vi "main_scan_5_Zeitsequenzen.vi"() -> ()   [LabVIEW 2009]
uses:
  <vilib>/userdefined/High Color/IMAQdx.ctl
  <vilib>/vision/Image Controls.llb/IMAQ Image.ctl
  global_stage_initialised.vi
  <vilib>/vision/driver/IMAQdx.llb/IMAQdx Buffer Number Mode.ctl
  <vilib>/Utility/file.llb/Write To Spreadsheet File (DBL).vi
  <vilib>/vision/driver/NI_Vision_Acquisition_Software.lvlib
  Program Files (x86)/National Instruments/LabVIEW 2009/resource/objmgr/imaqdx.rc
panel:
  in  "Log-Plot":bool
  in  "Video Mode":u32(ring)=2 items=["Mono 8 1.88 fsp", "Mono 8 3.75 fsp", "Mono 8 7.50 fsp", "Mono 8 15.00 fsp", "Mono 8 30.00 fsp", "Mono 8 60.00 fsp", "Mono 8 120.00 fsp", "Mono 16 1.88 fsp", "Mono 16 3.75 fsp", "Mono 16 7.50 fsp", "Mono 16 15.00 fsp", "Mono 16 30.00 fsp", "Mono 16 60.00 fsp", "Format 7 Mode 0 640x480"]
  out "Vektor Summierte Helligkeit [a.u.]":dbl[](array[numeric])
  out "Vektor L/2-Position [°]":dbl[](array[numeric])
  out "Daten speichern":bool
  out "Leist/Pol # Schleifen":i64
  out "Leistungs-/Polarisationscan läuft":bool
  in  "Max. Spannungsdifferenz":dbl=150.0
  out "Geschätzte Messzeit":string="00:00"
  out "Start time [ms]":timestamp
  out "2D-Intensitätsverteilung (MCP)":dbl[][](graph)
  in  "# Photosignale":i32
  in  "Achs-ID":i32
  in  "Spannungskanal":refnum<k21>
  out "x-U-Scan läuft":bool
  out "Spannungsscan läuft":bool
  out "LAPD Spannung (V)":dbl format="%#.3g"
  out "Summierte Helligkeit (a.u.)":i64
  out "# Messschritte":i32
  out "Aktueller Messschritt":i32
  in  "LAPD-Daten speichern":bool
  in  "Summierte Helligkeit speichern":bool
  in  "Einzelbilder speichern":bool
  in  "Gemittelte Bilder speichern":bool
  in  "# Bilder/Messschritt":i32=1
  in  "SN von Rotationsbühne":i32=83831982
  in  "Wellenplatte [°]":refnum<k7>(container)
  out "Wellenplatte":bool
  in  "Waveplate ON/OFF":bool
  in  "Registerkarte":T1(tab)=enum."Sequenzaufnahme"
  out "Aktuelle xyz-Position [mm]":dbl[](array[numeric]) format="%.5g"
  in  "Rasterweite [µm]":dbl[](array[numeric])
  in  "# Rasterschritte":i32[](array[numeric])=[1, 1, 1] min=1 step=1
  in  "Rasterung ON/OFF":bool
  out "Start xyz-Position [mm]":dbl[](array[numeric]) format="%.5g"
  in  "Rasterart":T2(ring)=enum."2D-Scan(xy)"
  out "Rasterschritt [µm]":dbl[](array[numeric])
  out "2D-Intensitätsverteilung (LAPD)":dbl[][](graph)
  out "Spannungsstart [V]":dbl[](array[numeric])
  out "TIP/SUP":string[](array[string])=["Tip", "Suppressor"]
  out "Spannungsschritt [V]":dbl[](array[numeric]) format="%.1g"
  out "Aktuelle Spannung [V]":dbl[](array[numeric]) format="%.1f"
  in  "# Spannungsschritte":i32[](array[numeric])
  in  "Spannungsweite [V]":dbl[](array[numeric])
  in  "Spannungsscan ON/OFF":bool
  out "Schräglage berücksichtigen":string="Schräglage berücksichtigen"
  in  "Ausgleichslage Start festlegen":bool
  out "x-U-Scan (Ausgleichslage) xy-Start [mm]":dbl[](array[numeric]) format="%_5g"
  in  "Raum-Koordinate 2 (Lagenausgleich)":enum16{"x-Achse", "y-Achse", "z-Achse"}(ring)=enum."y-Achse"
  out "x-U-Scan y-Startposition [mm]":dbl format="%.4g"
  out "x-U-Scan aktuelle y-Position [mm]":dbl format="%.4g"
  in  "x-U-Scan (Ausgleichslage) Steigung":dbl format="%_3g"
  out "x-U-Scan Spannungsstart [V]":dbl
  out "x-U-Scan Spannungsschritt [V]":dbl
  out "x-U-Scan aktuelle Spannung [V]":dbl
  in  "# x-U-Scan Spannungsschritte":i32
  in  "x-U-Scan Spannungsweite [V]":dbl
  in  "Raum-Koordinate 1":enum16{"x-Achse", "y-Achse", "z-Achse"}(ring)
  in  "Spannungs-Koordinate":enum16{"Tip-Spannung", "Suppressor-Spannung"}(ring)=2
  in  "x-U-Scan ON/OFF":bool
  in  "x-U-Scan x-Rasterweite [µm]":dbl
  in  "# x-U-Scan x-Rasterschritte":i32
  out "x-U-Scan x-Startposition [mm]":dbl format="%.4g"
  out "x-U-Scan aktuelle x-Position [mm]":dbl format="%.4g"
  out "x-U-Scan x-Rasterschritt [µm]":dbl
  out "x-U-Scan (Ausgleichslage) xy-End [mm]":dbl[](array[numeric]) format="%_5g"
  in  "Ausgleichslage Ende festlegen":bool
  in  "Sättigungszeit [s]":dbl
  in  "Wartezeit [s]":dbl
  in  "Max. Leistung (vK) [mW]":dbl
  out "Aktuelle Leistung (iK) [mW]":dbl
  out "Aktuelle L/2-Position [°]":dbl format="%_3g"
  out "L/2-Schritt [°]":dbl
  in  "Hin und Zurück":bool=TRUE
  in  "# L/2-Schritte":i32
  in  "L/2-Weite [°]":dbl
  in  "L/2-Start [°]":dbl
  in  "Leistuns- oder Polarisationsscan":u16(ring) items=["Polarisationsscan", "Leistungsscan"]
  in  "Leistungs-/Polarisationsscan ON/OFF":bool
  out "1D-Intensitätsverteilung (MCP)":T3(graph)
  out "Vorherige L/2 Position [°]":dbl format="%_3g"
  out "Gesamtzeit [min]":dbl format="%#.2g"
  in  "# Messpunkte":i32=1
  in  "Verzögerung [s]":i64
  in  "Hintergrund-Helligkeit":i64
  in  "Helligkeit nullen":bool
  out "Helligkeitsverlauf":dbl(graph)
  in  "Sequenz Ordner":string="Referenzbilder"
  in  "Sequenzaufnahme ON":bool
  out "LAPD (a.u.)":dbl(graph)
  in  "MCP-Spannung [V]":dbl=1300.0
  in  "P-Schirm-Spannung [V]":dbl=4300.0
  in  "Proben-ID":string="140528_06"
  out "Messlogbuch":path
  out "Gemitteltes Bild":u64[][](array[numeric])
  in  "Polarisation [°]":dbl=90.0
  out "Current y step":i32
  out "Current z step":i32
  out "Current x step":i32
  out "Scanschleifenzähler":i32
  out "Kameraschleifenzähler":i32
  out "Steuerschleifenzähler":i32
  out "Bühne":bool
  in  "HV ON/OFF":bool
  out "HV-Steuerung":bool
  in  "Suppressor-Spannung [V]":dbl min=0.0 max=300.0 step=1.0 format="%.1p"
  in  "Tip-Spannung [V]":dbl min=0.0 max=300.0 step=1.0 format="%.1p"
  in  "Leistung (iK) [mW]":dbl format="%.1f"
  in  "LAPD-Kanal (Meilhaus)":u32 max=31
  out "Save folder":string
  out "Buffer Number":u64
  out "ROI table":string[](array[string])=["Breite [px]", "Höhe [px]", "X-Offset [px]", "Y-Offset [px]"]
  in  "Vollbild":bool
  out "Frame Rate (FPS)":dbl format="%#_3g"
  in  "Buffer Interval":u32=1
  out "Ereignis: FrameDone?":refnum<event-registration>
  out "Image Display":T4(plugin-control)
  in  "ROI":i32[](array[numeric])=[640, 480, 0, 0]
  in  "Shutter time (ms)":u16(ring)=3 items=["1000", "500", "200", "100", "50", "20", "10", "1"]
  out "Buffer Overrun":bool
  out "Image Memory":T4
  out "Kamera":bool
  in  "Kamera ON/OFF":bool
  in  "Detektionskamera":T5="cam0"
  out "Day folder":string
  in  "Root folder":string="D:\\Michael Lohmann\\Messungen\\"
  out "z-Achse":i32=3
  out "y-Achse":i32=2
  out "x-Achse":i32=1
  out "Event: Rasterung gestartet?":refnum<user-event>
  out "Fehler (Ausgang)":errorcluster
  in  "Programm beenden":bool
  out "Rasterung läuft":bool
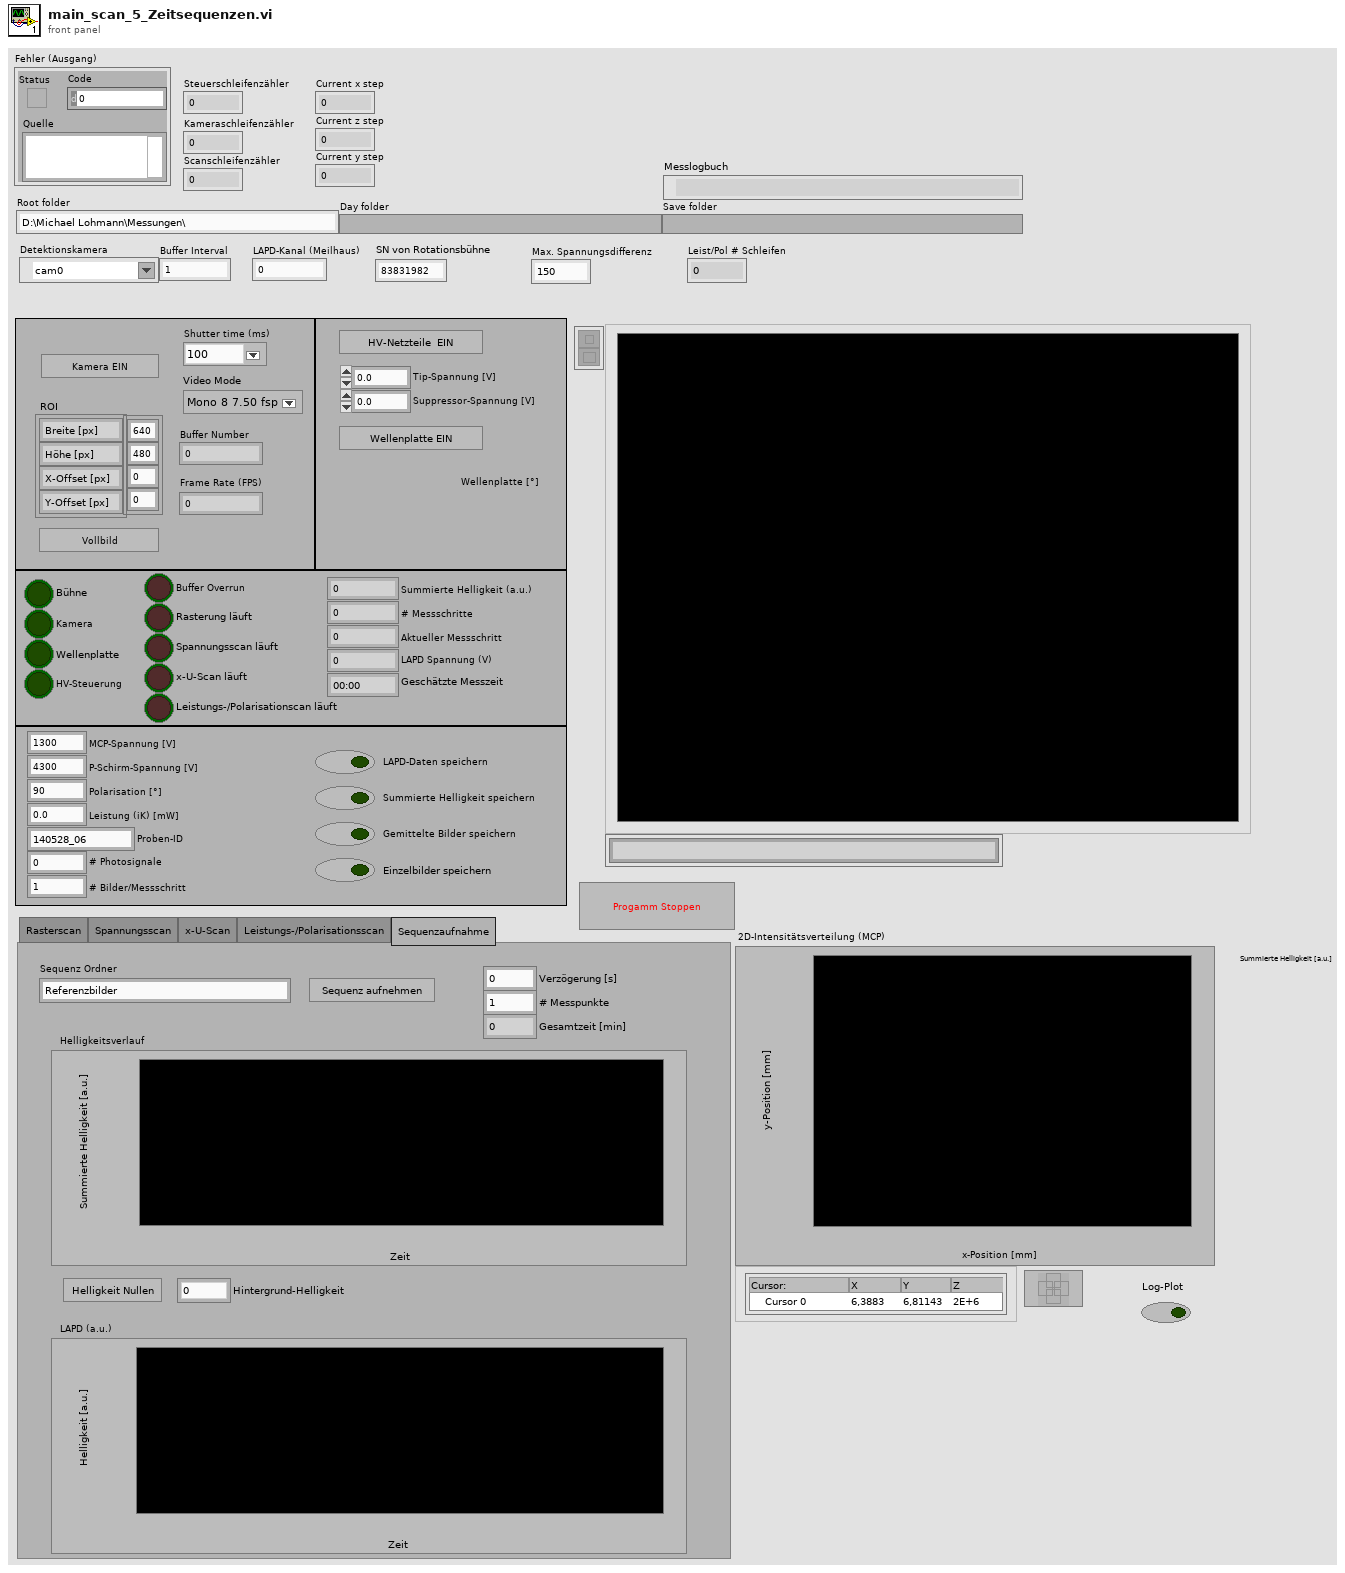
[diagram p1: front panel]
types:
  T1 = enum32{"Rasterscan", "Spannungsscan", "x-U-Scan", "Leistungs-/Polarisationsscan", "Sequenzaufnahme"}
  T2 = enum16{"Linescan(x)", "Linescan(z)", "2D-Scan(xy)", "2D-Scan(yz)", "2D-Scan(xz)"}
  T3 = cluster{"Vektor L/2-Position [°]":dbl[], "Vektor Summierte Helligkeit [a.u.]":dbl[]}
  T4 = typedef "IMAQ Image.ctl" = refnum<image>
  T5 = typedef "IMAQdx.ctl" = refnum<k21>
  T6 = enum32{"Bad", "Idle", "Run top level", "Running"}
  T7 = cluster{"Summierte Helligkeit (a.u.)":u64, "Aktuelle L/2-Position [°]":dbl}
  T8 = typedef "NI_Vision_Acquisition_Software.lvlib/IMAQdx Buffer Number Mode.ctl" = enum32{"Next", "Last", "Buffer Number"}
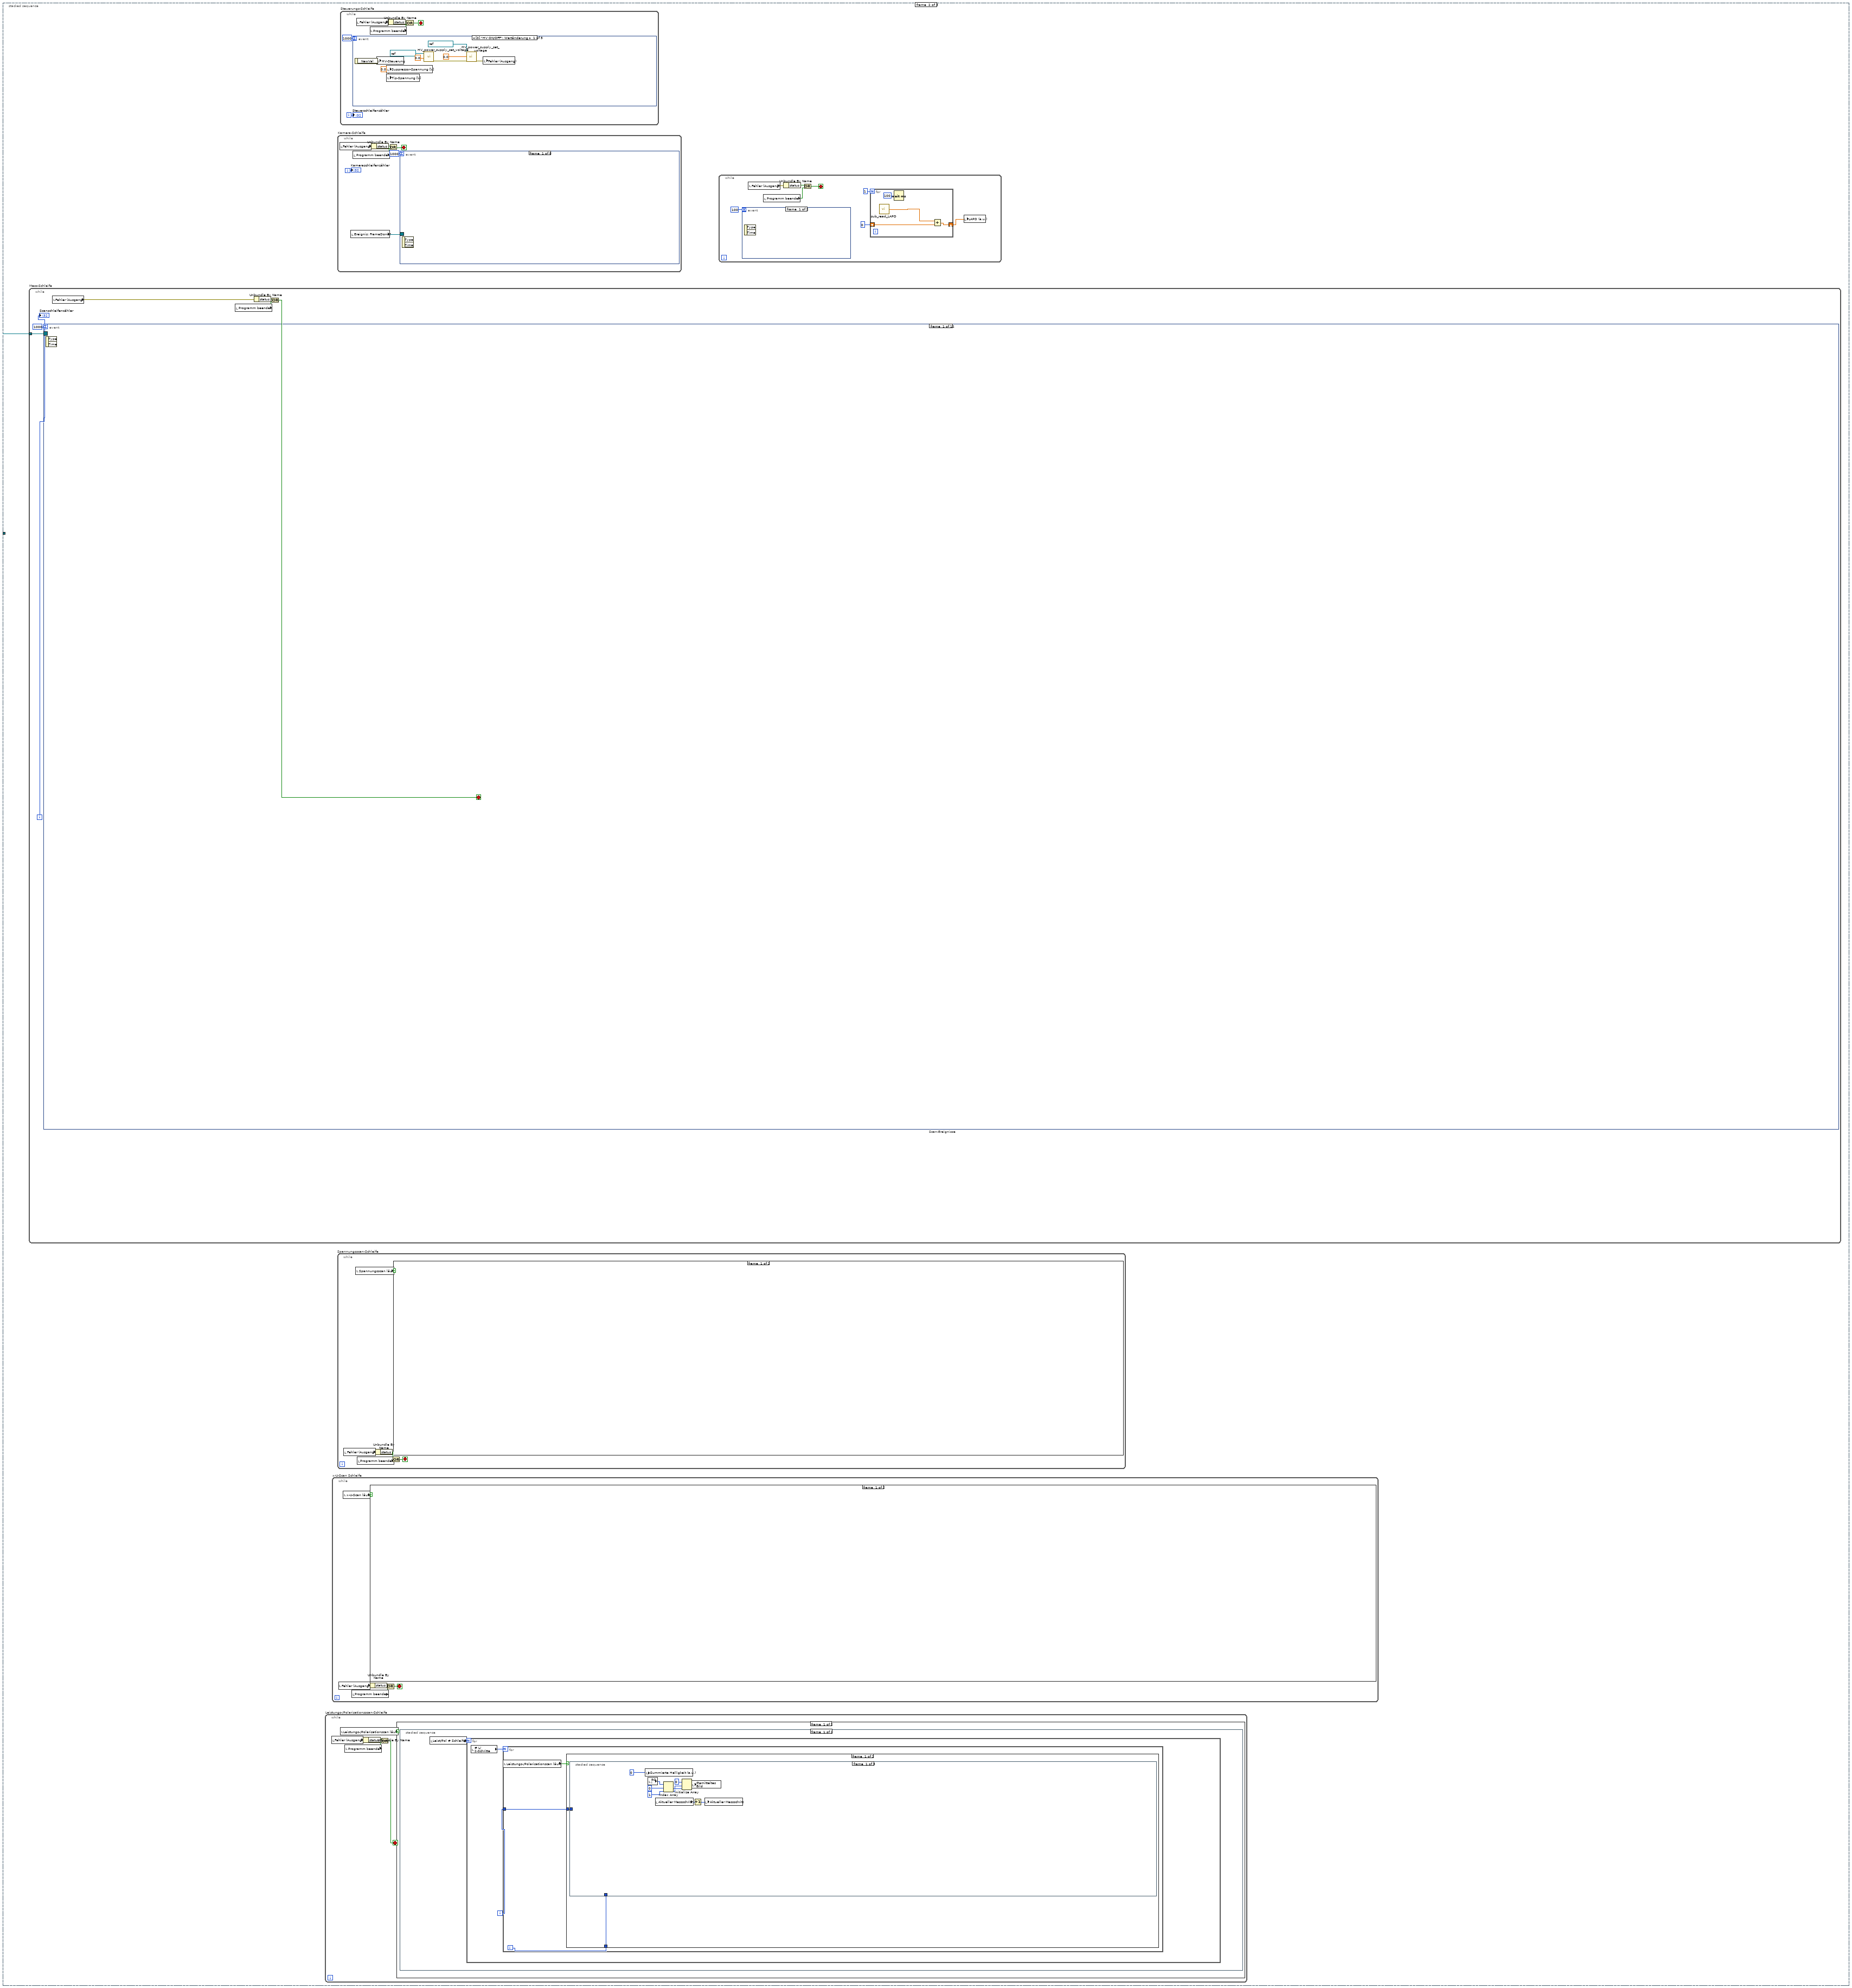
[diagram p3: hidden frame]
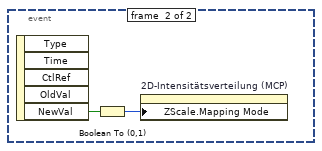
[diagram p4: hidden frame]
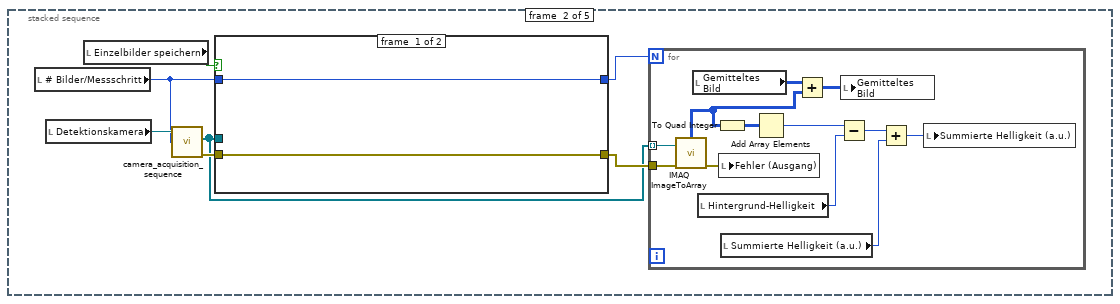
[diagram p5: hidden frame]
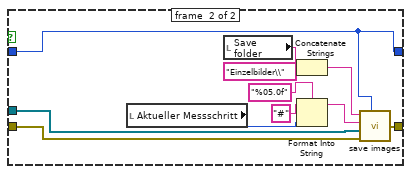
[diagram p6: hidden frame]
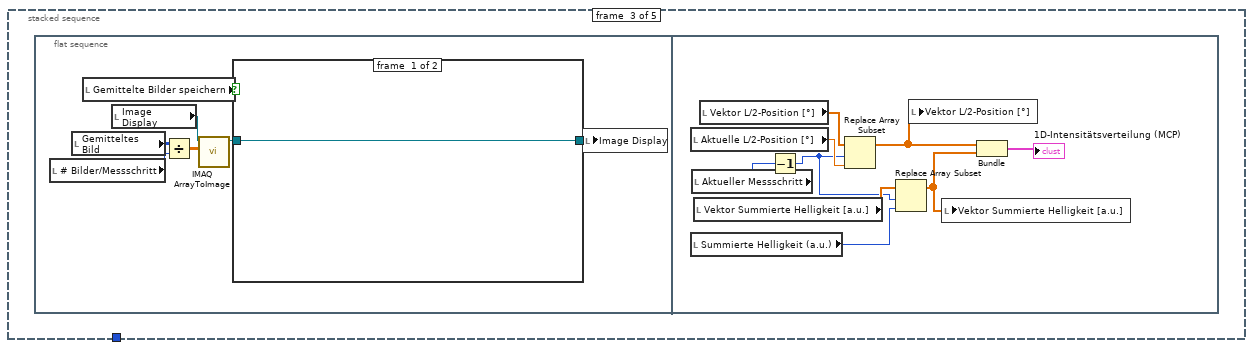
[diagram p7: hidden frame]
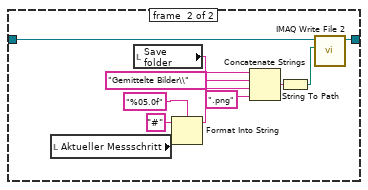
[diagram p8: hidden frame]
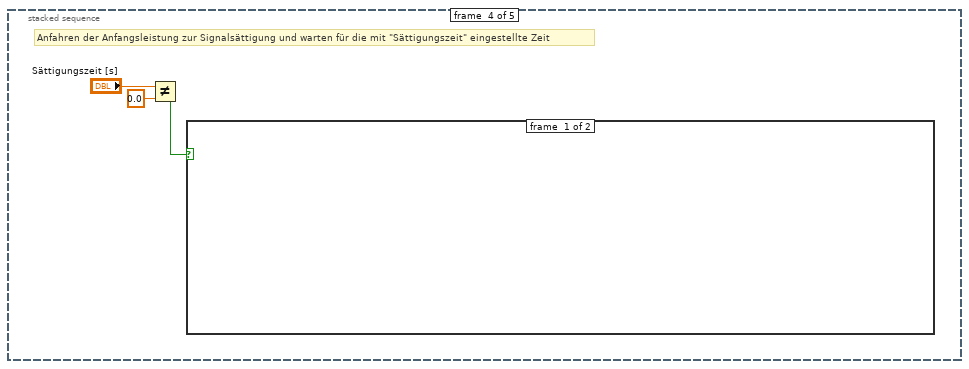
[diagram p9: hidden frame]
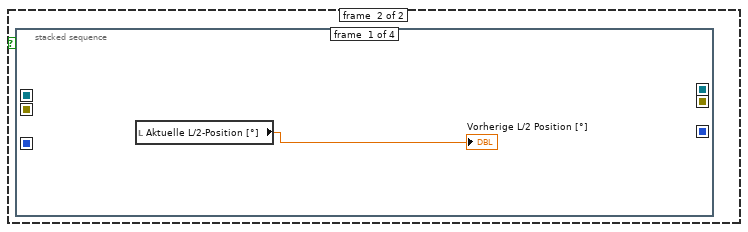
[diagram p10: hidden frame]
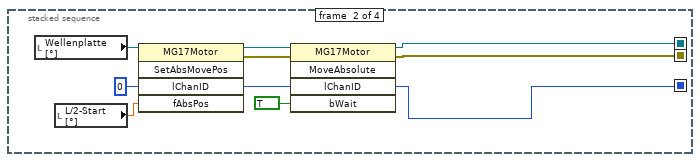
[diagram p11: hidden frame]
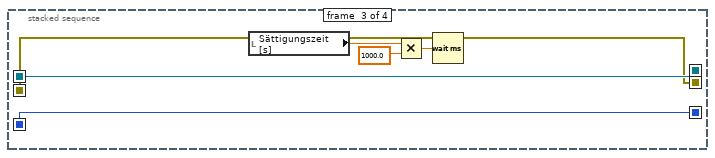
[diagram p12: hidden frame]
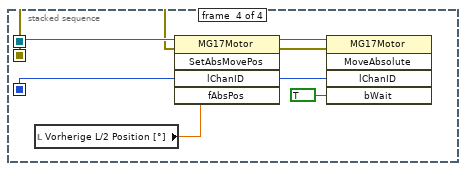
[diagram p13: hidden frame]
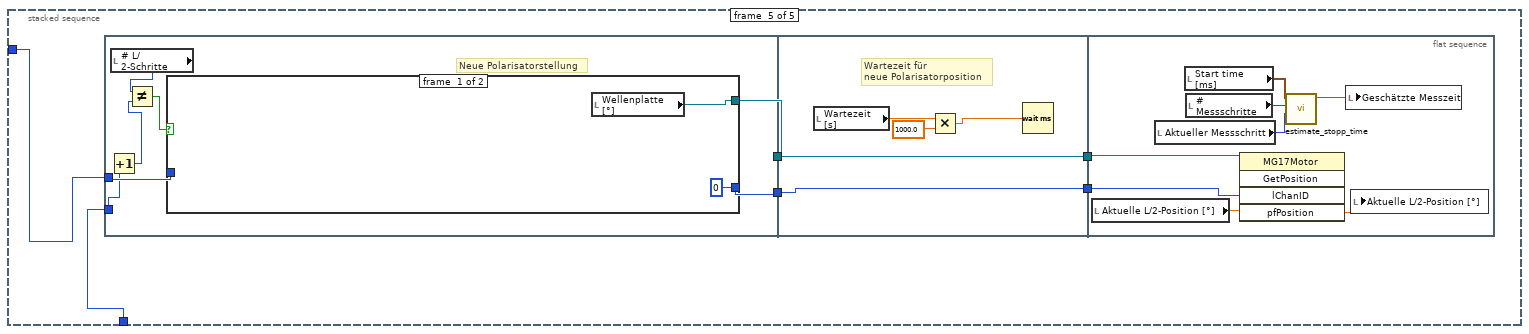
[diagram p14: hidden frame]
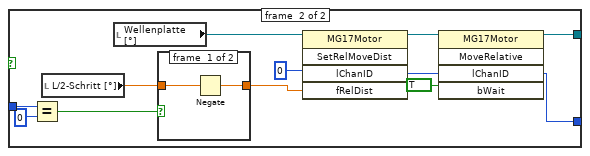
[diagram p15: hidden frame]
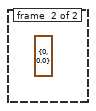
[diagram p17: hidden frame]
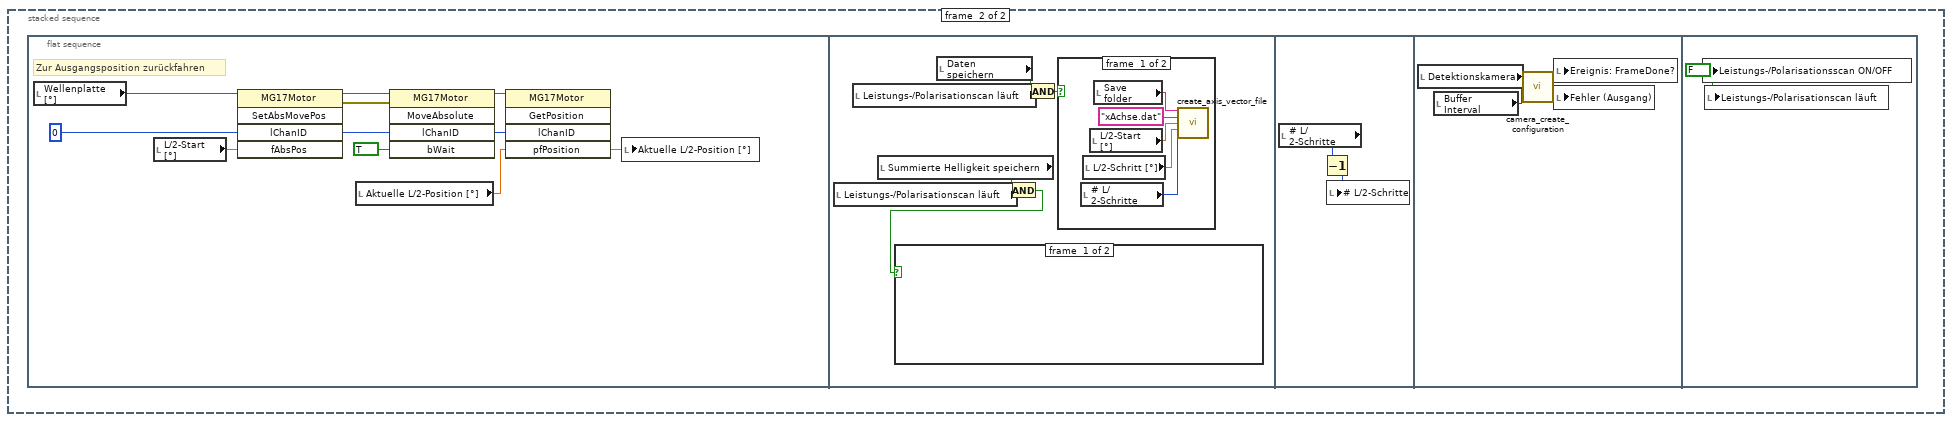
[diagram p18: hidden frame]
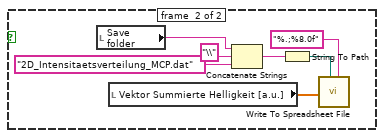
[diagram p19: hidden frame]
diagram:
  n1 = local read "Event: Rasterung gestartet?"() -> (w2:refnum<user-event>)
  n2 = register-events(w2) -> (reference out=w1:refnum<event-registration>)  [unwired: 2 in, 1 out]
  n3 = stacked-sequence {
    tunnel: w1 -> [_ w27 _]
    frame #0 {
      n4 = flat-sequence {
        frame #0 {
          # "Überprüfung ob die VI stage_control.vi ausgeführt wid, wenn nicht wird sie gestartet und gewartet bis die Bühne initialisiert ist"
          n5 = Open VI Reference(vi path=path "stage_control_mit_speichern.vi" ("VI-Pfad")) -> (vi reference=w5:refnum<vi>)  [unwired: 5 in, 1 out]
          n6 = property class="VI"(reference=w5) -> (reference out=w4:refnum<vi>, error out=w3:errorcluster, "Exec.State"=w8:T6)  [unwired: 1 in]
          n7 = Equal?(x=w8, y=T6."Run top level") -> (x = y?=w6:bool)
          n8 = case shown="False" w6 {
            tunnel: w4 -> [w15 _]
            tunnel: w3 -> [w14 _]
            frame #0 {
              n9 = invoke class="VI" method="VI ausführen"(reference=w15, error in=w14, "Wait until done"=FALSE ("Warten bis beendet"), "Auto Dispose Ref"=FALSE ("Referenz automatisch schließen")) -> (reference out=w11:refnum<vi>)  [unwired: 1 in, 4 out]
              n10 = invoke class="VI" method="FP.Öffnen"(reference=w11) -> (reference out=w10:refnum<vi>)  [unwired: 4 in, 4 out]
              n11 = while {
                tunnel: w10 -> [w22]
                stop <- w17 stop-if-true
                n12 = property class="VI"(reference=w22) -> (error out=w21:errorcluster, "Exec.State"=w20:T6)  [unwired: 1 in, 1 out]
                n13 = global read "global_stage_initialised.vi" "Bühne initialisiert"() -> (w16:bool)
                n14 = local write "Fehler (Ausgang)"(w21) -> ()
                n15 = Equal?(x=w20, y=T6."Run top level") -> (x = y?=w18:bool)
                n16 = And(x=w16, y=w18) -> (x .and. y?=w17:bool)
              }
            }
            frame #1 {
            }
          }
        }
        frame #1 {
          n17 = local read "Root folder"() -> (w26:string)
          n18 = local write "Bühne"(TRUE ("Bühne bereit")) -> ()
          n19 = call "create_day_folder.vi"("Root folder"=w26) -> ("Day Folder"=w24:string)  [unwired: 9 in, 1 out]
          n20 = local write "Day folder"(w24) -> ()
          n21 = call "create_measure_log_file.vi"("Tagesordner"=w24) -> ("Messlogbuch"=w23:path)  [unwired: 9 in]
          n22 = local write "Messlogbuch"(w23) -> ()
        }
      }
    }
    frame #1 {
      n23 = while "Mess-Schleife" {
        tunnel: w27 -> [w644]
        i -> [w643]
        stop <- w642 stop-if-true
        n24 = event "Scan-Ereignisse" shown="[3] <Event: Rasterung gestartet?>: Benutzerereignis" {
          selector: w644 -> [_ _ _ _ _ _ _ _ _ _ _]
          dyn-events: _ -> [_ _ _ _ _ _ _ _ _ _ _]
          timeout: 1000 -> [_ _ _ _ _ _ _ _ _ _ _]
          event #0 {
            n25 = event-data() -> ()  [unwired: 1 in, 2 out]
          }
          event #1 {
            n26 = event-data() -> ("NewVal"=w651:bool)  [unwired: 1 in]
            n27 = local read "Kamera"() -> (w649:bool)
            n28 = case shown="False" w649 {
              frame #0 {
                n29 = local write "Rasterung ON/OFF"(FALSE ("Rasterung ON/OFF")) -> ()
                n30 = One Button Dialog(message="Kamera aus" ("Nachricht")) -> ()  [unwired: 1 in, 1 out]
              }
              frame #1 {
              }
            }
            n31 = And(x=w649, y=w651) -> (x .and. y?=w650:bool)
            n32 = case shown="True" w650 {
              frame #0 {
                n33 = local write "Rasterung läuft"(FALSE ("Rasterung läuft")) -> ()
              }
              frame #1 {
                n34 = stacked-sequence {
                  frame #0 {
                    n35 = stacked-sequence {
                      seq-local: [w664 _] -> [_ w727]
                      frame #0 {
                        n36 = local read "Rasterart"() -> (w678:T2)
                        n37 = local read "Rasterweite [µm]"() -> (w675:dbl[])
                        n38 = local read "# Rasterschritte"() -> (w677:i32[])
                        n39 = Get Date/Time In Seconds() -> (seconds since 1Jan1904=w655:timestamp)
                        n40 = local write "Start time [ms]"(w655) -> ()
                        n41 = case shown="\"2D-Scan(xz)\"" w678 {
                          tunnel: w677 -> [w686 w702 w707 w716 w722]
                          tunnel: [w685 w701 w708 w715 w719] -> w676
                          tunnel: w675 -> [w684 w692 w704 w712 w721]
                          tunnel: [w683 w691 w703 w711 w720] -> w674
                          frame #0 {
                            n42 = Replace Array Subset(array=w686, new element #1=1 ("Neues Element/Teil-Array"), index #1=1 ("Index"), new element #2=1 ("Neues Element/Teil-Array"), index #2=2 ("Index")) -> (w685:i32[])
                            n43 = Replace Array Subset(array=w684, new element #1=0.0 ("Neues Element/Teil-Array"), index #1=1 ("Index"), new element #2=0.0 ("Neues Element/Teil-Array"), index #2=2 ("Index")) -> (w683:dbl[])
                          }
                          frame #1 {
                            n44 = Replace Array Subset(array=w702, new element #1=1 ("Neues Element/Teil-Array"), index #1=0 ("Index"), new element #2=1 ("Neues Element/Teil-Array"), index #2=1 ("Index")) -> (w701:i32[])
                            n45 = Replace Array Subset(array=w692, new element #1=0.0 ("Neues Element/Teil-Array"), index #1=0 ("Index"), new element #2=0.0 ("Neues Element/Teil-Array"), index #2=1 ("Index")) -> (w691:dbl[])
                          }
                          frame #2 {
                            n46 = Replace Array Subset(array=w707, new element=1 ("Neues Element/Teil-Array"), index=2 ("Index")) -> (w708:i32[])
                            n47 = Replace Array Subset(array=w704, new element=0.0 ("Neues Element/Teil-Array"), index=2 ("Index")) -> (w703:dbl[])
                          }
                          frame #3 {
                            n48 = Replace Array Subset(array=w716, new element=1 ("Neues Element/Teil-Array"), index=0 ("Index")) -> (w715:i32[])
                            n49 = Replace Array Subset(array=w712, new element=0.0 ("Neues Element/Teil-Array"), index=0 ("Index")) -> (w711:dbl[])
                          }
                          frame #4 {
                            n50 = Replace Array Subset(array=w722, new element=1 ("Neues Element/Teil-Array"), index=1 ("Index")) -> (w719:i32[])
                            n51 = Replace Array Subset(array=w721, new element=0.0 ("Neues Element/Teil-Array"), index=1 ("Index")) -> (w720:dbl[])
                          }
                        }
                        n52 = local write "# Rasterschritte"(w676) -> ()
                        n53 = local write "Rasterweite [µm]"(w674) -> ()
                        n54 = control-ref of="Rasterart"() -> (w673:refnum<vi>)
                        n55 = property class="Enum (strikt)"(reference=w673) -> ("RingText.Text"=w659:string)  [unwired: 1 in, 2 out]
                        n56 = control-ref of="Shutter time (ms)"() -> (w672:refnum<vi>)
                        n57 = property class="Ring (strikt)"(reference=w672) -> ("RingText.Text"=w671:string)  [unwired: 1 in, 2 out]
                        n58 = local read "# Bilder/Messschritt"() -> (w670:i32)
                        n59 = local read "Suppressor-Spannung [V]"() -> (w657:dbl)
                        n60 = local read "P-Schirm-Spannung [V]"() -> (w662:dbl)
                        n61 = local read "MCP-Spannung [V]"() -> (w661:dbl)
                        n62 = local read "Leistung (iK) [mW]"() -> (w660:dbl)
                        n63 = local read "Tip-Spannung [V]"() -> (w656:dbl)
                        n64 = Decimal String To Number(string=w671) -> (number=w668:i32)  [unwired: 2 in, 1 out]
                        n65 = local read "Polarisation [°]"() -> (w665:dbl)
                        n66 = local read "Messlogbuch"() -> (w667:path)
                        n67 = local read "Proben-ID"() -> (w666:string)
                        n68 = Multiply(x=w670, y=w668) -> (x*y=w669:i32)
                        n69 = local read "ROI"() -> (w658:i32[])
                        n70 = call "stage_get_current_xyz.vi"() -> ("Aktuelle xyz-Position OUT [mm]"=w663:dbl[])  [unwired: 3 in, 1 out]
                        n71 = call "create_measure_log_entry.vi"("Messlogbuch-Pfad"=w667, "Probe"=w666, "Polarisation [°]"=w665, "Messart"=w659, "ROI"=w658, "Messungen/Messschritt"=w670, "Maximalleistung (iK) [mW]"=w660, "Tip-Spannung [V]"=w656, "Suppressor-Spannung [V]"=w657, "Zeit/Messschritt [ms]"=w668, "MCP-Spannung [V]"=w661, "Zeit/Messung [ms]"=w669, "Phosphorschirm-Spannung [V]"=w662, "xyz [mm]"=w663) -> ("Messung Nr."=w664:i32)  [unwired: 4 in, 1 out]
                      }
                      frame #1 {
                        n72 = local read "Summierte Helligkeit speichern"() -> (w731:bool)
                        n73 = local read "Gemittelte Bilder speichern"() -> (w729:bool)
                        n74 = local read "LAPD-Daten speichern"() -> (w728:bool)
                        n75 = local read "Einzelbilder speichern"() -> (w730:bool)
                        n76 = local read "Rasterweite [µm]"() -> (w758:dbl[])
                        n77 = local read "# Rasterschritte"() -> (w757:i32[])
                        n78 = local read "# Rasterschritte"() -> (w755:i32[])
                        n79 = Divide(x=w758, y=w757) -> (x/y=w756:dbl[])
                        n80 = Compound Arithmetic op=OR(w729, w730, w731, w728) -> (w732:bool)
                        n81 = local read "Kamera"() -> (w744:bool)
                        n82 = Index Array(array=w755, index #1=0 ("Index"), index #2=1 ("Index"), index #3=2 ("Index")) -> (element #1=w752:i32, element #2=w751:i32, element #3=w750:i32)
                        n83 = local write "Rasterschritt [µm]"(w756) -> ()
                        n84 = local write "Daten speichern"(w732) -> ()
                        n85 = local read "Fehler (Ausgang)"() -> (w733:errorcluster)
                        n86 = local write "Aktueller Messschritt"(0 ("Aktueller Messschritt")) -> ()
                        n87 = Multiply(x=w752, y=w751) -> (x*y=w749:i32)
                        n88 = local read "Day folder"() -> (w738:string)
                        n89 = local read "Einzelbilder speichern"() -> (w741:bool)
                        n90 = Multiply(x=w749, y=w750) -> (x*y=w748:i32)
                        n91 = local write "# Messschritte"(w748) -> ()
                        n92 = call "create_save_folder.vi"("Day folder"=w738, "Measuring number"=w727, "Measuring folder"="Rasterung" ("Subfolder"), "error in"=w733) -> ("Save Folder"=w737:string, "Error Out"=w736:errorcluster)  [unwired: 5 in]
                        n93 = local write "Save folder"(w737) -> ()
                        n94 = case shown="True" w741 {
                          tunnel: w736 -> [w759 w761]
                          tunnel: [w759 w760] -> w735
                          frame #0 {
                          }
                          frame #1 {
                            n95 = local read "Save folder"() -> (w764:string)
                            n96 = Concatenate Strings(w764, "\\Einzelbilder" ("Subfolder")) -> (w762:string)
                            n97 = String To Path(string=w762) -> (path=w765:path)
                            n98 = call <vilib>:"Check if File or Folder Exists.vi"("error in (no error)"=w761, "path"=w765) -> ("error out"=w760:errorcluster, "file or folder exists?"=w766:bool, "dup path"=w767:path)  [unwired: 7 in]
                            n99 = case shown="False" w766 {
                              tunnel: w767 -> [w768 _]
                              frame #0 {
                                n100 = Create Folder(path (use dialog)=w768) -> ()  [unwired: 2 in, 3 out]
                              }
                              frame #1 {
                              }
                            }
                          }
                        }
                        n101 = local read "Gemittelte Bilder speichern"() -> (w742:bool)
                        n102 = case shown="True" w742 {
                          tunnel: w735 -> [w769 w771]
                          tunnel: [w769 w770] -> w734
                          frame #0 {
                          }
                          frame #1 {
                            n103 = local read "Save folder"() -> (w775:string)
                            n104 = Concatenate Strings(w775, "\\Gemittelte Bilder" ("Subfolder")) -> (w777:string)
                            n105 = String To Path(string=w777) -> (path=w774:path)
                            n106 = call <vilib>:"Check if File or Folder Exists.vi"("error in (no error)"=w771, "path"=w774) -> ("error out"=w770:errorcluster, "file or folder exists?"=w773:bool, "dup path"=w772:path)  [unwired: 7 in]
                            n107 = case shown="False" w773 {
                              tunnel: w772 -> [w778 _]
                              frame #0 {
                                n108 = Create Folder(path (use dialog)=w778) -> ()  [unwired: 2 in, 3 out]
                              }
                              frame #1 {
                              }
                            }
                          }
                        }
                        n109 = case shown="True" w744 {
                          tunnel: [w779 w781] -> w743
                          tunnel: w734 -> [w779 w780]
                          frame #0 {
                          }
                          frame #1 {
                            n110 = local read "Ereignis: FrameDone?"() -> (w782:refnum<event-registration>)
                            n111 = local read "Detektionskamera"() -> (w783:T5)
                            n112 = call "camera_release_configuration.vi"("error in"=w780, "Session In"=w783, "Ereignisregistrierung (Referenz) 2"=w782) -> ("error out"=w781:errorcluster)  [unwired: 1 out]
                          }
                        }
                        n113 = call "stage_get_current_xyz.vi"("error in"=w743) -> ("error out"=w740:errorcluster, "Aktuelle xyz-Position OUT [mm]"=w745:dbl[])  [unwired: 2 in]
                        n114 = local write "Start xyz-Position [mm]"(w745) -> ()
                        n115 = local write "Fehler (Ausgang)"(w740) -> ()
                      }
                    }
                  }
                  frame #1 {
                    n116 = flat-sequence {
                      tunnel: [w798] -> w794
                      tunnel: [w797] -> w793
                      tunnel: [w796] -> w792
                      tunnel: [w796] -> w791
                      tunnel: [w796] -> w790
                      tunnel: [w796] -> w789
                      tunnel: [w796] -> w788
                      tunnel: [w795] -> w787
                      tunnel: [w796] -> w786
                      tunnel: [w796] -> w785
                      tunnel: [w795] -> w784
                      tunnel: w794 -> [w812]
                      tunnel: w793 -> [w822]
                      tunnel: w792 -> [w821]
                      tunnel: w791 -> [w820]
                      tunnel: w790 -> [w819]
                      tunnel: w789 -> [w818]
                      tunnel: w788 -> [w817]
                      tunnel: w787 -> [w816]
                      tunnel: w786 -> [w815]
                      tunnel: w785 -> [w814]
                      tunnel: w784 -> [w813]
                      frame #0 {
                        n117 = local read "Rasterart"() -> (w799:T2)
                        n118 = case shown="\"2D-Scan(yz)\"" w799 {
                          tunnel: [0 ("Index") 2 ("Index") 0 ("Index")] -> w795
                          tunnel: [1 ("Index") 1 ("Index") 2 ("Index")] -> w796
                          tunnel: ["x-Position [mm]" ("X-Achse.Namensbeschriftung.Text") "z-Position [mm]" ("Y-Achse.Namensbeschriftung.Text") "x-Position [mm]" ("Y-Achse.Namensbeschriftung.Text")] -> w798
                          tunnel: ["y-Position [mm]" ("Y-Achse.Namensbeschriftung.Text") "y-Position [mm]" ("X-Achse.Namensbeschriftung.Text") "z-Position [mm]" ("X-Achse.Namensbeschriftung.Text")] -> w797
                          frame #0 {
                          }
                          frame #1 {
                          }
                          frame #2 {
                          }
                        }
                      }
                      frame #1 {
                        w830 = 1000.0 ("y")
                        w849 = 1000.0 ("y")
                        n119 = local read "Rasterweite [µm]"() -> (w854:dbl[])
                        n120 = local read "# Rasterschritte"() -> (w858:i32[])
                        n121 = local read "Rasterweite [µm]"() -> (w825:dbl[])
                        n122 = local read "# Rasterschritte"() -> (w847:i32[])
                        n123 = local read "Start xyz-Position [mm]"() -> (w853:dbl[])
                        n124 = Index Array(array=w854, index #1=w816, index #2=w815) -> (element #1=w850:dbl, element #2=w851:dbl)
                        n125 = Index Array(array=w858, index #1=w816, index #2=w821) -> (element #1=w856:i32, element #2=w857:i32)
                        n126 = local read "# Rasterschritte"() -> (w832:i32[])
                        n127 = Divide(x=w850, y=w849) -> (x/y=w844:dbl)
                        n128 = Divide(x=w851, y=w849) -> (x/y=w846:dbl)
                        n129 = Index Array(array=w847, index #1=w816, index #2=w820) -> (element #1=w843:i32, element #2=w845:i32)
                        n130 = Index Array(array=w825, index #1=w816, index #2=w817) -> (element #1=w829:dbl, element #2=w828:dbl)
                        n131 = Initialize Array(0.0 ("y"), w856, w857) -> (w839:dbl[][])
                        n132 = local read "Start xyz-Position [mm]"() -> (w826:dbl[])
                        n133 = control-ref of="2D-Intensitätsverteilung (MCP)"() -> (w855:refnum<vi>)
                        n134 = local write "2D-Intensitätsverteilung (LAPD)"(w839) -> ()
                        n135 = local write "2D-Intensitätsverteilung (MCP)"(w839) -> ()
                        n136 = Divide(x=w829, y=w830) -> (x/y=w835:dbl)
                        n137 = Divide(x=w828, y=w830) -> (x/y=w833:dbl)
                        n138 = Index Array(array=w853, index #1=w813, index #2=w814) -> (element #1=w852:dbl, element #2=w848:dbl)
                        n139 = Index Array(array=w832, index #1=w816, index #2=w819) -> (element #1=w836:i32, element #2=w834:i32)
                        n140 = Divide(x=w844, y=w843) -> (x/y=w842:dbl)
                        n141 = Divide(x=w846, y=w845) -> (x/y=w841:dbl)
                        n142 = property class="IntGraph (strikt)"(reference=w855, "XScale.Offset"=w852, "XScale.Multiplier"=w842, "YScale.Offset"=w848, "YScale.Multiplier"=w841, "XScale.MinorInc"=w842, "YScale.MinorInc"=w841, "XScale.NameLbl.Text"=w812, "YScale.NameLbl.Text"=w822) -> (error out=w859:errorcluster)  [unwired: 1 in, 1 out]
                        n143 = Index Array(array=w826, index #1=w816, index #2=w818) -> (element #1=w827:dbl, element #2=w831:dbl)
                        n144 = control-ref of="2D-Intensitätsverteilung (LAPD)"() -> (w823:refnum<vi>)
                        n145 = Divide(x=w835, y=w836) -> (x/y=w837:dbl)
                        n146 = Divide(x=w833, y=w834) -> (x/y=w838:dbl)
                        n147 = property class="IntGraph (strikt)"(reference=w823, error in=w859, "XScale.Offset"=w827, "XScale.Multiplier"=w837, "YScale.Offset"=w831, "YScale.Multiplier"=w838, "XScale.MinorInc"=w837, "YScale.MinorInc"=w838, "XScale.NameLbl.Text"=w812, "YScale.NameLbl.Text"=w822) -> (error out=w824:errorcluster)  [unwired: 1 out]
                        n148 = local write "Fehler (Ausgang)"(w824) -> ()
                      }
                    }
                  }
                  frame #2 {
                    n149 = flat-sequence {
                      frame #0 {
                        n150 = local read "Event: Rasterung gestartet?"() -> (w860:refnum<user-event>)
                        n151 = local read "Aktueller Messschritt"() -> (w861:i32)
                        n152 = Generate User Event(user event=w860, event data cluster=w861) -> (user event out=w862:refnum<user-event>)  [unwired: 1 in, 1 out]
                        n153 = local write "Event: Rasterung gestartet?"(w862) -> ()
                      }
                      frame #1 {
                        n154 = local write "Rasterung läuft"(TRUE ("x-Linsescan")) -> ()
                      }
                    }
                  }
                }
              }
            }
          }
          event #2 {
            n155 = event-data() -> ()  [unwired: 1 in, 1 out]
            n156 = local read "Rasterweite [µm]"() -> (w865:dbl[])
            n157 = local read "# Rasterschritte"() -> (w876:i32[])
            n158 = Replace Array Subset(array=w876, new element #1=1 ("Neues Element/Teil-Array"), index #1=0 ("Index"), new element #2=1 ("Neues Element/Teil-Array"), index #2=1 ("Index"), new element #3=1 ("Neues Element/Teil-Array"), index #3=2 ("Index")) -> (w872:i32[])
            n159 = Replace Array Subset(array=w865, new element #1=0 ("Neues Element/Teil-Array"), index #1=0 ("Index"), new element #2=0 ("Neues Element/Teil-Array"), index #2=1 ("Index"), new element #3=0 ("Neues Element/Teil-Array"), index #3=2 ("Index")) -> (w864:dbl[])
            n160 = local write "Rasterweite [µm]"(w864) -> ()
            n161 = local write "# Rasterschritte"(w872) -> ()
          }
          event #3 {
            n162 = event-data() -> ()  [unwired: 1 in, 1 out]
            n163 = stacked-sequence {
              frame #0 {
                n164 = while "x-Schleife" {
                  i -> [w882]
                  stop <- w883 stop-if-true
                  n165 = stacked-sequence {
                    frame #0 {
                      n166 = while "z-Schleife" {
                        i -> [w890]
                        stop <- w892 stop-if-true
                        n167 = stacked-sequence {
                          frame #0 {
                            n168 = while "y-Schleife" {
                              i -> [w901]
                              stop <- w907 stop-if-true
                              # "Schleife für y-Achse"
                              n169 = stacked-sequence {
                                frame #0 {
                                # "Hier findet die Messung statt"
                                n170 = stacked-sequence {
                                frame #0 {
                                n171 = local write "Summierte Helligkeit (a.u.)"(u64 0 ("Summierte Helligkeit (a.u.)")) -> ()
                                n172 = local write "LAPD Spannung (V)"(0.0 ("Transmittierte Intensität (a.u.)")) -> ()
                                n173 = local read "ROI"() -> (w914:i32[])
                                n174 = Index Array(array=w914, index #1=0 ("Index"), index #2=1 ("Index")) -> (element #1=w910:i32, element #2=w911:i32)
                                n175 = local read "Aktueller Messschritt"() -> (w917:i32)
                                n176 = Initialize Array(u64 0 ("Element"), w911, w910) -> (w916:u64[][])
                                n177 = local write "Gemitteltes Bild"(w916) -> ()
                                n178 = Increment(x=w917) -> (x+1=w918:i32)
                                n179 = local write "Aktueller Messschritt"(w918) -> ()
                                }
                                frame #1 {
                                n180 = local read "# Photosignale"() -> (w928:i32)
                                n181 = local read "# Bilder/Messschritt"() -> (w924:i32)
                                n182 = local read "Detektionskamera"() -> (w927:T5)
                                n183 = for {
                                N: w928 -> [_]
                                n184 = Wait (ms)(milliseconds to wait=u32 10 ("Zu wartende ms")) -> ()  [unwired: 1 out]
                                n185 = local read "LAPD Spannung (V)"() -> (w943:dbl)
                                n186 = call "sub_read_LAPD.vi"() -> ("data"=w942:dbl)  [unwired: 1 in]
                                n187 = Add(x=w942, y=w943) -> (x+y=w944:dbl)
                                n188 = local write "LAPD Spannung (V)"(w944) -> ()
                                }
                                n189 = local read "Einzelbilder speichern"() -> (w922:bool)
                                n190 = call "camera_acquisition_sequence.vi"("Session In"=w927, "Desired image number"=w924) -> ("Image Array"=w921:T4[], "error out"=w926:errorcluster)  [unwired: 2 in, 1 out]
                                n191 = case shown="True" w922 {
                                tunnel: w926 -> [w930 w938]
                                tunnel: [w930 w937] -> w925
                                tunnel: w924 -> [w929 w936]
                                tunnel: [w929 w936] -> w923
                                tunnel: w921 -> [_ w935]
                                frame #0 {
                                }
                                frame #1 {
                                n192 = local read "Aktueller Messschritt"() -> (w941:i32)
                                n193 = local read "Save folder"() -> (w933:string)
                                n194 = Concatenate Strings(w933, "Einzelbilder\\" ("String")) -> (w931:string)
                                n195 = Format Into String(format string="%05.0f" ("Format-String"), initial string="#" ("Eingangs-String"), w941) -> (resulting string=w934:string)  [unwired: 1 in, 1 out]
                                n196 = call "save images.vi"("Save Folder"=w931, "File name prefix"=w934, "Array"=w935, "error out 2"=w938, "Bilder/Messschritt"=w936) -> ("error out"=w937:errorcluster)
                                }
                                }
                                n197 = for {
                                N: w923 -> [_]
                                tunnel: w925 -> [w954]
                                tunnel: w921 -> [w952] mode=indexing
                                n198 = call "IMAQ ImageToArray"("error in (no error)"=w954, "Image"=w952) -> ("error out"=w953:errorcluster, "Image Pixels (U8)"=w951:u8[][])  [unwired: 2 in, 3 out]
                                n199 = local write "Fehler (Ausgang)"(w953) -> ()
                                n200 = To Quad Integer(1:w951) -> (0:w955:i64[][])
                                n201 = local read "Gemitteltes Bild"() -> (w949:u64[][])
                                n202 = Add Array Elements(numeric array=w955) -> (sum=w948:i64)
                                n203 = local read "Summierte Helligkeit (a.u.)"() -> (w956:i64)
                                n204 = Add(x=w949, y=w951) -> (x+y=w950:u64[][])
                                n205 = local write "Gemitteltes Bild"(w950) -> ()
                                n206 = local read "Hintergrund-Helligkeit"() -> (w946:i64)
                                n207 = Subtract(x=w948, y=w946) -> (x-y=w947:i64)
                                n208 = Add(x=w947, y=w956) -> (x+y=w957:i64)
                                n209 = local write "Summierte Helligkeit (a.u.)"(w957) -> ()
                                }
                                }
                                frame #2 {
                                n210 = local read "Rasterart"() -> (w967:T2)
                                n211 = case shown="\"2D-Scan(xz)\"" w967 {
                                tunnel: [w989 w990 w992 w993 w995] -> w966
                                tunnel: [w988 w991 w992 w993 w994] -> w965
                                frame #0 {
                                n212 = local read "Current y step"() -> (w988:i32)
                                n213 = local read "Current x step"() -> (w989:i32)
                                }
                                frame #1 {
                                n214 = local read "Current z step"() -> (w990:i32)
                                n215 = local read "Current y step"() -> (w991:i32)
                                }
                                frame #2 {
                                n216 = local read "Current z step"() -> (w992:i32)
                                }
                                frame #3 {
                                n217 = local read "Current x step"() -> (w993:i32)
                                }
                                frame #4 {
                                n218 = local read "Current z step"() -> (w994:i32)
                                n219 = local read "Current x step"() -> (w995:i32)
                                }
                                }
                                n220 = local read "# Bilder/Messschritt"() -> (w962:i32)
                                n221 = local read "Gemitteltes Bild"() -> (w964:u64[][])
                                n222 = local read "LAPD Spannung (V)"() -> (w973:dbl)
                                n223 = local read "# Photosignale"() -> (w972:i32)
                                n224 = local read "Image Display"() -> (w960:T4)
                                n225 = Divide(x=w964, y=w962) -> (x/y=w963:dbl[][])
                                n226 = local read "2D-Intensitätsverteilung (LAPD)"() -> (w968:dbl[][])
                                n227 = local read "2D-Intensitätsverteilung (MCP)"() -> (w969:dbl[][])
                                n228 = local read "Gemittelte Bilder speichern"() -> (w958:bool)
                                n229 = local read "Summierte Helligkeit (a.u.)"() -> (w974:i64)
                                n230 = Divide(x=w973, y=w972) -> (x/y=w970:dbl)
                                n231 = call "IMAQ ArrayToImage"("Image Pixels (U8)"=w963, "Image"=w960) -> ("Image Out"=w961:T4)  [unwired: 8 in, 1 out]
                                n232 = local write "LAPD Spannung (V)"(w970) -> ()
                                n233 = Replace Array Subset(array=w969, new element=w974, index (row)=w966, index (col)=w965) -> (w975:dbl[][])
                                n234 = Replace Array Subset(array=w968, new element=w970, index (row)=w966, index (col)=w965) -> (w971:dbl[][])
                                n235 = case shown="True" w958 {
                                tunnel: w961 -> [w976 w987]
                                tunnel: [w976 w978] -> w959
                                frame #0 {
                                }
                                frame #1 {
                                n236 = local read "Aktueller Messschritt"() -> (w982:i32)
                                n237 = local read "Save folder"() -> (w984:string)
                                n238 = Format Into String(format string="%05.0f" ("Format-String"), initial string="#" ("Eingangs-String"), w982) -> (resulting string=w981:string)  [unwired: 1 in, 1 out]
                                n239 = Concatenate Strings(w984, "Gemittelte Bilder\\" ("String"), w981, ".png" ("String")) -> (w980:string)
                                n240 = String To Path(string=w980) -> (path=w979:path)
                                n241 = call-poly "IMAQ Write File 2"("File Path"=w979, "Image"=w987) -> ("Image Out (duplicate)"=w978:T4)  [unwired: 8 in, 1 out]
                                }
                                }
                                n242 = local write "2D-Intensitätsverteilung (MCP)"(w975) -> ()
                                n243 = local write "2D-Intensitätsverteilung (LAPD)"(w971) -> ()
                                n244 = local write "Image Display"(w959) -> ()
                                }
                                }
                                }
                                frame #1 {
                                n245 = local read "y-Achse"() -> (w1001:i32)
                                n246 = local read "Aktueller Messschritt"() -> (w998:i32)
                                n247 = local read "Rasterschritt [µm]"() -> (w1005:dbl[])
                                n248 = local read "Start time [ms]"() -> (w999:timestamp)
                                n249 = local read "# Messschritte"() -> (w997:i32)
                                n250 = Decrement(x=w1001) -> (x-1=w1004:i32)
                                n251 = Index Array(array=w1005, index=w1004) -> (element=w1000:dbl)
                                n252 = call "estimate_stopp_time.vi"("Aktueller Messschritt"=w998, "# Messschritte"=w997, "Startzeit"=w999) -> ("Stopp Zeit"=w996:string)  [unwired: 8 in]
                                n253 = local write "Geschätzte Messzeit"(w996) -> ()
                                n254 = Not Equal?(x=w1000, y=0.0) -> (x != y?=w1002:bool)
                                n255 = case shown="True" w1002 {
                                tunnel: w1001 -> [_ w1007]
                                tunnel: w1000 -> [_ w1006]
                                frame #0 {
                                }
                                frame #1 {
                                # "Fahre nächste y-Position an"
                                n256 = call "stage_move_axis_relative.vi"("Achse"=w1007, "Schrittweite [µm]"=w1006) -> ("error out"=w1009:errorcluster, "xyz-Position OUT [mm]"=w1008:dbl[])  [unwired: 1 in, 1 out]
                                n257 = local write "Aktuelle xyz-Position [mm]"(w1008) -> ()
                                n258 = local write "Fehler (Ausgang)"(w1009) -> ()
                                }
                                }
                                }
                              }
                              n259 = local read "y-Achse"() -> (w900:i32)
                              n260 = local read "# Rasterschritte"() -> (w906:i32[])
                              n261 = Decrement(x=w900) -> (x-1=w902:i32)
                              n262 = local read "Rasterung ON/OFF"() -> (w908:bool)
                              n263 = Increment(x=w901) -> (x+1=w903:i32)
                              n264 = Index Array(array=w906, index=w902) -> (element=w905:i32)
                              n265 = Equal?(x=w905, y=w903) -> (x = y?=w904:bool)
                              n266 = Not(x=w908) -> (.not. x?=w909:bool)
                              n267 = Or(x=w904, y=w909) -> (x .or. y?=w907:bool)
                              "Current y step" <- w901
                            }
                          }
                          frame #1 {
                            n268 = flat-sequence {
                              frame #0 {
                                n269 = local read "Rasterschritt [µm]"() -> (w1016:dbl[])
                                n270 = local read "y-Achse"() -> (w1011:i32)
                                n271 = Decrement(x=w1011) -> (x-1=w1015:i32)
                                n272 = local read "Start xyz-Position [mm]"() -> (w1010:dbl[])
                                n273 = Index Array(array=w1016, index=w1015) -> (element=w1014:dbl)
                                n274 = Not Equal?(x=w1014, y=0.0) -> (x != y?=w1012:bool)
                                n275 = case shown="True" w1012 {
                                tunnel: w1011 -> [_ w1018]
                                tunnel: w1010 -> [_ w1017]
                                frame #0 {
                                }
                                frame #1 {
                                # "Fahre Startposition für y an"
                                n276 = call "stage_move_axis_absolute.vi"("Ziel xyz IN [mm]"=w1017, "Achse"=w1018) -> ("error out"=w1020:errorcluster, "Ziel xyz OUT [mm]"=w1019:dbl[])  [unwired: 1 in, 1 out]
                                n277 = local write "Aktuelle xyz-Position [mm]"(w1019) -> ()
                                n278 = local write "Fehler (Ausgang)"(w1020) -> ()
                                }
                                }
                              }
                              frame #1 {
                                n279 = local read "Rasterschritt [µm]"() -> (w1026:dbl[])
                                n280 = local read "z-Achse"() -> (w1021:i32)
                                n281 = Decrement(x=w1021) -> (x-1=w1022:i32)
                                n282 = Index Array(array=w1026, index=w1022) -> (element=w1023:dbl)
                                n283 = Not Equal?(x=w1023, y=0.0) -> (x != y?=w1024:bool)
                                n284 = case shown="True" w1024 {
                                tunnel: w1023 -> [_ w1028]
                                tunnel: w1021 -> [_ w1027]
                                frame #0 {
                                }
                                frame #1 {
                                # "Fahre nächste Position für z an"
                                n285 = call "stage_move_axis_relative.vi"("Achse"=w1027, "Schrittweite [µm]"=w1028) -> ("error out"=w1029:errorcluster, "xyz-Position OUT [mm]"=w1030:dbl[])  [unwired: 1 in, 1 out]
                                n286 = local write "Aktuelle xyz-Position [mm]"(w1030) -> ()
                                n287 = local write "Fehler (Ausgang)"(w1029) -> ()
                                }
                                }
                              }
                            }
                          }
                        }
                        n288 = local read "z-Achse"() -> (w891:i32)
                        n289 = local read "# Rasterschritte"() -> (w895:i32[])
                        n290 = Decrement(x=w891) -> (x-1=w899:i32)
                        n291 = local read "Rasterung ON/OFF"() -> (w894:bool)
                        n292 = Increment(x=w890) -> (x+1=w898:i32)
                        n293 = Index Array(array=w895, index=w899) -> (element=w896:i32)
                        n294 = Equal?(x=w896, y=w898) -> (x = y?=w897:bool)
                        n295 = Not(x=w894) -> (.not. x?=w893:bool)
                        n296 = Or(x=w897, y=w893) -> (x .or. y?=w892:bool)
                        "Current z step" <- w890
                      }
                    }
                    frame #1 {
                      n297 = flat-sequence {
                        frame #0 {
                          n298 = local read "z-Achse"() -> (w1031:i32)
                          n299 = local read "Rasterschritt [µm]"() -> (w1034:dbl[])
                          n300 = Decrement(x=w1031) -> (x-1=w1035:i32)
                          n301 = local read "Start xyz-Position [mm]"() -> (w1032:dbl[])
                          n302 = Index Array(array=w1034, index=w1035) -> (element=w1036:dbl)
                          n303 = Not Equal?(x=w1036, y=0.0) -> (x != y?=w1033:bool)
                          n304 = case shown="True" w1033 {
                            tunnel: w1032 -> [_ w1039]
                            tunnel: w1031 -> [_ w1038]
                            frame #0 {
                            }
                            frame #1 {
                              # "Fahre Startposition für z an"
                              n305 = call "stage_move_axis_absolute.vi"("Ziel xyz IN [mm]"=w1039, "Achse"=w1038) -> ("error out"=w1040:errorcluster, "Ziel xyz OUT [mm]"=w1041:dbl[])  [unwired: 1 in, 1 out]
                              n306 = local write "Aktuelle xyz-Position [mm]"(w1041) -> ()
                              n307 = local write "Fehler (Ausgang)"(w1040) -> ()
                            }
                          }
                        }
                        frame #1 {
                          n308 = local read "Rasterschritt [µm]"() -> (w1047:dbl[])
                          n309 = local read "x-Achse"() -> (w1042:i32)
                          n310 = Decrement(x=w1042) -> (x-1=w1046:i32)
                          n311 = Index Array(array=w1047, index=w1046) -> (element=w1045:dbl)
                          n312 = Not Equal?(x=w1045, y=0.0) -> (x != y?=w1043:bool)
                          n313 = case shown="True" w1043 {
                            tunnel: w1045 -> [_ w1050]
                            tunnel: w1042 -> [_ w1048]
                            frame #0 {
                            }
                            frame #1 {
                              # "Fahre nächste Position für x an"
                              n314 = call "stage_move_axis_relative.vi"("Achse"=w1048, "Schrittweite [µm]"=w1050) -> ("error out"=w1051:errorcluster, "xyz-Position OUT [mm]"=w1049:dbl[])  [unwired: 1 in, 1 out]
                              n315 = local write "Aktuelle xyz-Position [mm]"(w1049) -> ()
                              n316 = local write "Fehler (Ausgang)"(w1051) -> ()
                            }
                          }
                        }
                      }
                    }
                  }
                  n317 = local read "# Rasterschritte"() -> (w880:i32[])
                  n318 = local read "x-Achse"() -> (w881:i32)
                  n319 = Decrement(x=w881) -> (x-1=w884:i32)
                  n320 = local read "Rasterung ON/OFF"() -> (w888:bool)
                  n321 = Increment(x=w882) -> (x+1=w885:i32)
                  n322 = Index Array(array=w880, index=w884) -> (element=w887:i32)
                  n323 = Equal?(x=w887, y=w885) -> (x = y?=w886:bool)
                  n324 = Not(x=w888) -> (.not. x?=w889:bool)
                  n325 = Or(x=w886, y=w889) -> (x .or. y?=w883:bool)
                  "Current x step" <- w882
                }
              }
              frame #1 {
                n326 = flat-sequence {
                  frame #0 {
                    # "Zur Ausgangsposition zurückfahren"
                    n327 = local read "Start xyz-Position [mm]"() -> (w1142:dbl[])
                    n328 = local read "Detektionskamera"() -> (w1132:T5)
                    n329 = local read "Buffer Interval"() -> (w1131:u32)
                    n330 = call "camera_create_configuration.vi"("BufferInterval"=w1131, "Session Out 2"=w1132) -> ("Fehler (Ausgang)"=w1130:errorcluster, "Ereignisregistrierung (Referenz)"=w1133:refnum<event-registration>)  [unwired: 1 in, 1 out]
                    n331 = local write "Ereignis: FrameDone?"(w1133) -> ()
                    n332 = local read "x-Achse"() -> (w1139:i32)
                    n333 = call "stage_move_axis_absolute.vi"("error in"=w1130, "Ziel xyz IN [mm]"=w1142, "Achse"=w1139) -> ("error out"=w1135:errorcluster)  [unwired: 2 out]
                    n334 = local read "y-Achse"() -> (w1140:i32)
                    n335 = call "stage_move_axis_absolute.vi"("error in"=w1135, "Ziel xyz IN [mm]"=w1142, "Achse"=w1140) -> ("error out"=w1136:errorcluster)  [unwired: 2 out]
                    n336 = local read "z-Achse"() -> (w1141:i32)
                    n337 = call "stage_move_axis_absolute.vi"("error in"=w1136, "Ziel xyz IN [mm]"=w1142, "Achse"=w1141) -> ("error out"=w1137:errorcluster, "Fertig?"=w1138:bool, "Ziel xyz OUT [mm]"=w1143:dbl[])
                    n338 = local write "Aktuelle xyz-Position [mm]"(w1143) -> ()
                    n339 = local write "Fehler (Ausgang)"(w1137) -> ()
                    n340 = Not(x=w1138) -> (.not. x?=w1134:bool)
                    n341 = local write "Rasterung ON/OFF"(w1134) -> ()
                    n342 = local write "Rasterung läuft"(w1134) -> ()
                  }
                }
                n343 = local read "Daten speichern"() -> (w1052:bool)
                n344 = local read "LAPD-Daten speichern"() -> (w1061:bool)
                n345 = local read "2D-Intensitätsverteilung (MCP)"() -> (w1060:dbl[][])
                n346 = local read "Summierte Helligkeit speichern"() -> (w1062:bool)
                n347 = case shown="True" w1052 {
                  frame #0 {
                  }
                  frame #1 {
                    n348 = local read "Rasterschritt [µm]"() -> (w1064:dbl[])
                    n349 = Divide(x=w1064, y=1000) -> (x/y=w1065:dbl[])
                    n350 = local read "Start xyz-Position [mm]"() -> (w1067:dbl[])
                    n351 = local read "# Rasterschritte"() -> (w1068:i32[])
                    n352 = local read "Save folder"() -> (w1066:string)
                    n353 = local read "Rasterart"() -> (w1069:T2)
                    n354 = case shown="\"2D-Scan(xz)\"" w1069 {
                      tunnel: w1068 -> [w1072 w1079 w1091 w1112 w1122]
                      tunnel: w1067 -> [w1070 w1081 w1089 w1113 w1124]
                      tunnel: w1066 -> [w1073 w1082 w1088 w1111 w1125]
                      tunnel: w1065 -> [w1071 w1080 w1090 w1102 w1123]
                      frame #0 {
                        w1078 = 0 ("Index")
                        n355 = Index Array(array=w1070, index=w1078) -> (element=w1076:dbl)
                        n356 = Index Array(array=w1071, index=w1078) -> (element=w1074:dbl)
                        n357 = Index Array(array=w1072, index=w1078) -> (element=w1075:i32)
                        n358 = call "create_axis_vector_file.vi"("Save folder"=w1073, "Dateiname"="xAchse.dat", "Start"=w1076, "Schrittlänge"=w1074, "# Schritte"=w1075) -> ()  [unwired: 11 in]
                      }
                      frame #1 {
                        w1087 = 2 ("Index")
                        n359 = Index Array(array=w1081, index=w1087) -> (element=w1085:dbl)
                        n360 = Index Array(array=w1080, index=w1087) -> (element=w1083:dbl)
                        n361 = Index Array(array=w1079, index=w1087) -> (element=w1084:i32)
                        n362 = call "create_axis_vector_file.vi"("Save folder"=w1082, "Dateiname"="xAchse.dat", "Start"=w1085, "Schrittlänge"=w1083, "# Schritte"=w1084) -> ()  [unwired: 11 in]
                      }
                      frame #2 {
                        w1100 = 1 ("Index")
                        w1101 = 0 ("Index")
                        n363 = Index Array(array=w1089, index #1=w1101, index #2=w1100) -> (element #1=w1097:dbl, element #2=w1094:dbl)
                        n364 = Index Array(array=w1090, index #1=w1101, index #2=w1100) -> (element #1=w1095:dbl, element #2=w1093:dbl)
                        n365 = Index Array(array=w1091, index #1=w1101, index #2=w1100) -> (element #1=w1096:i32, element #2=w1092:i32)
                        n366 = call "create_axis_vector_file.vi"("Save folder"=w1088, "Dateiname"="xAchse.dat", "Start"=w1097, "Schrittlänge"=w1095, "# Schritte"=w1096) -> ()  [unwired: 11 in]
                        n367 = call "create_axis_vector_file.vi"("Save folder"=w1088, "Dateiname"="yAchse.dat", "Start"=w1094, "Schrittlänge"=w1093, "# Schritte"=w1092) -> ()  [unwired: 11 in]
                      }
                      frame #3 {
                        w1114 = 2 ("Index")
                        w1115 = 1 ("Index")
                        n368 = Index Array(array=w1113, index #1=w1115, index #2=w1114) -> (element #1=w1108:dbl, element #2=w1105:dbl)
                        n369 = Index Array(array=w1102, index #1=w1115, index #2=w1114) -> (element #1=w1106:dbl, element #2=w1104:dbl)
                        n370 = Index Array(array=w1112, index #1=w1115, index #2=w1114) -> (element #1=w1107:i32, element #2=w1103:i32)
                        n371 = call "create_axis_vector_file.vi"("Save folder"=w1111, "Dateiname"="yAchse.dat", "Start"=w1108, "Schrittlänge"=w1106, "# Schritte"=w1107) -> ()  [unwired: 11 in]
                        n372 = call "create_axis_vector_file.vi"("Save folder"=w1111, "Dateiname"="xAchse.dat", "Start"=w1105, "Schrittlänge"=w1104, "# Schritte"=w1103) -> ()  [unwired: 11 in]
                      }
                      frame #4 {
                        w1128 = 2 ("Index")
                        w1129 = 0 ("Index")
                        n373 = Index Array(array=w1124, index #1=w1129, index #2=w1128) -> (element #1=w1121:dbl, element #2=w1116:dbl)
                        n374 = Index Array(array=w1123, index #1=w1129, index #2=w1128) -> (element #1=w1120:dbl, element #2=w1117:dbl)
                        n375 = Index Array(array=w1122, index #1=w1129, index #2=w1128) -> (element #1=w1119:i32, element #2=w1118:i32)
                        n376 = call "create_axis_vector_file.vi"("Save folder"=w1125, "Dateiname"="xAchse.dat", "Start"=w1121, "Schrittlänge"=w1120, "# Schritte"=w1119) -> ()  [unwired: 11 in]
                        n377 = call "create_axis_vector_file.vi"("Save folder"=w1125, "Dateiname"="yAchse.dat", "Start"=w1116, "Schrittlänge"=w1117, "# Schritte"=w1118) -> ()  [unwired: 11 in]
                      }
                    }
                  }
                }
                n378 = local read "2D-Intensitätsverteilung (LAPD)"() -> (w1056:dbl[][])
                n379 = control-ref of="2D-Intensitätsverteilung (MCP)"() -> (w1059:refnum<vi>)
                n380 = case shown="True" w1061 {
                  frame #0 {
                  }
                  frame #1 {
                    n381 = local read "Save folder"() -> (w1148:string)
                    n382 = Concatenate Strings(w1148, "\\" ("String"), "2D_Intensitaetsverteilung_LAPD.dat" ("String")) -> (w1150:string)
                    n383 = local read "2D-Intensitätsverteilung (LAPD)"() -> (w1146:dbl[][])
                    n384 = String To Path(string=w1150) -> (path=w1149:path)
                    n385 = call-poly <vilib>:"Write To Spreadsheet File.vi"("format (%.3f)"="%.;%.5f", "2D data"=w1146, "file path (dialog if empty)"=w1149) -> ()  [unwired: 5 in, 1 out]
                  }
                }
                n386 = case shown="True" w1062 {
                  frame #0 {
                  }
                  frame #1 {
                    n387 = local read "Save folder"() -> (w1154:string)
                    n388 = Concatenate Strings(w1154, "\\" ("String"), "2D_Intensitaetsverteilung_MCP.dat" ("String")) -> (w1152:string)
                    n389 = local read "2D-Intensitätsverteilung (MCP)"() -> (w1156:dbl[][])
                    n390 = String To Path(string=w1152) -> (path=w1153:path)
                    n391 = call-poly <vilib>:"Write To Spreadsheet File.vi"("format (%.3f)"="%.;%8.0f", "2D data"=w1156, "file path (dialog if empty)"=w1153) -> ()  [unwired: 5 in, 1 out]
                  }
                }
                n392 = Array Max & Min(array=w1060) -> (max value=w1058:dbl, min value=w1057:dbl)  [unwired: 2 out]
                n393 = control-ref of="2D-Intensitätsverteilung (LAPD)"() -> (w1053:refnum<vi>)
                n394 = property class="IntGraph (strikt)"(reference=w1059, "ZScale.Maximum"=w1058, "ZScale.Minimum"=w1057) -> ()  [unwired: 1 in, 2 out]
                n395 = Array Max & Min(array=w1056) -> (max value=w1055:dbl, min value=w1054:dbl)  [unwired: 2 out]
                n396 = property class="IntGraph (strikt)"(reference=w1053, "ZScale.Maximum"=w1055, "ZScale.Minimum"=w1054) -> ()  [unwired: 1 in, 2 out]
              }
            }
          }
          event #4 {
            n397 = event-data() -> ("NewVal"=w1159:bool)  [unwired: 1 in, 3 out]
            n398 = local read "Wellenplatte"() -> (w1160:bool)
            n399 = local read "Kamera"() -> (w1161:bool)
            n400 = Compound Arithmetic op=AND(w1161, w1159, w1160) -> (w1158:bool)
            n401 = case shown="True" w1158 {
              frame #0 {
                n402 = local write "Leistungs-/Polarisationscan läuft"(FALSE ("Messung läuft")) -> ()
              }
              frame #1 {
                n403 = stacked-sequence {
                  frame #0 {
                    n404 = flat-sequence {
                      tunnel: [w1187] -> w1166
                      tunnel: [w1179] -> w1164
                      tunnel: w1166 -> [w1216]
                      tunnel: [w1216] -> w1165
                      tunnel: w1164 -> [w1215]
                      tunnel: [w1215] -> w1163
                      tunnel: w1165 -> [w1223]
                      tunnel: w1163 -> [w1222]
                      frame #0 {
                        n405 = local read "Hin und Zurück"() -> (w1173:bool)
                        n406 = local read "# L/2-Schritte"() -> (w1172:i32)
                        n407 = Get Date/Time In Seconds() -> (seconds since 1Jan1904=w1182:timestamp)
                        n408 = local read "L/2-Weite [°]"() -> (w1177:dbl)
                        n409 = local write "Aktueller Messschritt"(0 ("Aktueller Messschritt")) -> ()
                        n410 = local write "Start time [ms]"(w1182) -> ()
                        n411 = local read "Leistuns- oder Polarisationsscan"() -> (w1180:u16)
                        n412 = Divide(x=w1177, y=w1172) -> (x/y=w1176:dbl)
                        n413 = case shown="False" w1173 {
                          tunnel: w1172 -> [w1199 w1204]
                          tunnel: [w1197 w1202] -> w1167
                          frame #0 {
                            n414 = local write "Leist/Pol # Schleifen"(i64 1 ("Leist/Pol # Schleifen")) -> ()
                            n415 = Increment(x=w1199) -> (x+1=w1197:i32)
                          }
                          frame #1 {
                            n416 = local write "Leist/Pol # Schleifen"(i64 2 ("Leist/Pol # Schleifen")) -> ()
                            n417 = Increment(x=w1204) -> (x+1=w1200:i32)
                            n418 = Multiply(x=w1200, y=2) -> (x*y=w1202:i32)
                          }
                        }
                        n419 = local write "L/2-Schritt [°]"(w1176) -> ()
                        n420 = local read "L/2-Start [°]"() -> (w1174:dbl)
                        n421 = case shown="1" w1180 {
                          tunnel: ["Polarisationsscan" ("Subfolder") "Leistungsscan" ("Subfolder")] -> w1179
                          tunnel: [w1205 w1211] -> w1178
                          tunnel: [w1206 w1208] -> w1175
                          tunnel: w1174 -> [w1205 w1210]
                          frame #0 {
                            n422 = local read "Leistung (iK) [mW]"() -> (w1206:dbl)
                          }
                          frame #1 {
                            n423 = local read "Max. Leistung (vK) [mW]"() -> (w1209:dbl)
                            n424 = local read "Polarisation [°]"() -> (w1211:dbl)
                            n425 = call "calculate_power_in_chamber.vi"("Aktuelle L/2 Position [°]"=w1210, "Eingestellte Polarisation [°]"=w1211, "Max. Leistung (vK) [mW]"=w1209) -> ("Aktuelle Leistung (iK) [mW]"=w1208:dbl)  [unwired: 8 in]
                            n426 = local write "Leistung (iK) [mW]"(w1208) -> ()
                          }
                        }
                        n427 = local write "# Messschritte"(w1167) -> ()
                        n428 = Initialize Array(0.0 ("Element"), w1167) -> (w1171:dbl[])
                        n429 = Initialize Array(0.0 ("Element"), w1167) -> (w1170:dbl[])
                        n430 = local write "Vektor Summierte Helligkeit [a.u.]"(w1171) -> ()
                        n431 = local write "Vektor L/2-Position [°]"(w1170) -> ()
                        n432 = control-ref of="Shutter time (ms)"() -> (w1196:refnum<vi>)
                        n433 = property class="Ring (strikt)"(reference=w1196) -> ("RingText.Text"=w1195:string)  [unwired: 1 in, 2 out]
                        n434 = local read "# Bilder/Messschritt"() -> (w1188:i32)
                        n435 = local read "Suppressor-Spannung [V]"() -> (w1184:dbl)
                        n436 = local read "P-Schirm-Spannung [V]"() -> (w1186:dbl)
                        n437 = local read "MCP-Spannung [V]"() -> (w1185:dbl)
                        n438 = local read "Tip-Spannung [V]"() -> (w1183:dbl)
                        n439 = local read "Messlogbuch"() -> (w1193:path)
                        n440 = call "stage_get_current_xyz.vi"() -> ("Aktuelle xyz-Position OUT [mm]"=w1181:dbl[])  [unwired: 3 in, 1 out]
                        n441 = Decimal String To Number(string=w1195) -> (number=w1189:i32)  [unwired: 2 in, 1 out]
                        n442 = local read "Proben-ID"() -> (w1192:string)
                        n443 = local write "Start xyz-Position [mm]"(w1181) -> ()
                        n444 = Multiply(x=w1188, y=w1189) -> (x*y=w1190:i32)
                        n445 = local read "ROI"() -> (w1191:i32[])
                        n446 = call "create_measure_log_entry.vi"("Messlogbuch-Pfad"=w1193, "Probe"=w1192, "Polarisation [°]"=w1178, "Messart"=w1179, "ROI"=w1191, "Messungen/Messschritt"=w1188, "Maximalleistung (iK) [mW]"=w1175, "Tip-Spannung [V]"=w1183, "Suppressor-Spannung [V]"=w1184, "Zeit/Messschritt [ms]"=w1189, "MCP-Spannung [V]"=w1185, "Zeit/Messung [ms]"=w1190, "Phosphorschirm-Spannung [V]"=w1186, "xyz [mm]"=w1181) -> ("Messung Nr."=w1187:i32)  [unwired: 4 in, 1 out]
                      }
                      frame #1 {
                        n447 = local read "# L/2-Schritte"() -> (w1214:i32)
                        n448 = Increment(x=w1214) -> (x+1=w1213:i32)
                        n449 = local write "# L/2-Schritte"(w1213) -> ()
                      }
                      frame #2 {
                        n450 = local read "Fehler (Ausgang)"() -> (w1225:errorcluster)
                        n451 = local read "Summierte Helligkeit speichern"() -> (w1218:bool)
                        n452 = local read "Einzelbilder speichern"() -> (w1231:bool)
                        n453 = local read "Gemittelte Bilder speichern"() -> (w1220:bool)
                        n454 = local read "Day folder"() -> (w1230:string)
                        n455 = local read "LAPD-Daten speichern"() -> (w1221:bool)
                        n456 = local read "Einzelbilder speichern"() -> (w1219:bool)
                        n457 = call "create_save_folder.vi"("Day folder"=w1230, "Measuring number"=w1223, "Measuring folder"=w1222, "error in"=w1225) -> ("Save Folder"=w1229:string, "Error Out"=w1228:errorcluster)  [unwired: 5 in]
                        n458 = local write "Save folder"(w1229) -> ()
                        n459 = case shown="True" w1231 {
                          tunnel: w1228 -> [w1234 w1236]
                          tunnel: [w1234 w1235] -> w1227
                          frame #0 {
                          }
                          frame #1 {
                            n460 = local read "Save folder"() -> (w1239:string)
                            n461 = Concatenate Strings(w1239, "\\Einzelbilder" ("Subfolder")) -> (w1237:string)
                            n462 = String To Path(string=w1237) -> (path=w1240:path)
                            n463 = call <vilib>:"Check if File or Folder Exists.vi"("error in (no error)"=w1236, "path"=w1240) -> ("error out"=w1235:errorcluster, "file or folder exists?"=w1241:bool, "dup path"=w1242:path)  [unwired: 7 in]
                            n464 = case shown="False" w1241 {
                              tunnel: w1242 -> [w1243 _]
                              frame #0 {
                                n465 = Create Folder(path (use dialog)=w1243) -> ()  [unwired: 2 in, 3 out]
                              }
                              frame #1 {
                              }
                            }
                          }
                        }
                        n466 = Compound Arithmetic op=OR(w1220, w1219, w1218, w1221) -> (w1217:bool)
                        n467 = local write "Daten speichern"(w1217) -> ()
                        n468 = local read "Gemittelte Bilder speichern"() -> (w1232:bool)
                        n469 = case shown="True" w1232 {
                          tunnel: w1227 -> [w1244 w1246]
                          tunnel: [w1244 w1245] -> w1226
                          frame #0 {
                          }
                          frame #1 {
                            n470 = local read "Save folder"() -> (w1250:string)
                            n471 = Concatenate Strings(w1250, "\\Gemittelte Bilder" ("Subfolder")) -> (w1252:string)
                            n472 = String To Path(string=w1252) -> (path=w1249:path)
                            n473 = call <vilib>:"Check if File or Folder Exists.vi"("error in (no error)"=w1246, "path"=w1249) -> ("error out"=w1245:errorcluster, "file or folder exists?"=w1248:bool, "dup path"=w1247:path)  [unwired: 7 in]
                            n474 = case shown="False" w1248 {
                              tunnel: w1247 -> [w1253 _]
                              frame #0 {
                                n475 = Create Folder(path (use dialog)=w1253) -> ()  [unwired: 2 in, 3 out]
                              }
                              frame #1 {
                              }
                            }
                          }
                        }
                        n476 = local read "Kamera"() -> (w1233:bool)
                        n477 = case shown="True" w1233 {
                          tunnel: [w1254 w1256] -> w1224
                          tunnel: w1226 -> [w1254 w1255]
                          frame #0 {
                          }
                          frame #1 {
                            n478 = local read "Ereignis: FrameDone?"() -> (w1257:refnum<event-registration>)
                            n479 = local read "Detektionskamera"() -> (w1258:T5)
                            n480 = call "camera_release_configuration.vi"("error in"=w1255, "Session In"=w1258, "Ereignisregistrierung (Referenz) 2"=w1257) -> ("error out"=w1256:errorcluster)  [unwired: 1 out]
                          }
                        }
                        n481 = local write "Fehler (Ausgang)"(w1224) -> ()
                      }
                    }
                  }
                  frame #1 {
                    n482 = flat-sequence {
                      frame #0 {
                        n483 = local read "Wellenplatte [°]"() -> (w1269:refnum<k7>)
                        n484 = local read "L/2-Start [°]"() -> (w1263:dbl)
                        n485 = invoke class="MG17Motor" method="SetAbsMovePos"(reference=w1269, "lChanID"=0, "fAbsPos"=w1263) -> (reference out=w1267:refnum<k7>, error out=w1264:errorcluster, "lChanID"=w1265:i32)  [unwired: 2 in, 2 out]
                        n486 = local read "Aktuelle L/2-Position [°]"() -> (w1261:dbl)
                        n487 = invoke class="MG17Motor" method="MoveAbsolute"(reference=w1267, error in=w1264, "lChanID"=w1265, "bWait"=TRUE) -> (reference out=w1260:refnum<k7>, "lChanID"=w1259:i32)  [unwired: 1 in, 3 out]
                        n488 = invoke class="MG17Motor" method="GetPosition"(reference=w1260, "lChanID"=w1259, "pfPosition"=w1261) -> ("pfPosition"=w1262:sgl)  [unwired: 2 in, 4 out]
                        n489 = local write "Aktuelle L/2-Position [°]"(w1262) -> ()
                      }
                      frame #1 {
                        n490 = local write "Leistungs-/Polarisationscan läuft"(TRUE ("Messung läuft")) -> ()
                      }
                    }
                  }
                }
              }
            }
          }
          event #5 {
            n491 = event-data() -> ("NewVal"=w1273:bool)  [unwired: 1 in]
            n492 = local read "HV-Steuerung"() -> (w1271:bool)
            n493 = local read "Kamera"() -> (w1274:bool)
            n494 = Compound Arithmetic op=AND(w1274, w1273, w1271) -> (w1272:bool)
            n495 = case shown="True" w1272 {
              frame #0 {
                n496 = local write "Spannungsscan läuft"(FALSE ("Messung läuft")) -> ()
              }
              frame #1 {
                n497 = stacked-sequence {
                  frame #0 {
                    n498 = flat-sequence {
                      tunnel: [w1289] -> w1276
                      tunnel: w1276 -> [w1310]
                      frame #0 {
                        n499 = Get Date/Time In Seconds() -> (seconds since 1Jan1904=w1277:timestamp)
                        n500 = local write "Aktueller Messschritt"(0 ("Aktueller Messschritt")) -> ()
                        n501 = local write "Start time [ms]"(w1277) -> ()
                        n502 = local read "# Spannungsschritte"() -> (w1298:i32[])
                        n503 = local read "Spannungsweite [V]"() -> (w1297:dbl[])
                        n504 = control-ref of="Shutter time (ms)"() -> (w1302:refnum<vi>)
                        n505 = property class="Ring (strikt)"(reference=w1302) -> ("RingText.Text"=w1301:string)  [unwired: 1 in, 2 out]
                        n506 = local read "Suppressor-Spannung [V]"() -> (w1279:dbl)
                        n507 = local read "# Bilder/Messschritt"() -> (w1295:i32)
                        n508 = local read "Spannungsstart [V]"() -> (w1283:dbl[])
                        n509 = local read "Tip-Spannung [V]"() -> (w1280:dbl)
                        n510 = Divide(x=w1297, y=w1298) -> (x/y=w1299:dbl[])
                        n511 = Decimal String To Number(string=w1301) -> (number=w1284:i32)  [unwired: 2 in, 1 out]
                        n512 = local read "P-Schirm-Spannung [V]"() -> (w1287:dbl)
                        n513 = local read "MCP-Spannung [V]"() -> (w1286:dbl)
                        n514 = local read "Leistung (iK) [mW]"() -> (w1285:dbl)
                        n515 = local read "Polarisation [°]"() -> (w1292:dbl)
                        n516 = local read "Messlogbuch"() -> (w1294:path)
                        n517 = local read "Proben-ID"() -> (w1293:string)
                        n518 = local write "Spannungsschritt [V]"(w1299) -> ()
                        n519 = Multiply(x=w1295, y=w1284) -> (x*y=w1296:i32)
                        n520 = Replace Array Subset(array=w1283, new element #1=w1280, index #1=0 ("Index"), new element #2=w1279, index #2=1 ("Index")) -> (w1278:dbl[])
                        n521 = local read "ROI"() -> (w1290:i32[])
                        n522 = local write "Aktuelle Spannung [V]"(w1278) -> ()
                        n523 = local write "Spannungsstart [V]"(w1278) -> ()
                        n524 = call "stage_get_current_xyz.vi"() -> ("Aktuelle xyz-Position OUT [mm]"=w1288:dbl[])  [unwired: 3 in, 1 out]
                        n525 = call "create_measure_log_entry.vi"("Messlogbuch-Pfad"=w1294, "Probe"=w1293, "Polarisation [°]"=w1292, "Messart"="Spannungsscan", "ROI"=w1290, "Messungen/Messschritt"=w1295, "Maximalleistung (iK) [mW]"=w1285, "Tip-Spannung [V]"=w1280, "Suppressor-Spannung [V]"=w1279, "Zeit/Messschritt [ms]"=w1284, "MCP-Spannung [V]"=w1286, "Zeit/Messung [ms]"=w1296, "Phosphorschirm-Spannung [V]"=w1287, "xyz [mm]"=w1288) -> ("Messung Nr."=w1289:i32)  [unwired: 4 in, 1 out]
                      }
                      frame #1 {
                        n526 = local read "Fehler (Ausgang)"() -> (w1311:errorcluster)
                        n527 = local read "Day folder"() -> (w1316:string)
                        n528 = local read "Einzelbilder speichern"() -> (w1318:bool)
                        n529 = local read "# Spannungsschritte"() -> (w1325:i32[])
                        n530 = local read "Summierte Helligkeit speichern"() -> (w1306:bool)
                        n531 = local read "Gemittelte Bilder speichern"() -> (w1304:bool)
                        n532 = call "create_save_folder.vi"("Day folder"=w1316, "Measuring number"=w1310, "Measuring folder"="Spannungsscan" ("Subfolder"), "error in"=w1311) -> ("Save Folder"=w1315:string, "Error Out"=w1314:errorcluster)  [unwired: 5 in]
                        n533 = local read "LAPD-Daten speichern"() -> (w1303:bool)
                        n534 = local read "Einzelbilder speichern"() -> (w1305:bool)
                        n535 = local write "Save folder"(w1315) -> ()
                        n536 = case shown="True" w1318 {
                          tunnel: w1314 -> [w1326 w1328]
                          tunnel: [w1326 w1327] -> w1313
                          frame #0 {
                          }
                          frame #1 {
                            n537 = local read "Save folder"() -> (w1331:string)
                            n538 = Concatenate Strings(w1331, "\\Einzelbilder" ("Subfolder")) -> (w1329:string)
                            n539 = String To Path(string=w1329) -> (path=w1332:path)
                            n540 = call <vilib>:"Check if File or Folder Exists.vi"("error in (no error)"=w1328, "path"=w1332) -> ("error out"=w1327:errorcluster, "file or folder exists?"=w1333:bool, "dup path"=w1334:path)  [unwired: 7 in]
                            n541 = case shown="False" w1333 {
                              tunnel: w1334 -> [w1335 _]
                              frame #0 {
                                n542 = Create Folder(path (use dialog)=w1335) -> ()  [unwired: 2 in, 3 out]
                              }
                              frame #1 {
                              }
                            }
                          }
                        }
                        n543 = Index Array(array=w1325, index #1=0 ("Index"), index #2=1 ("Index")) -> (element #1=w1322:i32, element #2=w1321:i32)
                        n544 = Multiply(x=w1322, y=w1321) -> (x*y=w1308:i32)
                        n545 = Compound Arithmetic op=OR(w1304, w1305, w1306, w1303) -> (w1307:bool)
                        n546 = local write "Daten speichern"(w1307) -> ()
                        n547 = local write "# Messschritte"(w1308) -> ()
                        n548 = local read "Gemittelte Bilder speichern"() -> (w1319:bool)
                        n549 = case shown="True" w1319 {
                          tunnel: w1313 -> [w1336 w1338]
                          tunnel: [w1336 w1337] -> w1312
                          frame #0 {
                          }
                          frame #1 {
                            n550 = local read "Save folder"() -> (w1342:string)
                            n551 = Concatenate Strings(w1342, "\\Gemittelte Bilder" ("Subfolder")) -> (w1344:string)
                            n552 = String To Path(string=w1344) -> (path=w1341:path)
                            n553 = call <vilib>:"Check if File or Folder Exists.vi"("error in (no error)"=w1338, "path"=w1341) -> ("error out"=w1337:errorcluster, "file or folder exists?"=w1340:bool, "dup path"=w1339:path)  [unwired: 7 in]
                            n554 = case shown="False" w1340 {
                              tunnel: w1339 -> [w1345 _]
                              frame #0 {
                                n555 = Create Folder(path (use dialog)=w1345) -> ()  [unwired: 2 in, 3 out]
                              }
                              frame #1 {
                              }
                            }
                          }
                        }
                        n556 = local read "Kamera"() -> (w1320:bool)
                        n557 = case shown="True" w1320 {
                          tunnel: [w1346 w1348] -> w1309
                          tunnel: w1312 -> [w1346 w1347]
                          frame #0 {
                          }
                          frame #1 {
                            n558 = local read "Ereignis: FrameDone?"() -> (w1349:refnum<event-registration>)
                            n559 = local read "Detektionskamera"() -> (w1350:T5)
                            n560 = call "camera_release_configuration.vi"("error in"=w1347, "Session In"=w1350, "Ereignisregistrierung (Referenz) 2"=w1349) -> ("error out"=w1348:errorcluster)  [unwired: 1 out]
                          }
                        }
                        n561 = local write "Fehler (Ausgang)"(w1309) -> ()
                      }
                    }
                  }
                  frame #1 {
                    n562 = flat-sequence {
                      frame #0 {
                        w1356 = 1 ("Index")
                        w1357 = 0 ("Index")
                        n563 = local read "# Spannungsschritte"() -> (w1367:i32[])
                        n564 = local read "Spannungsstart [V]"() -> (w1352:dbl[])
                        n565 = local read "Spannungsschritt [V]"() -> (w1355:dbl[])
                        n566 = Index Array(array=w1367, index #1=w1357, index #2=w1356) -> (element #1=w1365:i32, element #2=w1366:i32)
                        n567 = Index Array(array=w1352, index #1=w1357, index #2=w1356) -> (element #1=w1354:dbl, element #2=w1353:dbl)
                        n568 = control-ref of="2D-Intensitätsverteilung (MCP)"() -> (w1351:refnum<vi>)
                        n569 = Index Array(array=w1355, index #1=w1357, index #2=w1356) -> (element #1=w1359:dbl, element #2=w1358:dbl)
                        n570 = Initialize Array(0.0 ("y"), w1365, w1366) -> (w1363:dbl[][])
                        n571 = local write "2D-Intensitätsverteilung (MCP)"(w1363) -> ()
                        n572 = property class="IntGraph (strikt)"(reference=w1351, "XScale.Offset"=w1354, "XScale.Multiplier"=w1359, "YScale.Offset"=w1353, "YScale.Multiplier"=w1358, "XScale.MinorInc"=w1359, "YScale.MinorInc"=w1358, "XScale.NameLbl.Text"="Tip-Spannung [V]" ("Y-Achse.Namensbeschriftung.Text"), "YScale.NameLbl.Text"="Suppressor-Spannung [V]" ("X-Achse.Namensbeschriftung.Text")) -> (error out=w1362:errorcluster)  [unwired: 1 in, 1 out]
                        n573 = local write "Fehler (Ausgang)"(w1362) -> ()
                      }
                      frame #1 {
                        n574 = local write "Spannungsscan läuft"(TRUE ("Messung läuft")) -> ()
                      }
                    }
                  }
                }
              }
            }
          }
          event #6 {
            n575 = event-data() -> ("NewVal"=w1371:bool)  [unwired: 1 in]
            n576 = local read "HV-Steuerung"() -> (w1369:bool)
            n577 = local read "Kamera"() -> (w1372:bool)
            n578 = Compound Arithmetic op=AND(w1372, w1371, w1369) -> (w1370:bool)
            n579 = case shown="True" w1370 {
              frame #0 {
                n580 = local write "x-U-Scan läuft"(FALSE ("Messung läuft")) -> ()
              }
              frame #1 {
                n581 = stacked-sequence {
                  frame #0 {
                    # "Falls der gewählte Startwert für den Scan und der Startwert zur Berechnung der Ausgleichslage nicht identisch sind muss ein korrigierter Wert für die Raum-Koordinate 2 angefahren werden"
                    n582 = local read "x-U-Scan (Ausgleichslage) Steigung"() -> (w1375:dbl)
                    n583 = Not Equal?(x=w1375, y=0.0) -> (x != y?=w1376:bool)
                    n584 = case shown="True" w1376 {
                      frame #0 {
                      }
                      frame #1 {
                        n585 = flat-sequence {
                          tunnel: [w1379] -> w1377
                          tunnel: w1377 -> [w1392]
                          frame #0 {
                            n586 = local read "x-U-Scan (Ausgleichslage) xy-Start [mm]"() -> (w1390:dbl[])
                            n587 = local read "Raum-Koordinate 2 (Lagenausgleich)"() -> (w1379:enum16{"x-Achse", "y-Achse", "z-Achse"})
                            n588 = local read "Raum-Koordinate 1"() -> (w1388:enum16{"x-Achse", "y-Achse", "z-Achse"})
                            n589 = call "stage_get_current_xyz.vi"() -> ("Aktuelle xyz-Position OUT [mm]"=w1381:dbl[])  [unwired: 3 in, 1 out]
                            n590 = local read "x-U-Scan (Ausgleichslage) Steigung"() -> (w1385:dbl)
                            n591 = Index Array(array=w1381, index=w1388) -> (element=w1387:dbl)
                            n592 = Index Array(array=w1390, index #1=w1388, index #2=w1379) -> (element #1=w1389:dbl, element #2=w1382:dbl)
                            n593 = local write "x-U-Scan x-Startposition [mm]"(w1387) -> ()
                            n594 = Subtract(x=w1387, y=w1389) -> (x-y=w1386:dbl)
                            n595 = Multiply(x=w1386, y=w1385) -> (x*y=w1383:dbl)
                            n596 = Increment(x=w1379) -> (x+1=w1384:enum16{"x-Achse", "y-Achse", "z-Achse"})
                            n597 = Add(x=w1383, y=w1382) -> (x+y=w1378:dbl)
                            n598 = Replace Array Subset(array=w1381, new element=w1378, index=w1379) -> (w1380:dbl[])
                            n599 = call "stage_move_axis_absolute.vi"("Ziel xyz IN [mm]"=w1380, "Achse"=w1384) -> ()  [unwired: 1 in, 3 out]
                          }
                          frame #1 {
                            n600 = call "stage_get_current_xyz.vi"() -> ("Aktuelle xyz-Position OUT [mm]"=w1393:dbl[])  [unwired: 3 in, 1 out]
                            n601 = local write "Start xyz-Position [mm]"(w1393) -> ()
                            n602 = Index Array(array=w1393, index=w1392) -> (element=w1391:dbl)
                            n603 = local write "x-U-Scan y-Startposition [mm]"(w1391) -> ()
                          }
                        }
                      }
                    }
                  }
                  frame #1 {
                    n604 = flat-sequence {
                      tunnel: [w1409] -> w1394
                      tunnel: w1394 -> [w1440]
                      frame #0 {
                        n605 = Get Date/Time In Seconds() -> (seconds since 1Jan1904=w1400:timestamp)
                        n606 = local write "Aktueller Messschritt"(0 ("Aktueller Messschritt")) -> ()
                        n607 = local write "Start time [ms]"(w1400) -> ()
                        n608 = local read "Spannungs-Koordinate"() -> (w1419:enum16{"Tip-Spannung", "Suppressor-Spannung"})
                        n609 = local read "# x-U-Scan Spannungsschritte"() -> (w1424:i32)
                        n610 = local read "x-U-Scan x-Rasterweite [µm]"() -> (w1422:dbl)
                        n611 = local read "x-U-Scan Spannungsweite [V]"() -> (w1423:dbl)
                        n612 = local read "# x-U-Scan x-Rasterschritte"() -> (w1421:i32)
                        n613 = control-ref of="Shutter time (ms)"() -> (w1428:refnum<vi>)
                        n614 = case shown="\"Suppressor-Spannung\", Voreinstellung" w1419 {
                          tunnel: [refnum<k21> "Dev0/Ao1" ("Spannungskanal") refnum<k21> "Dev0/Ao0" ("Spannungskanal")] -> w1418
                          tunnel: [w1429 w1431] -> w1401
                          frame #0 {
                            n615 = local read "Tip-Spannung [V]"() -> (w1429:dbl)
                          }
                          frame #1 {
                            n616 = local read "Suppressor-Spannung [V]"() -> (w1431:dbl)
                          }
                        }
                        n617 = property class="Ring (strikt)"(reference=w1428) -> ("RingText.Text"=w1427:string)  [unwired: 1 in, 2 out]
                        n618 = Divide(x=w1423, y=w1424) -> (x/y=w1425:dbl)
                        n619 = Divide(x=w1422, y=w1421) -> (x/y=w1420:dbl)
                        n620 = local read "# Bilder/Messschritt"() -> (w1410:i32)
                        n621 = local write "x-U-Scan Spannungsschritt [V]"(w1425) -> ()
                        n622 = local write "x-U-Scan x-Rasterschritt [µm]"(w1420) -> ()
                        n623 = Decimal String To Number(string=w1427) -> (number=w1411:i32)  [unwired: 2 in, 1 out]
                        n624 = local read "Suppressor-Spannung [V]"() -> (w1405:dbl)
                        n625 = local read "P-Schirm-Spannung [V]"() -> (w1408:dbl)
                        n626 = local read "MCP-Spannung [V]"() -> (w1407:dbl)
                        n627 = local read "Leistung (iK) [mW]"() -> (w1406:dbl)
                        n628 = local read "Tip-Spannung [V]"() -> (w1404:dbl)
                        n629 = local read "Polarisation [°]"() -> (w1415:dbl)
                        n630 = local read "Messlogbuch"() -> (w1417:path)
                        n631 = local read "Proben-ID"() -> (w1416:string)
                        n632 = Multiply(x=w1410, y=w1411) -> (x*y=w1412:i32)
                        n633 = local read "Raum-Koordinate 2 (Lagenausgleich)"() -> (w1397:enum16{"x-Achse", "y-Achse", "z-Achse"})
                        n634 = local read "ROI"() -> (w1413:i32[])
                        n635 = local read "Raum-Koordinate 1"() -> (w1398:enum16{"x-Achse", "y-Achse", "z-Achse"})
                        n636 = call "stage_get_current_xyz.vi"() -> ("Aktuelle xyz-Position OUT [mm]"=w1399:dbl[])  [unwired: 3 in, 1 out]
                        n637 = call "create_measure_log_entry.vi"("Messlogbuch-Pfad"=w1417, "Probe"=w1416, "Polarisation [°]"=w1415, "Messart"="x-U-Scan", "ROI"=w1413, "Messungen/Messschritt"=w1410, "Maximalleistung (iK) [mW]"=w1406, "Tip-Spannung [V]"=w1404, "Suppressor-Spannung [V]"=w1405, "Zeit/Messschritt [ms]"=w1411, "MCP-Spannung [V]"=w1407, "Zeit/Messung [ms]"=w1412, "Phosphorschirm-Spannung [V]"=w1408, "xyz [mm]"=w1399) -> ("Messung Nr."=w1409:i32)  [unwired: 4 in, 1 out]
                        n638 = local write "Start xyz-Position [mm]"(w1399) -> ()
                        n639 = Index Array(array=w1399, index #1=w1398, index #2=w1397) -> (element #1=w1395:dbl, element #2=w1396:dbl)
                        n640 = Add(x=w1398, y=1) -> (x+y=w1402:i32)
                        n641 = local write "x-U-Scan aktuelle y-Position [mm]"(w1396) -> ()
                        n642 = local write "x-U-Scan aktuelle x-Position [mm]"(w1395) -> ()
                        n643 = local write "x-U-Scan y-Startposition [mm]"(w1396) -> ()
                        n644 = local write "x-U-Scan x-Startposition [mm]"(w1395) -> ()
                        n645 = local write "x-U-Scan aktuelle Spannung [V]"(w1401) -> ()
                        n646 = local write "x-U-Scan Spannungsstart [V]"(w1401) -> ()
                        n647 = local write "Spannungskanal"(w1418) -> ()
                        n648 = local write "Achs-ID"(w1402) -> ()
                      }
                      frame #1 {
                        n649 = local read "Fehler (Ausgang)"() -> (w1443:errorcluster)
                        n650 = local read "Day folder"() -> (w1448:string)
                        n651 = local read "Summierte Helligkeit speichern"() -> (w1436:bool)
                        n652 = local read "# x-U-Scan Spannungsschritte"() -> (w1439:i32)
                        n653 = local read "# x-U-Scan x-Rasterschritte"() -> (w1438:i32)
                        n654 = local read "Gemittelte Bilder speichern"() -> (w1434:bool)
                        n655 = local read "LAPD-Daten speichern"() -> (w1433:bool)
                        n656 = local read "Einzelbilder speichern"() -> (w1435:bool)
                        n657 = local read "Einzelbilder speichern"() -> (w1450:bool)
                        n658 = call "create_save_folder.vi"("Day folder"=w1448, "Measuring number"=w1440, "Measuring folder"="x-U-Scan" ("Subfolder"), "error in"=w1443) -> ("Save Folder"=w1447:string, "Error Out"=w1446:errorcluster)  [unwired: 5 in]
                        n659 = Multiply(x=w1439, y=w1438) -> (x*y=w1441:i32)
                        n660 = local write "Save folder"(w1447) -> ()
                        n661 = case shown="True" w1450 {
                          tunnel: w1446 -> [w1453 w1455]
                          tunnel: [w1453 w1454] -> w1445
                          frame #0 {
                          }
                          frame #1 {
                            n662 = local read "Save folder"() -> (w1458:string)
                            n663 = Concatenate Strings(w1458, "\\Einzelbilder" ("Subfolder")) -> (w1456:string)
                            n664 = String To Path(string=w1456) -> (path=w1459:path)
                            n665 = call <vilib>:"Check if File or Folder Exists.vi"("error in (no error)"=w1455, "path"=w1459) -> ("error out"=w1454:errorcluster, "file or folder exists?"=w1460:bool, "dup path"=w1461:path)  [unwired: 7 in]
                            n666 = case shown="False" w1460 {
                              tunnel: w1461 -> [w1462 _]
                              frame #0 {
                                n667 = Create Folder(path (use dialog)=w1462) -> ()  [unwired: 2 in, 3 out]
                              }
                              frame #1 {
                              }
                            }
                          }
                        }
                        n668 = Compound Arithmetic op=OR(w1434, w1435, w1436, w1433) -> (w1437:bool)
                        n669 = local write "Daten speichern"(w1437) -> ()
                        n670 = local write "# Messschritte"(w1441) -> ()
                        n671 = local read "Gemittelte Bilder speichern"() -> (w1451:bool)
                        n672 = case shown="True" w1451 {
                          tunnel: w1445 -> [w1463 w1465]
                          tunnel: [w1463 w1464] -> w1444
                          frame #0 {
                          }
                          frame #1 {
                            n673 = local read "Save folder"() -> (w1469:string)
                            n674 = Concatenate Strings(w1469, "\\Gemittelte Bilder" ("Subfolder")) -> (w1471:string)
                            n675 = String To Path(string=w1471) -> (path=w1468:path)
                            n676 = call <vilib>:"Check if File or Folder Exists.vi"("error in (no error)"=w1465, "path"=w1468) -> ("error out"=w1464:errorcluster, "file or folder exists?"=w1467:bool, "dup path"=w1466:path)  [unwired: 7 in]
                            n677 = case shown="False" w1467 {
                              tunnel: w1466 -> [w1472 _]
                              frame #0 {
                                n678 = Create Folder(path (use dialog)=w1472) -> ()  [unwired: 2 in, 3 out]
                              }
                              frame #1 {
                              }
                            }
                          }
                        }
                        n679 = local read "Kamera"() -> (w1452:bool)
                        n680 = case shown="True" w1452 {
                          tunnel: [w1473 w1475] -> w1442
                          tunnel: w1444 -> [w1473 w1474]
                          frame #0 {
                          }
                          frame #1 {
                            n681 = local read "Ereignis: FrameDone?"() -> (w1476:refnum<event-registration>)
                            n682 = local read "Detektionskamera"() -> (w1477:T5)
                            n683 = call "camera_release_configuration.vi"("error in"=w1474, "Session In"=w1477, "Ereignisregistrierung (Referenz) 2"=w1476) -> ("error out"=w1475:errorcluster)  [unwired: 1 out]
                          }
                        }
                        n684 = local write "Fehler (Ausgang)"(w1442) -> ()
                      }
                    }
                  }
                  frame #2 {
                    n685 = flat-sequence {
                      frame #0 {
                        n686 = local read "# x-U-Scan Spannungsschritte"() -> (w1486:i32)
                        n687 = local read "x-U-Scan x-Rasterschritt [µm]"() -> (w1479:dbl)
                        n688 = local read "# x-U-Scan x-Rasterschritte"() -> (w1485:i32)
                        n689 = Initialize Array(0.0 ("y"), w1485, w1486) -> (w1490:dbl[][])
                        n690 = Divide(x=w1479, y=1000.0) -> (x/y=w1480:dbl)
                        n691 = local write "2D-Intensitätsverteilung (MCP)"(w1490) -> ()
                        n692 = local read "x-U-Scan Spannungsschritt [V]"() -> (w1482:dbl)
                        n693 = local read "x-U-Scan x-Startposition [mm]"() -> (w1483:dbl)
                        n694 = local read "x-U-Scan Spannungsstart [V]"() -> (w1484:dbl)
                        n695 = control-ref of="2D-Intensitätsverteilung (MCP)"() -> (w1481:refnum<vi>)
                        n696 = property class="IntGraph (strikt)"(reference=w1481, "XScale.Offset"=w1483, "XScale.Multiplier"=w1480, "YScale.Offset"=w1484, "YScale.Multiplier"=w1482, "XScale.MinorInc"=w1480, "YScale.MinorInc"=w1482, "XScale.NameLbl.Text"="Position [mm]" ("Y-Achse.Namensbeschriftung.Text"), "YScale.NameLbl.Text"="Spannung [V]" ("X-Achse.Namensbeschriftung.Text")) -> (error out=w1489:errorcluster)  [unwired: 1 in, 1 out]
                        n697 = local write "Fehler (Ausgang)"(w1489) -> ()
                      }
                      frame #1 {
                        n698 = local write "x-U-Scan läuft"(TRUE ("Messung läuft")) -> ()
                      }
                    }
                  }
                }
              }
            }
          }
          event #7 {
            n699 = event-data() -> ("NewVal"=w1493:bool)  [unwired: 1 in]
            n700 = case shown="True" w1493 {
              frame #0 {
              }
              frame #1 {
                n701 = flat-sequence {
                  tunnel: [w1498] -> w1494
                  tunnel: w1494 -> [w1515]
                  frame #0 {
                    n702 = local write "Ausgleichslage Start festlegen"(FALSE ("Ausgleichslage Ende festlegen")) -> ()
                    n703 = local read "Raum-Koordinate 2 (Lagenausgleich)"() -> (w1496:enum16{"x-Achse", "y-Achse", "z-Achse"})
                    n704 = local read "Raum-Koordinate 1"() -> (w1497:enum16{"x-Achse", "y-Achse", "z-Achse"})
                    n705 = local read "x-U-Scan (Ausgleichslage) xy-Start [mm]"() -> (w1499:dbl[])
                    n706 = call "stage_get_current_xyz.vi"() -> ("Aktuelle xyz-Position OUT [mm]"=w1504:dbl[])  [unwired: 3 in, 1 out]
                    n707 = Index Array(array=w1504, index #1=w1497, index #2=w1496) -> (element #1=w1501:dbl, element #2=w1500:dbl)
                    n708 = Replace Array Subset(array=w1499, new element #1=w1501, index #1=0 ("Index"), new element #2=w1500, index #2=1 ("Index")) -> (w1498:dbl[])
                    n709 = local write "x-U-Scan (Ausgleichslage) xy-Start [mm]"(w1498) -> ()
                  }
                  frame #1 {
                    n710 = local read "x-U-Scan (Ausgleichslage) xy-End [mm]"() -> (w1516:dbl[])
                    n711 = Index Array(array=w1515, index #1=0 ("Index"), index #2=1 ("Index")) -> (element #1=w1507:dbl, element #2=w1510:dbl)
                    n712 = Index Array(array=w1516, index #1=0 ("Index"), index #2=1 ("Index")) -> (element #1=w1506:dbl, element #2=w1509:dbl)
                    n713 = Not Equal?(x=w1507, y=w1506) -> (x != y?=w1505:bool)
                    n714 = case shown="True" w1505 {
                      tunnel: w1510 -> [_ w1522]
                      tunnel: w1509 -> [_ w1521]
                      tunnel: w1506 -> [_ w1520]
                      tunnel: w1507 -> [_ w1519]
                      tunnel: [0.0 w1518] -> w1508
                      frame #0 {
                      }
                      frame #1 {
                        n715 = Subtract(x=w1522, y=w1521) -> (x-y=w1524:dbl)
                        n716 = Subtract(x=w1519, y=w1520) -> (x-y=w1523:dbl)
                        n717 = Divide(x=w1524, y=w1523) -> (x/y=w1518:dbl)
                      }
                    }
                    n718 = local write "x-U-Scan (Ausgleichslage) Steigung"(w1508) -> ()
                  }
                }
              }
            }
          }
          event #8 {
            n719 = event-data() -> ("NewVal"=w1525:bool)  [unwired: 1 in]
            n720 = case shown="True" w1525 {
              frame #0 {
              }
              frame #1 {
                n721 = flat-sequence {
                  tunnel: [w1530] -> w1526
                  tunnel: w1526 -> [w1547]
                  frame #0 {
                    n722 = local write "Ausgleichslage Ende festlegen"(FALSE ("Ausgleichslage Ende festlegen")) -> ()
                    n723 = local read "Raum-Koordinate 2 (Lagenausgleich)"() -> (w1528:enum16{"x-Achse", "y-Achse", "z-Achse"})
                    n724 = local read "Raum-Koordinate 1"() -> (w1529:enum16{"x-Achse", "y-Achse", "z-Achse"})
                    n725 = local read "x-U-Scan (Ausgleichslage) xy-End [mm]"() -> (w1531:dbl[])
                    n726 = call "stage_get_current_xyz.vi"() -> ("Aktuelle xyz-Position OUT [mm]"=w1536:dbl[])  [unwired: 3 in, 1 out]
                    n727 = Index Array(array=w1536, index #1=w1529, index #2=w1528) -> (element #1=w1533:dbl, element #2=w1532:dbl)
                    n728 = Replace Array Subset(array=w1531, new element #1=w1533, index #1=0 ("Index"), new element #2=w1532, index #2=1 ("Index")) -> (w1530:dbl[])
                    n729 = local write "x-U-Scan (Ausgleichslage) xy-End [mm]"(w1530) -> ()
                  }
                  frame #1 {
                    n730 = local read "x-U-Scan (Ausgleichslage) xy-Start [mm]"() -> (w1548:dbl[])
                    n731 = Index Array(array=w1547, index #1=0 ("Index"), index #2=1 ("Index")) -> (element #1=w1539:dbl, element #2=w1542:dbl)
                    n732 = Index Array(array=w1548, index #1=0 ("Index"), index #2=1 ("Index")) -> (element #1=w1538:dbl, element #2=w1541:dbl)
                    n733 = Not Equal?(x=w1539, y=w1538) -> (x != y?=w1537:bool)
                    n734 = case shown="True" w1537 {
                      tunnel: w1542 -> [_ w1554]
                      tunnel: w1541 -> [_ w1553]
                      tunnel: w1538 -> [_ w1552]
                      tunnel: w1539 -> [_ w1551]
                      tunnel: [0.0 w1550] -> w1540
                      frame #0 {
                      }
                      frame #1 {
                        n735 = Subtract(x=w1554, y=w1553) -> (x-y=w1556:dbl)
                        n736 = Subtract(x=w1551, y=w1552) -> (x-y=w1555:dbl)
                        n737 = Divide(x=w1556, y=w1555) -> (x/y=w1550:dbl)
                      }
                    }
                    n738 = local write "x-U-Scan (Ausgleichslage) Steigung"(w1540) -> ()
                  }
                }
              }
            }
          }
          event #9 {
            n739 = event-data() -> ("NewVal"=w1557:bool)  [unwired: 1 in]
            n740 = case shown="True" w1557 {
              frame #0 {
              }
              frame #1 {
                n741 = stacked-sequence {
                  seq-local: [w1578 _ _ _] -> [_ w1584 _ _]
                  seq-local: [w1577 _ _ _] -> [_ w1587 _ _]
                  seq-local: [w1559 _ _ _] -> [_ w1586 _ _]
                  seq-local: [_ w1587 _ _] -> [_ _ w1598 _]
                  seq-local: [_ w1586 _ _] -> [_ _ w1597 _]
                  seq-local: [_ w1583 _ _] -> [_ _ w1600 _]
                  seq-local: [_ w1582 _ _] -> [_ _ w1599 _]
                  seq-local: [_ _ w1596 _] -> [_ _ _ w1626]
                  seq-local: [_ _ w1595 _] -> [_ _ _ w1625]
                  frame #0 {
                    n742 = local read "# Messpunkte"() -> (w1558:i32)
                    n743 = control-ref of="Shutter time (ms)"() -> (w1581:refnum<vi>)
                    n744 = property class="Ring (strikt)"(reference=w1581) -> ("RingText.Text"=w1561:string)  [unwired: 1 in, 2 out]
                    n745 = local write "# Messschritte"(w1558) -> ()
                    n746 = local read "# Bilder/Messschritt"() -> (w1575:i32)
                    n747 = local read "Suppressor-Spannung [V]"() -> (w1562:dbl)
                    n748 = local read "P-Schirm-Spannung [V]"() -> (w1567:dbl)
                    n749 = Decimal String To Number(string=w1561) -> (number=w1574:i32)  [unwired: 2 in, 1 out]
                    n750 = local read "MCP-Spannung [V]"() -> (w1566:dbl)
                    n751 = Concatenate Strings(w1561, "ms_" ("String")) -> (w1559:string)
                    n752 = local read "Leistung (iK) [mW]"() -> (w1565:dbl)
                    n753 = local read "Tip-Spannung [V]"() -> (w1563:dbl)
                    n754 = local read "Polarisation [°]"() -> (w1570:dbl)
                    n755 = local read "Messlogbuch"() -> (w1572:path)
                    n756 = Multiply(x=w1575, y=w1574) -> (x*y=w1573:i32)
                    n757 = local read "Proben-ID"() -> (w1571:string)
                    n758 = local read "ROI"() -> (w1568:i32[])
                    n759 = local read "Sequenz Ordner"() -> (w1579:string)
                    n760 = local read "Day folder"() -> (w1580:string)
                    n761 = call "stage_get_current_xyz.vi"() -> ("Aktuelle xyz-Position OUT [mm]"=w1576:dbl[])  [unwired: 3 in, 1 out]
                    n762 = call "create_measure_log_entry.vi"("Messlogbuch-Pfad"=w1572, "Probe"=w1571, "Polarisation [°]"=w1570, "Messart"="Referenzbilder", "ROI"=w1568, "Messungen/Messschritt"=w1575, "Maximalleistung (iK) [mW]"=w1565, "Tip-Spannung [V]"=w1563, "Suppressor-Spannung [V]"=w1562, "Zeit/Messschritt [ms]"=w1574, "MCP-Spannung [V]"=w1566, "Zeit/Messung [ms]"=w1573, "Phosphorschirm-Spannung [V]"=w1567, "xyz [mm]"=w1576) -> ("Messung Nr."=w1564:i32)  [unwired: 4 in, 1 out]
                    n763 = call "create_save_folder.vi"("Day folder"=w1580, "Measuring number"=w1564, "Measuring folder"=w1579) -> ("Save Folder"=w1577:string, "Error Out"=w1578:errorcluster)  [unwired: 6 in]
                    n764 = local write "Save folder"(w1577) -> ()
                  }
                  frame #1 {
                    n765 = local read "Kamera"() -> (w1585:bool)
                    n766 = case shown="True" w1585 {
                      tunnel: [w1589 w1592] -> w1582
                      tunnel: w1584 -> [w1588 w1591]
                      tunnel: [w1588 w1590] -> w1583
                      frame #0 {
                        n767 = local read "Detektionskamera"() -> (w1589:T5)
                      }
                      frame #1 {
                        n768 = local read "Ereignis: FrameDone?"() -> (w1593:refnum<event-registration>)
                        n769 = local read "Detektionskamera"() -> (w1594:T5)
                        n770 = call "camera_release_configuration.vi"("error in"=w1591, "Session In"=w1594, "Ereignisregistrierung (Referenz) 2"=w1593) -> ("error out"=w1590:errorcluster, "Session Out"=w1592:T5)
                      }
                    }
                  }
                  frame #2 {
                    n771 = for {
                      N: "# Messpunkte" -> [_]
                      tunnel: [w1608] -> w1595
                      tunnel: [w1607] -> w1596
                      tunnel: w1598 -> [w1606]
                      tunnel: w1597 -> [w1604]
                      tunnel: w1600 -> [w1603]
                      tunnel: w1599 -> [w1602]
                      i -> [w1605]
                      n772 = stacked-sequence {
                        tunnel: [w1618 _] -> w1608
                        tunnel: [w1617 _] -> w1607
                        tunnel: w1606 -> [w1616 _]
                        tunnel: w1605 -> [w1609 _]
                        tunnel: w1604 -> [w1614 _]
                        tunnel: w1603 -> [w1612 _]
                        tunnel: w1602 -> [w1611 _]
                        frame #0 {
                          n773 = local read "# Bilder/Messschritt"() -> (w1620:i32)
                          n774 = Format Into String(format string="#%03.0f" ("Format-String"), initial string=w1614, w1609) -> (resulting string=w1613:string)  [unwired: 1 in, 1 out]
                          n775 = Increment(x=w1609) -> (x+1=w1610:i32)
                          n776 = local write "Aktueller Messschritt"(w1610) -> ()
                          n777 = call "camera_acquisition_sequence.vi"("Session In"=w1611, "Desired image number"=w1620, "error in"=w1612) -> ("Session Out"=w1617:T5, "Image Array"=w1621:T4[], "error out"=w1619:errorcluster)  [unwired: 1 in]
                          n778 = call "save images.vi"("Save Folder"=w1616, "File name prefix"=w1613, "Array"=w1621, "error out 2"=w1619, "Bilder/Messschritt"=w1620) -> ("error out"=w1618:errorcluster)
                        }
                        frame #1 {
                          n779 = Multiply(x=i64 1000, y="Verzögerung [s]") -> (x*y=w1623:i64)
                          n780 = Wait (ms)(milliseconds to wait=w1623) -> ()  [unwired: 1 out]
                        }
                      }
                    }
                  }
                  frame #3 {
                    n781 = local read "Buffer Interval"() -> (w1631:u32)
                    n782 = call "camera_create_configuration.vi"("error in"=w1625, "BufferInterval"=w1631, "Session Out 2"=w1626) -> ("Fehler (Ausgang)"=w1629:errorcluster, "Session Out"=w1628:T5, "Ereignisregistrierung (Referenz)"=w1627:refnum<event-registration>)
                    n783 = local write "Ereignis: FrameDone?"(w1627) -> ()
                    n784 = local write "Detektionskamera"(w1628) -> ()
                    n785 = local write "Fehler (Ausgang)"(w1629) -> ()
                    n786 = Unbundle By Name(w1629) -> ("status"=w1630:bool)
                    n787 = local write "Sequenzaufnahme ON"(w1630) -> ()
                  }
                }
              }
            }
          }
          event #10 {
            n788 = event-data() -> ()  [unwired: 1 in, 1 out]
            n789 = control-ref of="Shutter time (ms)"() -> (w1642:refnum<vi>)
            n790 = property class="Ring (strikt)"(reference=w1642) -> ("RingText.Text"=w1641:string)  [unwired: 1 in, 2 out]
            n791 = local read "# Bilder/Messschritt"() -> (w1639:i32)
            n792 = local read "Verzögerung [s]"() -> (w1644:i64)
            n793 = local read "# Messpunkte"() -> (w1640:i32)
            n794 = Decimal String To Number(string=w1641) -> (number=w1638:i32)  [unwired: 2 in, 1 out]
            n795 = Multiply(x=w1640, y=w1644) -> (x*y=w1643:i64)
            n796 = Compound Arithmetic op=MULTIPLY(w1640, w1639, w1638) -> (w1637:i32)
            n797 = Divide(x=w1637, y=1000) -> (x/y=w1636:dbl)
            n798 = Add(x=w1643, y=w1636) -> (x+y=w1634:dbl)
            n799 = Divide(x=w1634, y=60.0) -> (x/y=→"Gesamtzeit [min]":dbl)
          }
        }
        n800 = local read "Fehler (Ausgang)"() -> (w647:errorcluster)
        n801 = local read "Programm beenden"() -> (w645:bool)
        n802 = Unbundle By Name(w647) -> ("status"=w646:bool)
        n803 = Or(x=w646, y=w645) -> (x .or. y?=w642:bool)
        "Scanschleifenzähler" <- w643
      }
      n804 = while "Leistungs-/Polarisationsscan-Schleife" {
        stop <- w43 stop-if-true
        n805 = local read "Fehler (Ausgang)"() -> (w46:errorcluster)
        n806 = local read "Leistungs-/Polarisationscan läuft"() -> (w42:bool)
        n807 = local read "Programm beenden"() -> (w44:bool)
        n808 = Unbundle By Name(w46) -> ("status"=w45:bool)
        n809 = Or(x=w45, y=w44) -> (x .or. y?=w43:bool)
        n810 = case shown="True" w42 {
          frame #0 {
            n811 = stacked-sequence {
              frame #0 {
                n812 = local read "Leist/Pol # Schleifen"() -> (w47:i64)
                n813 = for {
                  N: w47 -> [_]
                  i -> [w48]
                  n814 = local read "# L/2-Schritte"() -> (w49:i32)
                  n815 = for "Schleife für L/2-Position" {
                    N: w49 -> [_]
                    tunnel: w48 -> [w51]
                    i -> [w50]
                    n816 = local read "Leistungs-/Polarisationscan läuft"() -> (w52:bool)
                    n817 = case shown="True" w52 {
                      tunnel: w51 -> [w54 _]
                      tunnel: w50 -> [w53 _]
                      frame #0 {
                        n818 = stacked-sequence {
                          tunnel: w54 -> [_ _ _ _ w158]
                          tunnel: w53 -> [_ _ _ _ w153]
                          frame #0 {
                            n819 = local write "Summierte Helligkeit (a.u.)"(u64 0 ("Summierte Helligkeit (a.u.)")) -> ()
                            n820 = local read "ROI"() -> (w60:i32[])
                            n821 = local read "Aktueller Messschritt"() -> (w57:i32)
                            n822 = Index Array(array=w60, index #1=0 ("Index"), index #2=1 ("Index")) -> (element #1=w64:i32, element #2=w63:i32)
                            n823 = Initialize Array(u64 0 ("Element"), w63, w64) -> (w58:u64[][])
                            n824 = local write "Gemitteltes Bild"(w58) -> ()
                            n825 = Increment(x=w57) -> (x+1=w56:i32)
                            n826 = local write "Aktueller Messschritt"(w56) -> ()
                          }
                          frame #1 {
                            n827 = local read "# Bilder/Messschritt"() -> (w68:i32)
                            n828 = local read "Detektionskamera"() -> (w71:T5)
                            n829 = local read "Einzelbilder speichern"() -> (w66:bool)
                            n830 = call "camera_acquisition_sequence.vi"("Session In"=w71, "Desired image number"=w68) -> ("Image Array"=w65:T4[], "error out"=w70:errorcluster)  [unwired: 2 in, 1 out]
                            n831 = case shown="True" w66 {
                              tunnel: w70 -> [w73 w81]
                              tunnel: [w73 w80] -> w69
                              tunnel: w68 -> [w72 w79]
                              tunnel: [w72 w79] -> w67
                              tunnel: w65 -> [_ w78]
                              frame #0 {
                              }
                              frame #1 {
                                n832 = local read "Aktueller Messschritt"() -> (w84:i32)
                                n833 = local read "Save folder"() -> (w76:string)
                                n834 = Concatenate Strings(w76, "Einzelbilder\\" ("String")) -> (w74:string)
                                n835 = Format Into String(format string="%05.0f" ("Format-String"), initial string="#" ("Eingangs-String"), w84) -> (resulting string=w77:string)  [unwired: 1 in, 1 out]
                                n836 = call "save images.vi"("Save Folder"=w74, "File name prefix"=w77, "Array"=w78, "error out 2"=w81, "Bilder/Messschritt"=w79) -> ("error out"=w80:errorcluster)
                              }
                            }
                            n837 = for {
                              N: w67 -> [_]
                              tunnel: w69 -> [w94]
                              tunnel: w65 -> [w92] mode=indexing
                              n838 = call "IMAQ ImageToArray"("error in (no error)"=w94, "Image"=w92) -> ("error out"=w93:errorcluster, "Image Pixels (U8)"=w91:u8[][])  [unwired: 2 in, 3 out]
                              n839 = local read "Gemitteltes Bild"() -> (w89:u64[][])
                              n840 = local read "Hintergrund-Helligkeit"() -> (w85:i64)
                              n841 = To Quad Integer(1:w91) -> (0:w95:i64[][])
                              n842 = local write "Fehler (Ausgang)"(w93) -> ()
                              n843 = local read "Summierte Helligkeit (a.u.)"() -> (w88:i64)
                              n844 = Add Array Elements(numeric array=w95) -> (sum=w87:i64)
                              n845 = Add(x=w89, y=w91) -> (x+y=w90:u64[][])
                              n846 = Subtract(x=w87, y=w85) -> (x-y=w86:i64)
                              n847 = local write "Gemitteltes Bild"(w90) -> ()
                              n848 = Add(x=w86, y=w88) -> (x+y=w96:i64)
                              n849 = local write "Summierte Helligkeit (a.u.)"(w96) -> ()
                            }
                          }
                          frame #2 {
                            n850 = flat-sequence {
                              frame #0 {
                                n851 = local read "# Bilder/Messschritt"() -> (w99:i32)
                                n852 = local read "Gemitteltes Bild"() -> (w97:u64[][])
                                n853 = local read "Gemittelte Bilder speichern"() -> (w103:bool)
                                n854 = local read "Image Display"() -> (w101:T4)
                                n855 = Divide(x=w97, y=w99) -> (x/y=w98:dbl[][])
                                n856 = call "IMAQ ArrayToImage"("Image Pixels (U8)"=w98, "Image"=w101) -> ("Image Out"=w100:T4)  [unwired: 8 in, 1 out]
                                n857 = case shown="True" w103 {
                                tunnel: w100 -> [w104 w115]
                                tunnel: [w104 w106] -> w102
                                frame #0 {
                                }
                                frame #1 {
                                n858 = local read "Aktueller Messschritt"() -> (w110:i32)
                                n859 = local read "Save folder"() -> (w112:string)
                                n860 = Format Into String(format string="%05.0f" ("Format-String"), initial string="#" ("Eingangs-String"), w110) -> (resulting string=w109:string)  [unwired: 1 in, 1 out]
                                n861 = Concatenate Strings(w112, "Gemittelte Bilder\\" ("String"), w109, ".png" ("String")) -> (w108:string)
                                n862 = String To Path(string=w108) -> (path=w107:path)
                                n863 = call-poly "IMAQ Write File 2"("File Path"=w107, "Image"=w115) -> ("Image Out (duplicate)"=w106:T4)  [unwired: 8 in, 1 out]
                                }
                                }
                                n864 = local write "Image Display"(w102) -> ()
                              }
                              frame #1 {
                                n865 = local read "Aktuelle L/2-Position [°]"() -> (w121:dbl)
                                n866 = local read "Summierte Helligkeit (a.u.)"() -> (w120:i64)
                                n867 = local read "Aktueller Messschritt"() -> (w119:i32)
                                n868 = local read "Vektor Summierte Helligkeit [a.u.]"() -> (w123:dbl[])
                                n869 = local read "Vektor L/2-Position [°]"() -> (w122:dbl[])
                                n870 = Decrement(x=w119) -> (x-1=w118:i32)
                                n871 = Replace Array Subset(array=w122, new element=w121, index=w118) -> (w117:dbl[])
                                n872 = Replace Array Subset(array=w123, new element=w120, index=w118) -> (w116:dbl[])
                                n873 = local write "Vektor L/2-Position [°]"(w117) -> ()
                                n874 = local write "Vektor Summierte Helligkeit [a.u.]"(w116) -> ()
                                n875 = Bundle("Vektor L/2-Position [°]"=w117, "Vektor Summierte Helligkeit [a.u.]"=w116) -> (→"1D-Intensitätsverteilung (MCP)":T3)  [unwired: 1 in]
                              }
                            }
                          }
                          frame #3 {
                            # "Anfahren der Anfangsleistung zur Signalsättigung und warten für die mit \"Sättigungszeit\" eingestellte Zeit"
                            n876 = Not Equal?(x="Sättigungszeit [s]", y=0.0) -> (x != y?=w127:bool)
                            n877 = case shown="True" w127 {
                              frame #0 {
                              }
                              frame #1 {
                                n878 = stacked-sequence {
                                seq-local: [_ w131 _ _] -> [_ _ w141 _]
                                seq-local: [_ w130 _ _] -> [_ _ w140 _]
                                seq-local: [_ w129 _ _] -> [_ _ w139 _]
                                seq-local: [_ _ w141 _] -> [_ _ _ w148]
                                seq-local: [_ _ w140 _] -> [_ _ _ w147]
                                seq-local: [_ _ w139 _] -> [_ _ _ w146]
                                frame #0 {
                                n879 = local read "Aktuelle L/2-Position [°]"() -> (→"Vorherige L/2 Position [°]":dbl)
                                }
                                frame #1 {
                                n880 = local read "Wellenplatte [°]"() -> (w132:refnum<k7>)
                                n881 = local read "L/2-Start [°]"() -> (w138:dbl)
                                n882 = invoke class="MG17Motor" method="SetAbsMovePos"(reference=w132, "lChanID"=0, "fAbsPos"=w138) -> (reference out=w134:refnum<k7>, error out=w137:errorcluster, "lChanID"=w136:i32)  [unwired: 2 in, 2 out]
                                n883 = invoke class="MG17Motor" method="MoveAbsolute"(reference=w134, error in=w137, "lChanID"=w136, "bWait"=TRUE) -> (reference out=w130:refnum<k7>, error out=w129:errorcluster, "lChanID"=w131:i32)  [unwired: 1 in, 2 out]
                                }
                                frame #2 {
                                n884 = local read "Sättigungszeit [s]"() -> (w144:dbl)
                                n885 = Multiply(x=w144, y=1000.0) -> (x*y=w142:dbl)
                                n886 = Wait (ms)(milliseconds to wait=w142) -> ()  [unwired: 1 out]
                                }
                                frame #3 {
                                n887 = local read "Vorherige L/2 Position [°]"() -> (w145:dbl)
                                n888 = invoke class="MG17Motor" method="SetAbsMovePos"(reference=w147, error in=w146, "lChanID"=w148, "fAbsPos"=w145) -> (reference out=w150:refnum<k7>, error out=w152:errorcluster, "lChanID"=w151:i32)  [unwired: 1 in, 2 out]
                                n889 = invoke class="MG17Motor" method="MoveAbsolute"(reference=w150, error in=w152, "lChanID"=w151, "bWait"=TRUE) -> ()  [unwired: 1 in, 5 out]
                                }
                                }
                              }
                            }
                          }
                          frame #4 {
                            n890 = flat-sequence {
                              tunnel: w158 -> [w165]
                              tunnel: [w164] -> w157
                              tunnel: [w163] -> w156
                              tunnel: w153 -> [w162]
                              tunnel: w157 -> [w186]
                              tunnel: w156 -> [w187]
                              tunnel: [w187] -> w155
                              tunnel: [w186] -> w154
                              tunnel: w155 -> [w191]
                              tunnel: w154 -> [w190]
                              frame #0 {
                                # "Neue Polarisatorstellung"
                                n891 = Increment(x=w162) -> (x+1=w161:i32)
                                n892 = local read "# L/2-Schritte"() -> (w160:i32)
                                n893 = Not Equal?(x=w160, y=w161) -> (x != y?=w159:bool)
                                n894 = case shown="True" w159 {
                                tunnel: w165 -> [_ w172]
                                tunnel: [0 ("lChanID") w169] -> w164
                                tunnel: [w167 w168] -> w163
                                frame #0 {
                                n895 = local read "Wellenplatte [°]"() -> (w167:refnum<k7>)
                                }
                                frame #1 {
                                n896 = Equal?(x=w172, y=0) -> (x = y?=w170:bool)
                                n897 = local read "L/2-Schritt [°]"() -> (w174:dbl)
                                n898 = local read "Wellenplatte [°]"() -> (w175:refnum<k7>)
                                n899 = case shown="False" w170 {
                                tunnel: w174 -> [w181 w182]
                                tunnel: [w180 w182] -> w173
                                frame #0 {
                                n900 = Negate(x=w181) -> (-x=w180:dbl)
                                }
                                frame #1 {
                                }
                                }
                                n901 = invoke class="MG17Motor" method="SetRelMoveDist"(reference=w175, "lChanID"=0, "fRelDist"=w173) -> (reference out=w177:refnum<k7>, "lChanID"=w178:i32)  [unwired: 2 in, 3 out]
                                n902 = invoke class="MG17Motor" method="MoveRelative"(reference=w177, "lChanID"=w178, "bWait"=TRUE) -> (reference out=w168:refnum<k7>, "lChanID"=w169:i32)  [unwired: 2 in, 3 out]
                                }
                                }
                              }
                              frame #1 {
                                # "Wartezeit für\nneue Polarisatorposition"
                                n903 = local read "Wartezeit [s]"() -> (w184:dbl)
                                n904 = Multiply(x=w184, y=1000.0) -> (x*y=w183:dbl)
                                n905 = Wait (ms)(milliseconds to wait=w183) -> ()  [unwired: 1 out]
                              }
                              frame #2 {
                                n906 = local read "Aktuelle L/2-Position [°]"() -> (w188:dbl)
                                n907 = local read "Aktueller Messschritt"() -> (w193:i32)
                                n908 = local read "Start time [ms]"() -> (w195:timestamp)
                                n909 = local read "# Messschritte"() -> (w194:i32)
                                n910 = invoke class="MG17Motor" method="GetPosition"(reference=w191, "lChanID"=w190, "pfPosition"=w188) -> ("pfPosition"=w189:sgl)  [unwired: 2 in, 4 out]
                                n911 = call "estimate_stopp_time.vi"("Aktueller Messschritt"=w193, "# Messschritte"=w194, "Startzeit"=w195) -> ("Stopp Zeit"=w192:string)  [unwired: 8 in]
                                n912 = local write "Geschätzte Messzeit"(w192) -> ()
                                n913 = local write "Aktuelle L/2-Position [°]"(w189) -> ()
                              }
                            }
                          }
                        }
                      }
                      frame #1 {
                        (unwired) T7 {"Summierte Helligkeit (a.u.)"=0, "Aktuelle L/2-Position [°]"=0.0}
                      }
                    }
                  }
                }
              }
              frame #1 {
                n914 = flat-sequence {
                  frame #0 {
                    # "Zur Ausgangsposition zurückfahren"
                    n915 = local read "Wellenplatte [°]"() -> (w206:refnum<k7>)
                    n916 = local read "L/2-Start [°]"() -> (w200:dbl)
                    n917 = invoke class="MG17Motor" method="SetAbsMovePos"(reference=w206, "lChanID"=0, "fAbsPos"=w200) -> (reference out=w204:refnum<k7>, error out=w201:errorcluster, "lChanID"=w202:i32)  [unwired: 2 in, 2 out]
                    n918 = local read "Aktuelle L/2-Position [°]"() -> (w198:dbl)
                    n919 = invoke class="MG17Motor" method="MoveAbsolute"(reference=w204, error in=w201, "lChanID"=w202, "bWait"=TRUE) -> (reference out=w197:refnum<k7>, "lChanID"=w196:i32)  [unwired: 1 in, 3 out]
                    n920 = invoke class="MG17Motor" method="GetPosition"(reference=w197, "lChanID"=w196, "pfPosition"=w198) -> ("pfPosition"=w199:sgl)  [unwired: 2 in, 4 out]
                    n921 = local write "Aktuelle L/2-Position [°]"(w199) -> ()
                  }
                  frame #1 {
                    n922 = local read "Leistungs-/Polarisationscan läuft"() -> (w209:bool)
                    n923 = local read "Leistungs-/Polarisationscan läuft"() -> (w211:bool)
                    n924 = local read "Summierte Helligkeit speichern"() -> (w208:bool)
                    n925 = local read "Daten speichern"() -> (w212:bool)
                    n926 = And(x=w208, y=w209) -> (x .and. y?=w207:bool)
                    n927 = case shown="True" w207 {
                      frame #0 {
                      }
                      frame #1 {
                        n928 = local read "Save folder"() -> (w213:string)
                        n929 = local read "Vektor Summierte Helligkeit [a.u.]"() -> (w214:dbl[])
                        n930 = Concatenate Strings(w213, "\\" ("String"), "2D_Intensitaetsverteilung_MCP.dat" ("String")) -> (w218:string)
                        n931 = String To Path(string=w218) -> (path=w217:path)
                        n932 = call-poly <vilib>:"Write To Spreadsheet File.vi"("format (%.3f)"="%.;%8.0f", "1D data"=w214, "file path (dialog if empty)"=w217) -> ()  [unwired: 5 in, 1 out]
                      }
                    }
                    n933 = And(x=w212, y=w211) -> (x .and. y?=w210:bool)
                    n934 = case shown="True" w210 {
                      frame #0 {
                        n935 = local read "# L/2-Schritte"() -> (w222:i32)
                        n936 = local read "L/2-Schritt [°]"() -> (w221:dbl)
                        n937 = local read "L/2-Start [°]"() -> (w220:dbl)
                        n938 = local read "Save folder"() -> (w223:string)
                        n939 = call "create_axis_vector_file.vi"("Save folder"=w223, "Dateiname"="xAchse.dat", "Start"=w220, "Schrittlänge"=w221, "# Schritte"=w222) -> ()  [unwired: 11 in]
                      }
                      frame #1 {
                      }
                    }
                  }
                  frame #2 {
                    n940 = local read "# L/2-Schritte"() -> (w226:i32)
                    n941 = Decrement(x=w226) -> (x-1=w225:i32)
                    n942 = local write "# L/2-Schritte"(w225) -> ()
                  }
                  frame #3 {
                    n943 = local read "Detektionskamera"() -> (w228:T5)
                    n944 = local read "Buffer Interval"() -> (w229:u32)
                    n945 = call "camera_create_configuration.vi"("BufferInterval"=w229, "Session Out 2"=w228) -> ("Fehler (Ausgang)"=w230:errorcluster, "Ereignisregistrierung (Referenz)"=w227:refnum<event-registration>)  [unwired: 1 in, 1 out]
                    n946 = local write "Ereignis: FrameDone?"(w227) -> ()
                    n947 = local write "Fehler (Ausgang)"(w230) -> ()
                  }
                  frame #4 {
                    w231 = FALSE ("Spannungsscan läuft")
                    n948 = local write "Leistungs-/Polarisationsscan ON/OFF"(w231) -> ()
                    n949 = local write "Leistungs-/Polarisationscan läuft"(w231) -> ()
                  }
                }
              }
            }
          }
          frame #1 {
          }
        }
      }
      n950 = while "x-U-Scan Schleife" {
        stop <- w233 stop-if-true
        n951 = local read "Fehler (Ausgang)"() -> (w234:errorcluster)
        n952 = local read "x-U-Scan läuft"() -> (w232:bool)
        n953 = local read "Programm beenden"() -> (w236:bool)
        n954 = case shown="True" w232 {
          frame #0 {
          }
          frame #1 {
            n955 = stacked-sequence {
              frame #0 {
                n956 = local read "# x-U-Scan x-Rasterschritte"() -> (w237:i32)
                n957 = for "Schleife für Raumkoordinate" {
                  N: w237 -> [_]
                  i -> [w238]
                  n958 = local read "x-U-Scan läuft"() -> (w239:bool)
                  n959 = case shown="True" w239 {
                    tunnel: w238 -> [_ w240]
                    frame #0 {
                    }
                    frame #1 {
                      n960 = stacked-sequence {
                        tunnel: w240 -> [w242 _]
                        frame #0 {
                          n961 = local read "# x-U-Scan Spannungsschritte"() -> (w241:i32)
                          n962 = for "Schleife für Spannungskoordinate" {
                            N: w241 -> [_]
                            tunnel: w242 -> [w244]
                            i -> [w243]
                            n963 = local read "x-U-Scan läuft"() -> (w245:bool)
                            n964 = case shown="True" w245 {
                              tunnel: w244 -> [_ w247]
                              tunnel: w243 -> [_ w246]
                              frame #0 {
                              }
                              frame #1 {
                                n965 = stacked-sequence {
                                tunnel: w247 -> [_ _ w291 _]
                                tunnel: w246 -> [_ _ w290 _]
                                frame #0 {
                                n966 = local write "Summierte Helligkeit (a.u.)"(u64 0 ("Summierte Helligkeit (a.u.)")) -> ()
                                n967 = local read "ROI"() -> (w253:i32[])
                                n968 = local read "Aktueller Messschritt"() -> (w250:i32)
                                n969 = Index Array(array=w253, index #1=0 ("Index"), index #2=1 ("Index")) -> (element #1=w257:i32, element #2=w256:i32)
                                n970 = Initialize Array(u64 0 ("Element"), w256, w257) -> (w251:u64[][])
                                n971 = local write "Gemitteltes Bild"(w251) -> ()
                                n972 = Increment(x=w250) -> (x+1=w249:i32)
                                n973 = local write "Aktueller Messschritt"(w249) -> ()
                                }
                                frame #1 {
                                n974 = local read "# Bilder/Messschritt"() -> (w261:i32)
                                n975 = local read "Detektionskamera"() -> (w264:T5)
                                n976 = local read "Einzelbilder speichern"() -> (w259:bool)
                                n977 = call "camera_acquisition_sequence.vi"("Session In"=w264, "Desired image number"=w261) -> ("Image Array"=w258:T4[], "error out"=w263:errorcluster)  [unwired: 2 in, 1 out]
                                n978 = case shown="True" w259 {
                                tunnel: w263 -> [w266 w274]
                                tunnel: [w266 w273] -> w262
                                tunnel: w261 -> [w265 w272]
                                tunnel: [w265 w272] -> w260
                                tunnel: w258 -> [_ w271]
                                frame #0 {
                                }
                                frame #1 {
                                n979 = local read "Aktueller Messschritt"() -> (w277:i32)
                                n980 = local read "Save folder"() -> (w269:string)
                                n981 = Concatenate Strings(w269, "Einzelbilder\\" ("String")) -> (w267:string)
                                n982 = Format Into String(format string="%05.0f" ("Format-String"), initial string="#" ("Eingangs-String"), w277) -> (resulting string=w270:string)  [unwired: 1 in, 1 out]
                                n983 = call "save images.vi"("Save Folder"=w267, "File name prefix"=w270, "Array"=w271, "error out 2"=w274, "Bilder/Messschritt"=w272) -> ("error out"=w273:errorcluster)
                                }
                                }
                                n984 = for {
                                N: w260 -> [_]
                                tunnel: w262 -> [w286]
                                tunnel: w258 -> [w284] mode=indexing
                                n985 = call "IMAQ ImageToArray"("error in (no error)"=w286, "Image"=w284) -> ("error out"=w285:errorcluster, "Image Pixels (U8)"=w283:u8[][])  [unwired: 2 in, 3 out]
                                n986 = local read "Gemitteltes Bild"() -> (w281:u64[][])
                                n987 = local read "Summierte Helligkeit (a.u.)"() -> (w288:i64)
                                n988 = local write "Fehler (Ausgang)"(w285) -> ()
                                n989 = To Quad Integer(1:w283) -> (0:w287:i64[][])
                                n990 = Add Array Elements(numeric array=w287) -> (sum=w280:i64)
                                n991 = Add(x=w281, y=w283) -> (x+y=w282:u64[][])
                                n992 = local write "Gemitteltes Bild"(w282) -> ()
                                n993 = local read "Hintergrund-Helligkeit"() -> (w278:i64)
                                n994 = Subtract(x=w280, y=w278) -> (x-y=w279:i64)
                                n995 = Add(x=w279, y=w288) -> (x+y=w289:i64)
                                n996 = local write "Summierte Helligkeit (a.u.)"(w289) -> ()
                                }
                                }
                                frame #2 {
                                n997 = local read "# Bilder/Messschritt"() -> (w297:i32)
                                n998 = local read "2D-Intensitätsverteilung (MCP)"() -> (w294:dbl[][])
                                n999 = local read "Gemitteltes Bild"() -> (w295:u64[][])
                                n1000 = local read "Summierte Helligkeit (a.u.)"() -> (w292:i64)
                                n1001 = local read "Gemittelte Bilder speichern"() -> (w301:bool)
                                n1002 = local read "Image Display"() -> (w299:T4)
                                n1003 = Divide(x=w295, y=w297) -> (x/y=w296:dbl[][])
                                n1004 = call "IMAQ ArrayToImage"("Image Pixels (U8)"=w296, "Image"=w299) -> ("Image Out"=w298:T4)  [unwired: 8 in, 1 out]
                                n1005 = Replace Array Subset(array=w294, new element=w292, index (row)=w291, index (col)=w290) -> (w293:dbl[][])
                                n1006 = local write "2D-Intensitätsverteilung (MCP)"(w293) -> ()
                                n1007 = case shown="True" w301 {
                                tunnel: w298 -> [w302 w313]
                                tunnel: [w302 w304] -> w300
                                frame #0 {
                                }
                                frame #1 {
                                n1008 = local read "Aktueller Messschritt"() -> (w308:i32)
                                n1009 = local read "Save folder"() -> (w310:string)
                                n1010 = Format Into String(format string="%05.0f" ("Format-String"), initial string="#" ("Eingangs-String"), w308) -> (resulting string=w307:string)  [unwired: 1 in, 1 out]
                                n1011 = Concatenate Strings(w310, "Gemittelte Bilder\\" ("String"), w307, ".png" ("String")) -> (w306:string)
                                n1012 = String To Path(string=w306) -> (path=w305:path)
                                n1013 = call-poly "IMAQ Write File 2"("File Path"=w305, "Image"=w313) -> ("Image Out (duplicate)"=w304:T4)  [unwired: 8 in, 1 out]
                                }
                                }
                                n1014 = local write "Image Display"(w300) -> ()
                                }
                                frame #3 {
                                n1015 = flat-sequence {
                                frame #0 {
                                n1016 = local read "x-U-Scan aktuelle Spannung [V]"() -> (w316:dbl)
                                n1017 = local read "x-U-Scan Spannungsschritt [V]"() -> (w317:dbl)
                                n1018 = local read "Spannungskanal"() -> (w315:refnum<k21>)
                                n1019 = Add(x=w316, y=w317) -> (x+y=w314:dbl)
                                n1020 = local write "x-U-Scan aktuelle Spannung [V]"(w314) -> ()
                                n1021 = call "HV_power_supply_set_voltage.vi"("Desired output voltage in V (HV power supply)"=w314, "Channel of HV power supply"=w315) -> ("error out"=w318:errorcluster)  [unwired: 8 in]
                                n1022 = local write "Fehler (Ausgang)"(w318) -> ()
                                }
                                frame #1 {
                                # "Wartezeit für\nneue Spannung"
                                n1023 = Wait (ms)(milliseconds to wait=u32 200 ("Zu wartende ms")) -> ()  [unwired: 1 out]
                                }
                                frame #2 {
                                n1024 = local read "Aktueller Messschritt"() -> (w321:i32)
                                n1025 = local read "Start time [ms]"() -> (w323:timestamp)
                                n1026 = local read "# Messschritte"() -> (w322:i32)
                                n1027 = call "estimate_stopp_time.vi"("Aktueller Messschritt"=w321, "# Messschritte"=w322, "Startzeit"=w323) -> ("Stopp Zeit"=w320:string)  [unwired: 8 in]
                                n1028 = local write "Geschätzte Messzeit"(w320) -> ()
                                }
                                }
                                }
                                }
                              }
                            }
                          }
                        }
                        frame #1 {
                          n1029 = flat-sequence {
                            frame #0 {
                              n1030 = local read "x-U-Scan Spannungsstart [V]"() -> (w324:dbl)
                              n1031 = local read "Spannungskanal"() -> (w325:refnum<k21>)
                              n1032 = local write "x-U-Scan aktuelle Spannung [V]"(w324) -> ()
                              n1033 = call "HV_power_supply_set_voltage.vi"("Desired output voltage in V (HV power supply)"=w324, "Channel of HV power supply"=w325) -> ("error out"=w326:errorcluster)  [unwired: 8 in]
                              n1034 = local write "Fehler (Ausgang)"(w326) -> ()
                            }
                            frame #1 {
                              # "Fahre nächste x-Position an"
                              n1035 = local read "x-U-Scan x-Rasterschritt [µm]"() -> (w331:dbl)
                              n1036 = local read "Achs-ID"() -> (w330:i32)
                              n1037 = Decrement(x=w330) -> (x-1=w329:i32)
                              n1038 = call "stage_move_axis_relative.vi"("Achse"=w330, "Schrittweite [µm]"=w331) -> ("xyz-Position OUT [mm]"=w328:dbl[])  [unwired: 1 in, 2 out]
                              n1039 = Index Array(array=w328, index=w329) -> (element=w327:dbl)
                              n1040 = local write "x-U-Scan aktuelle x-Position [mm]"(w327) -> ()
                            }
                            frame #2 {
                              n1041 = local read "x-U-Scan (Ausgleichslage) Steigung"() -> (w333:dbl)
                              n1042 = Not Equal?(x=w333, y=0.0) -> (x != y?=w334:bool)
                              n1043 = case shown="True" w334 {
                                frame #0 {
                                }
                                frame #1 {
                                # "Fahre nächste y-Position an"
                                n1044 = local read "Raum-Koordinate 2 (Lagenausgleich)"() -> (w335:enum16{"x-Achse", "y-Achse", "z-Achse"})
                                n1045 = local read "x-U-Scan (Ausgleichslage) Steigung"() -> (w337:dbl)
                                n1046 = local read "x-U-Scan x-Rasterschritt [µm]"() -> (w339:dbl)
                                n1047 = Multiply(x=w339, y=w337) -> (x*y=w338:dbl)
                                n1048 = Increment(x=w335) -> (x+1=w336:enum16{"x-Achse", "y-Achse", "z-Achse"})
                                n1049 = call "stage_move_axis_relative.vi"("Achse"=w336, "Schrittweite [µm]"=w338) -> ("xyz-Position OUT [mm]"=w340:dbl[])  [unwired: 1 in, 2 out]
                                n1050 = Index Array(array=w340, index=w335) -> (element=w341:dbl)
                                n1051 = local write "x-U-Scan aktuelle y-Position [mm]"(w341) -> ()
                                }
                              }
                            }
                            frame #3 {
                              # "Wartezeit für\nStartspannung"
                              n1052 = Wait (ms)(milliseconds to wait=u32 6000 ("Zu wartende ms")) -> ()  [unwired: 1 out]
                            }
                          }
                        }
                      }
                    }
                  }
                }
              }
              frame #1 {
                n1053 = local read "x-U-Scan läuft"() -> (w343:bool)
                n1054 = case shown="True" w343 {
                  frame #0 {
                    n1055 = flat-sequence {
                      frame #0 {
                        # "Zur Ausgangsposition zurückfahren"
                        n1056 = local read "x-U-Scan x-Startposition [mm]"() -> (w344:dbl)
                        n1057 = local read "Aktuelle xyz-Position [mm]"() -> (w347:dbl[])
                        n1058 = local read "Achs-ID"() -> (w345:i32)
                        n1059 = local read "x-U-Scan Spannungsstart [V]"() -> (w351:dbl)
                        n1060 = Decrement(x=w345) -> (x-1=w346:i32)
                        n1061 = Replace Array Subset(array=w347, new element=w344, index=w346) -> (w348:dbl[])
                        n1062 = local read "Detektionskamera"() -> (w355:T5)
                        n1063 = local read "Buffer Interval"() -> (w354:u32)
                        n1064 = call "stage_move_axis_absolute.vi"("Ziel xyz IN [mm]"=w348, "Achse"=w345) -> ("error out"=w349:errorcluster)  [unwired: 1 in, 2 out]
                        n1065 = local write "x-U-Scan aktuelle Spannung [V]"(w351) -> ()
                        n1066 = local read "Spannungskanal"() -> (w352:refnum<k21>)
                        n1067 = call "camera_create_configuration.vi"("error in"=w349, "BufferInterval"=w354, "Session Out 2"=w355) -> ("Fehler (Ausgang)"=w353:errorcluster, "Ereignisregistrierung (Referenz)"=w356:refnum<event-registration>)  [unwired: 1 out]
                        n1068 = local write "Ereignis: FrameDone?"(w356) -> ()
                        n1069 = call "HV_power_supply_set_voltage.vi"("error in"=w353, "Desired output voltage in V (HV power supply)"=w351, "Channel of HV power supply"=w352) -> ("error out"=w350:errorcluster)  [unwired: 7 in]
                        n1070 = local write "Fehler (Ausgang)"(w350) -> ()
                      }
                    }
                  }
                  frame #1 {
                    n1071 = flat-sequence {
                      frame #0 {
                        n1072 = local read "2D-Intensitätsverteilung (MCP)"() -> (w357:dbl[][])
                        n1073 = control-ref of="2D-Intensitätsverteilung (MCP)"() -> (w360:refnum<vi>)
                        n1074 = Array Max & Min(array=w357) -> (max value=w358:dbl, min value=w359:dbl)  [unwired: 2 out]
                        n1075 = property class="IntGraph (strikt)"(reference=w360, "ZScale.Maximum"=w358, "ZScale.Minimum"=w359) -> ()  [unwired: 1 in, 2 out]
                      }
                      frame #1 {
                        # "Zur Ausgangsposition zurückfahren"
                        n1076 = local read "Start xyz-Position [mm]"() -> (w365:dbl[])
                        n1077 = local read "x-U-Scan Spannungsstart [V]"() -> (w370:dbl)
                        n1078 = local read "x-U-Scan Spannungsstart [V]"() -> (w368:dbl)
                        n1079 = local read "Detektionskamera"() -> (w373:T5)
                        n1080 = local read "Achs-ID"() -> (w362:i32)
                        n1081 = local read "Buffer Interval"() -> (w372:u32)
                        n1082 = local read "Spannungskanal"() -> (w369:refnum<k21>)
                        n1083 = Decrement(x=w362) -> (x-1=w363:i32)
                        n1084 = call "stage_move_axis_absolute.vi"("Ziel xyz IN [mm]"=w365, "Achse"=w362) -> ("error out"=w366:errorcluster, "Ziel xyz OUT [mm]"=w364:dbl[])  [unwired: 1 in, 1 out]
                        n1085 = local write "x-U-Scan aktuelle Spannung [V]"(w370) -> ()
                        n1086 = call "camera_create_configuration.vi"("error in"=w366, "BufferInterval"=w372, "Session Out 2"=w373) -> ("Fehler (Ausgang)"=w367:errorcluster, "Ereignisregistrierung (Referenz)"=w374:refnum<event-registration>)  [unwired: 1 out]
                        n1087 = Index Array(array=w364, index=w363) -> (element=w361:dbl)
                        n1088 = local write "x-U-Scan aktuelle x-Position [mm]"(w361) -> ()
                        n1089 = local write "x-U-Scan aktuelle Spannung [V]"(w368) -> ()
                        n1090 = local write "Ereignis: FrameDone?"(w374) -> ()
                        n1091 = call "HV_power_supply_set_voltage.vi"("error in"=w367, "Desired output voltage in V (HV power supply)"=w368, "Channel of HV power supply"=w369) -> ("error out"=w371:errorcluster)  [unwired: 7 in]
                        n1092 = local write "Fehler (Ausgang)"(w371) -> ()
                      }
                      frame #2 {
                        n1093 = local read "x-U-Scan (Ausgleichslage) Steigung"() -> (w376:dbl)
                        n1094 = Not Equal?(x=w376, y=0.0) -> (x != y?=w375:bool)
                        n1095 = case shown="True" w375 {
                          frame #0 {
                          }
                          frame #1 {
                            n1096 = local read "Raum-Koordinate 2 (Lagenausgleich)"() -> (w378:enum16{"x-Achse", "y-Achse", "z-Achse"})
                            n1097 = local read "Start xyz-Position [mm]"() -> (w380:dbl[])
                            n1098 = Increment(x=w378) -> (x+1=w379:enum16{"x-Achse", "y-Achse", "z-Achse"})
                            n1099 = call "stage_move_axis_absolute.vi"("Ziel xyz IN [mm]"=w380, "Achse"=w379) -> ("Ziel xyz OUT [mm]"=w381:dbl[])  [unwired: 1 in, 2 out]
                            n1100 = Index Array(array=w381, index=w378) -> (element=w382:dbl)
                            n1101 = local write "x-U-Scan aktuelle y-Position [mm]"(w382) -> ()
                          }
                        }
                      }
                      frame #3 {
                        n1102 = local read "Daten speichern"() -> (w383:bool)
                        n1103 = case shown="True" w383 {
                          frame #0 {
                          }
                          frame #1 {
                            n1104 = local read "x-U-Scan x-Rasterschritt [µm]"() -> (w391:dbl)
                            n1105 = local read "x-U-Scan (Ausgleichslage) Steigung"() -> (w385:dbl)
                            n1106 = local read "x-U-Scan Spannungsschritt [V]"() -> (w394:dbl)
                            n1107 = local read "# x-U-Scan Spannungsschritte"() -> (w393:i32)
                            n1108 = local read "x-U-Scan x-Startposition [mm]"() -> (w392:dbl)
                            n1109 = local read "x-U-Scan Spannungsstart [V]"() -> (w395:dbl)
                            n1110 = local read "# x-U-Scan x-Rasterschritte"() -> (w387:i32)
                            n1111 = Divide(x=w391, y=1000.0) -> (x/y=w388:dbl)
                            n1112 = local read "Save folder"() -> (w389:string)
                            n1113 = Not Equal?(x=w385, y=0.0) -> (x != y?=w386:bool)
                            n1114 = local read "2D-Intensitätsverteilung (MCP)"() -> (w402:dbl[][])
                            n1115 = call "create_axis_vector_file.vi"("Save folder"=w389, "Dateiname"="yAchse.dat", "Start"=w395, "Schrittlänge"=w394, "# Schritte"=w393) -> ()  [unwired: 11 in]
                            n1116 = case shown="True" w386 {
                              tunnel: w389 -> [_ w410]
                              tunnel: w388 -> [_ w407]
                              tunnel: w387 -> [_ w404]
                              frame #0 {
                              }
                              frame #1 {
                                n1117 = local read "x-U-Scan (Ausgleichslage) Steigung"() -> (w408:dbl)
                                n1118 = local read "x-U-Scan y-Startposition [mm]"() -> (w405:dbl)
                                n1119 = Multiply(x=w407, y=w408) -> (x*y=w406:dbl)
                                n1120 = call "create_axis_vector_file.vi"("Save folder"=w410, "Dateiname"="zAchse.dat", "Start"=w405, "Schrittlänge"=w406, "# Schritte"=w404) -> ()  [unwired: 11 in]
                              }
                            }
                            n1121 = call "create_axis_vector_file.vi"("Save folder"=w389, "Dateiname"="xAchse.dat", "Start"=w392, "Schrittlänge"=w388, "# Schritte"=w387) -> ()  [unwired: 11 in]
                            n1122 = Concatenate Strings(w389, "\\" ("String"), "2D_Intensitaetsverteilung_MCP.dat" ("String")) -> (w399:string)
                            n1123 = String To Path(string=w399) -> (path=w400:path)
                            n1124 = call-poly <vilib>:"Write To Spreadsheet File.vi"("format (%.3f)"="%.;%8.0f", "2D data"=w402, "file path (dialog if empty)"=w400) -> ()  [unwired: 5 in, 1 out]
                          }
                        }
                      }
                      frame #4 {
                        w411 = FALSE ("Spannungsscan läuft")
                        n1125 = local write "x-U-Scan ON/OFF"(w411) -> ()
                        n1126 = local write "x-U-Scan läuft"(w411) -> ()
                      }
                    }
                  }
                }
              }
            }
          }
        }
        n1127 = Unbundle By Name(w234) -> ("status"=w235:bool)
        n1128 = Or(x=w235, y=w236) -> (x .or. y?=w233:bool)
      }
      n1129 = while "Spannungsscan-Schleife" {
        stop <- w413 stop-if-true
        n1130 = local read "Fehler (Ausgang)"() -> (w414:errorcluster)
        n1131 = local read "Spannungsscan läuft"() -> (w412:bool)
        n1132 = local read "Programm beenden"() -> (w416:bool)
        n1133 = Unbundle By Name(w414) -> ("status"=w415:bool)
        n1134 = Or(x=w415, y=w416) -> (x .or. y?=w413:bool)
        n1135 = case shown="True" w412 {
          frame #0 {
          }
          frame #1 {
            n1136 = stacked-sequence {
              frame #0 {
                n1137 = local read "# Spannungsschritte"() -> (w421:i32[])
                n1138 = Index Array(array=w421, index #1=0 ("Index"), index #2=1 ("Index")) -> (element #1=w418:i32, element #2=w417:i32)
                n1139 = for "Schleife für Tip-Spannung" {
                  N: w418 -> [_]
                  tunnel: w417 -> [w422]
                  i -> [w423]
                  n1140 = local read "Spannungsscan läuft"() -> (w424:bool)
                  n1141 = case shown="True" w424 {
                    tunnel: w423 -> [_ w426]
                    tunnel: w422 -> [_ w425]
                    frame #0 {
                    }
                    frame #1 {
                      n1142 = stacked-sequence {
                        tunnel: w426 -> [w428 _]
                        tunnel: w425 -> [w427 _]
                        frame #0 {
                          n1143 = for "Schleife für Suppressor-Spannung" {
                            N: w427 -> [_]
                            tunnel: w428 -> [w430]
                            i -> [w429]
                            n1144 = local read "Spannungsscan läuft"() -> (w431:bool)
                            n1145 = case shown="True" w431 {
                              tunnel: w430 -> [_ w433]
                              tunnel: w429 -> [_ w432]
                              frame #0 {
                              }
                              frame #1 {
                                n1146 = stacked-sequence {
                                tunnel: w433 -> [_ _ w477 _]
                                tunnel: w432 -> [_ _ w476 _]
                                frame #0 {
                                n1147 = local write "Summierte Helligkeit (a.u.)"(u64 0 ("Summierte Helligkeit (a.u.)")) -> ()
                                n1148 = local read "ROI"() -> (w439:i32[])
                                n1149 = local read "Aktueller Messschritt"() -> (w436:i32)
                                n1150 = Index Array(array=w439, index #1=0 ("Index"), index #2=1 ("Index")) -> (element #1=w443:i32, element #2=w442:i32)
                                n1151 = Initialize Array(u64 0 ("Element"), w442, w443) -> (w437:u64[][])
                                n1152 = local write "Gemitteltes Bild"(w437) -> ()
                                n1153 = Increment(x=w436) -> (x+1=w435:i32)
                                n1154 = local write "Aktueller Messschritt"(w435) -> ()
                                }
                                frame #1 {
                                n1155 = local read "# Bilder/Messschritt"() -> (w447:i32)
                                n1156 = local read "Detektionskamera"() -> (w450:T5)
                                n1157 = local read "Einzelbilder speichern"() -> (w445:bool)
                                n1158 = call "camera_acquisition_sequence.vi"("Session In"=w450, "Desired image number"=w447) -> ("Image Array"=w444:T4[], "error out"=w449:errorcluster)  [unwired: 2 in, 1 out]
                                n1159 = case shown="True" w445 {
                                tunnel: w449 -> [w452 w460]
                                tunnel: [w452 w459] -> w448
                                tunnel: w447 -> [w451 w458]
                                tunnel: [w451 w458] -> w446
                                tunnel: w444 -> [_ w457]
                                frame #0 {
                                }
                                frame #1 {
                                n1160 = local read "Aktueller Messschritt"() -> (w463:i32)
                                n1161 = local read "Save folder"() -> (w455:string)
                                n1162 = Concatenate Strings(w455, "Einzelbilder\\" ("String")) -> (w453:string)
                                n1163 = Format Into String(format string="%05.0f" ("Format-String"), initial string="#" ("Eingangs-String"), w463) -> (resulting string=w456:string)  [unwired: 1 in, 1 out]
                                n1164 = call "save images.vi"("Save Folder"=w453, "File name prefix"=w456, "Array"=w457, "error out 2"=w460, "Bilder/Messschritt"=w458) -> ("error out"=w459:errorcluster)
                                }
                                }
                                n1165 = for {
                                N: w446 -> [_]
                                tunnel: w448 -> [w472]
                                tunnel: w444 -> [w470] mode=indexing
                                n1166 = call "IMAQ ImageToArray"("error in (no error)"=w472, "Image"=w470) -> ("error out"=w471:errorcluster, "Image Pixels (U8)"=w469:u8[][])  [unwired: 2 in, 3 out]
                                n1167 = local read "Gemitteltes Bild"() -> (w467:u64[][])
                                n1168 = local write "Fehler (Ausgang)"(w471) -> ()
                                n1169 = To Quad Integer(1:w469) -> (0:w473:i64[][])
                                n1170 = Add Array Elements(numeric array=w473) -> (sum=w466:i64)
                                n1171 = local read "Summierte Helligkeit (a.u.)"() -> (w474:i64)
                                n1172 = Add(x=w467, y=w469) -> (x+y=w468:u64[][])
                                n1173 = local write "Gemitteltes Bild"(w468) -> ()
                                n1174 = local read "Hintergrund-Helligkeit"() -> (w464:i64)
                                n1175 = Subtract(x=w466, y=w464) -> (x-y=w465:i64)
                                n1176 = Add(x=w465, y=w474) -> (x+y=w475:i64)
                                n1177 = local write "Summierte Helligkeit (a.u.)"(w475) -> ()
                                }
                                }
                                frame #2 {
                                n1178 = local read "# Bilder/Messschritt"() -> (w483:i32)
                                n1179 = local read "2D-Intensitätsverteilung (MCP)"() -> (w480:dbl[][])
                                n1180 = local read "Gemitteltes Bild"() -> (w481:u64[][])
                                n1181 = local read "Summierte Helligkeit (a.u.)"() -> (w478:i64)
                                n1182 = local read "Gemittelte Bilder speichern"() -> (w487:bool)
                                n1183 = local read "Image Display"() -> (w485:T4)
                                n1184 = Divide(x=w481, y=w483) -> (x/y=w482:dbl[][])
                                n1185 = Replace Array Subset(array=w480, new element=w478, index (row)=w477, index (col)=w476) -> (w479:dbl[][])
                                n1186 = call "IMAQ ArrayToImage"("Image Pixels (U8)"=w482, "Image"=w485) -> ("Image Out"=w484:T4)  [unwired: 8 in, 1 out]
                                n1187 = local write "2D-Intensitätsverteilung (MCP)"(w479) -> ()
                                n1188 = case shown="True" w487 {
                                tunnel: w484 -> [w488 w499]
                                tunnel: [w488 w490] -> w486
                                frame #0 {
                                }
                                frame #1 {
                                n1189 = local read "Aktueller Messschritt"() -> (w494:i32)
                                n1190 = local read "Save folder"() -> (w496:string)
                                n1191 = Format Into String(format string="%05.0f" ("Format-String"), initial string="#" ("Eingangs-String"), w494) -> (resulting string=w493:string)  [unwired: 1 in, 1 out]
                                n1192 = Concatenate Strings(w496, "Gemittelte Bilder\\" ("String"), w493, ".png" ("String")) -> (w492:string)
                                n1193 = String To Path(string=w492) -> (path=w491:path)
                                n1194 = call-poly "IMAQ Write File 2"("File Path"=w491, "Image"=w499) -> ("Image Out (duplicate)"=w490:T4)  [unwired: 8 in, 1 out]
                                }
                                }
                                n1195 = local write "Image Display"(w486) -> ()
                                }
                                frame #3 {
                                n1196 = flat-sequence {
                                frame #0 {
                                n1197 = local read "Aktuelle Spannung [V]"() -> (w502:dbl[])
                                n1198 = local read "Spannungsschritt [V]"() -> (w506:dbl[])
                                n1199 = Index Array(array=w502, index=1 ("Index")) -> (element=w504:dbl)
                                n1200 = Index Array(array=w506, index=1 ("Index")) -> (element=w505:dbl)
                                n1201 = Add(x=w504, y=w505) -> (x+y=w500:dbl)
                                n1202 = local write "Suppressor-Spannung [V]"(w500) -> ()
                                n1203 = call "HV_power_supply_set_voltage.vi"("Desired output voltage in V (HV power supply)"=w500, "Channel of HV power supply"=refnum<k21> "Dev0/Ao0") -> ("error out"=w509:errorcluster)  [unwired: 8 in]
                                n1204 = local write "Fehler (Ausgang)"(w509) -> ()
                                n1205 = Replace Array Subset(array=w502, new element=w500, index=1 ("Index")) -> (w501:dbl[])
                                n1206 = local write "Aktuelle Spannung [V]"(w501) -> ()
                                }
                                frame #1 {
                                # "Wartezeit für\nneue Spannung"
                                n1207 = Wait (ms)(milliseconds to wait=u32 200 ("Zu wartende ms")) -> ()  [unwired: 1 out]
                                }
                                frame #2 {
                                n1208 = local read "Aktueller Messschritt"() -> (w513:i32)
                                n1209 = local read "Start time [ms]"() -> (w515:timestamp)
                                n1210 = local read "# Messschritte"() -> (w514:i32)
                                n1211 = call "estimate_stopp_time.vi"("Aktueller Messschritt"=w513, "# Messschritte"=w514, "Startzeit"=w515) -> ("Stopp Zeit"=w512:string)  [unwired: 8 in]
                                n1212 = local write "Geschätzte Messzeit"(w512) -> ()
                                }
                                }
                                }
                                }
                              }
                            }
                          }
                        }
                        frame #1 {
                          n1213 = flat-sequence {
                            frame #0 {
                              n1214 = local read "Spannungsstart [V]"() -> (w521:dbl[])
                              n1215 = local read "Aktuelle Spannung [V]"() -> (w523:dbl[])
                              n1216 = Index Array(array=w521, index=1 ("Index")) -> (element=w516:dbl)
                              n1217 = local write "Suppressor-Spannung [V]"(w516) -> ()
                              n1218 = call "HV_power_supply_set_voltage.vi"("Desired output voltage in V (HV power supply)"=w516, "Channel of HV power supply"=refnum<k21> "Dev0/Ao0") -> ("error out"=w517:errorcluster)  [unwired: 8 in]
                              n1219 = local write "Fehler (Ausgang)"(w517) -> ()
                              n1220 = Replace Array Subset(array=w523, new element=w516, index=1 ("Index")) -> (w519:dbl[])
                              n1221 = local write "Aktuelle Spannung [V]"(w519) -> ()
                            }
                            frame #1 {
                              n1222 = local read "Aktuelle Spannung [V]"() -> (w526:dbl[])
                              n1223 = local read "Spannungsschritt [V]"() -> (w530:dbl[])
                              n1224 = Index Array(array=w526, index=0 ("Index")) -> (element=w528:dbl)
                              n1225 = Index Array(array=w530, index=0 ("Index")) -> (element=w529:dbl)
                              n1226 = Add(x=w528, y=w529) -> (x+y=w524:dbl)
                              n1227 = local write "Tip-Spannung [V]"(w524) -> ()
                              n1228 = call "HV_power_supply_set_voltage.vi"("Desired output voltage in V (HV power supply)"=w524, "Channel of HV power supply"=refnum<k21> "Dev0/Ao1") -> ("error out"=w533:errorcluster)  [unwired: 8 in]
                              n1229 = local write "Fehler (Ausgang)"(w533) -> ()
                              n1230 = Replace Array Subset(array=w526, new element=w524, index=0 ("Index")) -> (w525:dbl[])
                              n1231 = local write "Aktuelle Spannung [V]"(w525) -> ()
                            }
                            frame #2 {
                              # "Wartezeit für\nStartspannung"
                              n1232 = Wait (ms)(milliseconds to wait=u32 6000 ("Zu wartende ms")) -> ()  [unwired: 1 out]
                            }
                          }
                        }
                      }
                    }
                  }
                }
              }
              frame #1 {
                n1233 = local read "Spannungsscan läuft"() -> (w536:bool)
                n1234 = case shown="False" w536 {
                  frame #0 {
                    n1235 = flat-sequence {
                      frame #0 {
                        # "Zur Ausgangsposition zurückfahren"
                        n1236 = local read "Spannungsstart [V]"() -> (w542:dbl[])
                        n1237 = local read "Spannungsstart [V]"() -> (w537:dbl[])
                        n1238 = local read "Detektionskamera"() -> (w549:T5)
                        n1239 = local read "Buffer Interval"() -> (w548:u32)
                        n1240 = local write "Aktuelle Spannung [V]"(w537) -> ()
                        n1241 = call "camera_create_configuration.vi"("BufferInterval"=w548, "Session Out 2"=w549) -> ("Fehler (Ausgang)"=w543:errorcluster, "Ereignisregistrierung (Referenz)"=w550:refnum<event-registration>)  [unwired: 1 in, 1 out]
                        n1242 = Index Array(array=w542, index #1=0 ("Index"), index #2=1 ("Index")) -> (element #1=w538:dbl, element #2=w539:dbl)
                        n1243 = local write "Tip-Spannung [V]"(w538) -> ()
                        n1244 = local write "Suppressor-Spannung [V]"(w539) -> ()
                        n1245 = local write "Ereignis: FrameDone?"(w550) -> ()
                        n1246 = call "HV_power_supply_set_voltage.vi"("error in"=w543, "Desired output voltage in V (HV power supply)"=w539, "Channel of HV power supply"=refnum<k21> "Dev0/Ao0") -> ("error out"=w545:errorcluster)  [unwired: 7 in]
                        n1247 = call "HV_power_supply_set_voltage.vi"("error in"=w545, "Desired output voltage in V (HV power supply)"=w538, "Channel of HV power supply"=refnum<k21> "Dev0/Ao1") -> ("error out"=w544:errorcluster)  [unwired: 7 in]
                        n1248 = local write "Fehler (Ausgang)"(w544) -> ()
                      }
                    }
                  }
                  frame #1 {
                    n1249 = flat-sequence {
                      frame #0 {
                        n1250 = local read "2D-Intensitätsverteilung (MCP)"() -> (w551:dbl[][])
                        n1251 = control-ref of="2D-Intensitätsverteilung (MCP)"() -> (w554:refnum<vi>)
                        n1252 = Array Max & Min(array=w551) -> (max value=w552:dbl, min value=w553:dbl)  [unwired: 2 out]
                        n1253 = property class="IntGraph (strikt)"(reference=w554, "ZScale.Maximum"=w552, "ZScale.Minimum"=w553) -> ()  [unwired: 1 in, 2 out]
                      }
                      frame #1 {
                        # "Zur Ausgangsposition zurückfahren"
                        n1254 = local read "Spannungsstart [V]"() -> (w555:dbl[])
                        n1255 = local read "Spannungsstart [V]"() -> (w560:dbl[])
                        n1256 = local read "Detektionskamera"() -> (w567:T5)
                        n1257 = local read "Buffer Interval"() -> (w566:u32)
                        n1258 = local write "Aktuelle Spannung [V]"(w555) -> ()
                        n1259 = call "camera_create_configuration.vi"("BufferInterval"=w566, "Session Out 2"=w567) -> ("Fehler (Ausgang)"=w561:errorcluster, "Ereignisregistrierung (Referenz)"=w568:refnum<event-registration>)  [unwired: 1 in, 1 out]
                        n1260 = Index Array(array=w560, index #1=0 ("Index"), index #2=1 ("Index")) -> (element #1=w556:dbl, element #2=w557:dbl)
                        n1261 = local write "Tip-Spannung [V]"(w556) -> ()
                        n1262 = local write "Suppressor-Spannung [V]"(w557) -> ()
                        n1263 = local write "Ereignis: FrameDone?"(w568) -> ()
                        n1264 = call "HV_power_supply_set_voltage.vi"("error in"=w561, "Desired output voltage in V (HV power supply)"=w557, "Channel of HV power supply"=refnum<k21> "Dev0/Ao0") -> ("error out"=w563:errorcluster)  [unwired: 7 in]
                        n1265 = call "HV_power_supply_set_voltage.vi"("error in"=w563, "Desired output voltage in V (HV power supply)"=w556, "Channel of HV power supply"=refnum<k21> "Dev0/Ao1") -> ("error out"=w562:errorcluster)  [unwired: 7 in]
                        n1266 = local write "Fehler (Ausgang)"(w562) -> ()
                      }
                      frame #2 {
                        n1267 = local read "Daten speichern"() -> (w569:bool)
                        n1268 = case shown="True" w569 {
                          frame #0 {
                          }
                          frame #1 {
                            w570 = 1 ("Index")
                            w582 = 0 ("Index")
                            n1269 = local read "Spannungsschritt [V]"() -> (w580:dbl[])
                            n1270 = local read "# Spannungsschritte"() -> (w581:i32[])
                            n1271 = local read "Spannungsstart [V]"() -> (w579:dbl[])
                            n1272 = local read "Save folder"() -> (w571:string)
                            n1273 = Index Array(array=w579, index #1=w582, index #2=w570) -> (element #1=w578:dbl, element #2=w574:dbl)
                            n1274 = Index Array(array=w580, index #1=w582, index #2=w570) -> (element #1=w577:dbl, element #2=w573:dbl)
                            n1275 = Index Array(array=w581, index #1=w582, index #2=w570) -> (element #1=w576:i32, element #2=w572:i32)
                            n1276 = local read "2D-Intensitätsverteilung (MCP)"() -> (w588:dbl[][])
                            n1277 = call "create_axis_vector_file.vi"("Save folder"=w571, "Dateiname"="xAchse.dat" ("Save folder"), "Start"=w578, "Schrittlänge"=w577, "# Schritte"=w576) -> ()  [unwired: 11 in]
                            n1278 = call "create_axis_vector_file.vi"("Save folder"=w571, "Dateiname"="yAchse.dat", "Start"=w574, "Schrittlänge"=w573, "# Schritte"=w572) -> ()  [unwired: 11 in]
                            n1279 = Concatenate Strings(w571, "\\" ("String"), "2D_Intensitaetsverteilung_MCP.dat" ("String")) -> (w585:string)
                            n1280 = String To Path(string=w585) -> (path=w586:path)
                            n1281 = call-poly <vilib>:"Write To Spreadsheet File.vi"("format (%.3f)"="%.;%8.0f", "2D data"=w588, "file path (dialog if empty)"=w586) -> ()  [unwired: 5 in, 1 out]
                          }
                        }
                      }
                      frame #3 {
                        w590 = FALSE ("Spannungsscan läuft")
                        n1282 = local write "Spannungsscan ON/OFF"(w590) -> ()
                        n1283 = local write "Spannungsscan läuft"(w590) -> ()
                      }
                    }
                  }
                }
              }
            }
          }
        }
      }
      n1284 = while "Kamera-Schleife" {
        i -> [w1645]
        stop <- w1646 stop-if-true
        n1285 = local read "Fehler (Ausgang)"() -> (w1647:errorcluster)
        n1286 = local read "Ereignis: FrameDone?"() -> (w1650:refnum<event-registration>)
        n1287 = local read "Programm beenden"() -> (w1649:bool)
        n1288 = Unbundle By Name(w1647) -> ("status"=w1648:bool)
        n1289 = Or(x=w1648, y=w1649) -> (x .or. y?=w1646:bool)
        n1290 = event "Kamera-Ereignisse" shown="[1] \"Kamera ON/OFF\": Wertänderung" {
          selector: w1650 -> [_ _ _ _ _ _ _ _]
          dyn-events: _ -> [_ _ _ _ _ _ _ _]
          timeout: 1000 -> [_ _ _ _ _ _ _ _]
          event #0 {
            n1291 = event-data() -> ()  [unwired: 1 in, 2 out]
          }
          event #1 {
            n1292 = event-data() -> ()  [unwired: 1 in, 4 out]
            n1293 = local read "Detektionskamera"() -> (w1653:T5)
            n1294 = local read "Kamera ON/OFF"() -> (w1654:bool)
            n1295 = case shown="True" w1654 {
              tunnel: w1653 -> [w1655 w1661]
              tunnel: [w1658 w1662] -> w1652
              frame #0 {
                n1296 = local read "Image Memory"() -> (w1656:T4)
                n1297 = call "camera_release configuration_stop.vi"("Image Memory"=w1656, "Detektionskamera"=w1655) -> ("error out"=w1658:errorcluster, "status"=w1657:bool)
                n1298 = local write "Kamera"(w1657) -> ()
              }
              frame #1 {
                n1299 = local read "Buffer Interval"() -> (w1660:u32)
                n1300 = local read "Video Mode"() -> (w1659:u32)
                n1301 = call "camera_acquisition_continously.vi"("Detektionskamera"=w1661, "BufferInterval"=w1660, "Video Mode"=w1659) -> ("Kamera eingeschaltet?"=w1666:bool, "Detektionskamera"=w1665:T5, "Image Memory"=w1664:T4, "Ereignis: FrameDone?"=w1663:refnum<event-registration>, "error out"=w1662:errorcluster)  [unwired: 1 in]
                n1302 = local write "Image Memory"(w1664) -> ()
                n1303 = local write "Detektionskamera"(w1665) -> ()
                n1304 = local write "Ereignis: FrameDone?"(w1663) -> ()
                n1305 = local write "Kamera"(w1666) -> ()
              }
            }
            n1306 = local write "Fehler (Ausgang)"(w1652) -> ()
          }
          event #2 {
            w1681 = IMAQdx_Buffer_Number_Mode."Buffer Number"  # Buffer Number Mode
            n1307 = event-data() -> ("ActualBufferNumber"=w1675:u32)  [unwired: 1 in]
            n1308 = local read "Detektionskamera"() -> (w1680:T5)
            n1309 = local read "Image Memory"() -> (w1679:T4)
            n1310 = call <vilib>:"IMAQdx Get Image.vi"("Buffer Number Mode (Next)"=w1681, "Buffer Number In"=w1675, "Image In"=w1679, "Session In"=w1680) -> ("error out"=w1673:errorcluster, "Buffer Number Out"=w1676:u32, "Image Out"=w1672:T4, "Session Out"=w1677:T5)  [unwired: 1 in, 3 out]
            n1311 = local write "Image Memory"(w1672) -> ()
            n1312 = local write "Detektionskamera"(w1677) -> ()
            n1313 = local write "Image Display"(w1672) -> ()
            n1314 = local write "Buffer Number"(w1676) -> ()
            n1315 = local write "Fehler (Ausgang)"(w1673) -> ()
            n1316 = Not Equal?(x=w1676, y=w1675) -> (x != y?=w1674:bool)
            n1317 = call "IMAQ ImageToArray"("Image"=w1672) -> ("Image Pixels (U8)"=w1669:u8[][])  [unwired: 3 in, 4 out]
            n1318 = call "CalculateFPS.vi"("buffer number"=w1676) -> ("processed FPS"=w1678:dbl)  [unwired: 2 out]
            n1319 = To Quad Integer(1:w1669) -> (0:w1668:i64[][])
            n1320 = local write "Buffer Overrun"(w1674) -> ()
            n1321 = local write "Frame Rate (FPS)"(w1678) -> ()
            n1322 = Add Array Elements(numeric array=w1668) -> (sum=w1671:i64)
            n1323 = local read "Hintergrund-Helligkeit"() -> (w1667:i64)
            n1324 = Subtract(x=w1671, y=w1667) -> (x-y=w1670:i64)
            n1325 = local write "Summierte Helligkeit (a.u.)"(w1670) -> ()
            n1326 = local write "Helligkeitsverlauf"(w1670) -> ()
          }
          event #3 {
            n1327 = event-data() -> ()  [unwired: 1 in, 2 out]
            n1328 = case shown="True" "Helligkeit nullen" {
              frame #0 {
              }
              frame #1 {
                n1329 = local read "Summierte Helligkeit (a.u.)"() -> (w1683:i64)
                n1330 = local write "Hintergrund-Helligkeit"(w1683) -> ()
              }
            }
          }
          event #4 {
            n1331 = event-data() -> ()  [unwired: 1 in, 2 out]
            n1332 = local read "Kamera"() -> (w1684:bool)
            n1333 = case shown="True" w1684 {
              frame #0 {
              }
              frame #1 {
                n1334 = control-ref of="Shutter time (ms)"() -> (w1691:refnum<vi>)
                n1335 = property class="Ring (strikt)"(reference=w1691) -> ("RingText.Text"=w1690:string)  [unwired: 1 in, 2 out]
                n1336 = local read "Detektionskamera"() -> (w1689:T5)
                n1337 = Decimal String To Number(string=w1690) -> (number=w1686:i32)  [unwired: 2 in, 1 out]
                n1338 = property class="IMAQdx"(reference=w1689, "ActiveAttribute"="CameraAttributes::Shutter::Value", "ValueDBL"=w1686) -> (reference out=w1688:T5, error out=w1685:errorcluster)  [unwired: 1 in]
                n1339 = local write "Detektionskamera"(w1688) -> ()
                n1340 = local write "Fehler (Ausgang)"(w1685) -> ()
              }
            }
          }
          event #5 {
            n1341 = event-data() -> ()  [unwired: 1 in, 1 out]
            n1342 = local read "Kamera ON/OFF"() -> (w1692:bool)
            n1343 = case shown="True" w1692 {
              frame #0 {
              }
              frame #1 {
                n1344 = flat-sequence {
                  frame #0 {
                    n1345 = local read "Detektionskamera"() -> (w1693:T5)
                    n1346 = local read "Image Memory"() -> (w1694:T4)
                    n1347 = call "camera_release configuration_stop.vi"("Image Memory"=w1694, "Detektionskamera"=w1693) -> ("status"=w1695:bool)  [unwired: 1 out]
                    n1348 = local write "Kamera"(w1695) -> ()
                  }
                  frame #1 {
                    n1349 = local read "Detektionskamera"() -> (w1696:T5)
                    n1350 = control-ref of="Shutter time (ms)"() -> (w1699:refnum<vi>)
                    n1351 = property class="Ring (strikt)"(reference=w1699) -> ("RingText.Text"=w1698:string)  [unwired: 1 in, 2 out]
                    n1352 = local read "Buffer Interval"() -> (w1702:u32)
                    n1353 = local read "Video Mode"() -> (w1701:u32)
                    n1354 = Decimal String To Number(string=w1698) -> (number=w1697:i32)  [unwired: 2 in, 1 out]
                    n1355 = call "camera_acquisition_continously.vi"("Detektionskamera"=w1696, "BufferInterval"=w1702, "Video Mode"=w1701, "Shutter time (ms)"=w1697) -> ("Kamera eingeschaltet?"=w1706:bool, "Detektionskamera"=w1705:T5, "Image Memory"=w1704:T4, "Ereignis: FrameDone?"=w1703:refnum<event-registration>, "error out"=w1700:errorcluster)
                    n1356 = local write "Image Memory"(w1704) -> ()
                    n1357 = local write "Detektionskamera"(w1705) -> ()
                    n1358 = local write "Ereignis: FrameDone?"(w1703) -> ()
                    n1359 = local write "Fehler (Ausgang)"(w1700) -> ()
                    n1360 = local write "Kamera"(w1706) -> ()
                  }
                }
              }
            }
          }
          event #6 {
            n1361 = event-data() -> ()  [unwired: 1 in, 1 out]
            n1362 = local read "Kamera"() -> (w1707:bool)
            n1363 = case shown="True" w1707 {
              frame #0 {
              }
              frame #1 {
                n1364 = local read "Ereignis: FrameDone?"() -> (w1709:refnum<event-registration>)
                n1365 = local read "Detektionskamera"() -> (w1713:T5)
                n1366 = local read "Buffer Interval"() -> (w1712:u32)
                n1367 = local read "ROI"() -> (w1714:i32[])
                n1368 = call "camera_change_ROI.vi"("BufferInterval"=w1712, "Region of Interest"=w1714, "Ereignisregistrierung (Referenz) 2"=w1709, "Session In"=w1713) -> ("Fehler (Ausgang)"=w1708:errorcluster, "Ereignisregistrierung (Referenz)"=w1711:refnum<event-registration>, "Session Out"=w1710:T5)  [unwired: 5 in]
                n1369 = local write "Detektionskamera"(w1710) -> ()
                n1370 = local write "Ereignis: FrameDone?"(w1711) -> ()
                n1371 = local write "Fehler (Ausgang)"(w1708) -> ()
              }
            }
          }
          event #7 {
            n1372 = event-data() -> ("NewVal"=w1716:bool)  [unwired: 1 in, 1 out]
            n1373 = local read "Kamera"() -> (w1717:bool)
            n1374 = And(x=w1717, y=w1716) -> (x .and. y?=w1715:bool)
            n1375 = case shown="True" w1715 {
              frame #0 {
              }
              frame #1 {
                w1718 = i32[] [640, 480, 0, 0] ("Region of Interest (px)")
                n1376 = local read "Ereignis: FrameDone?"() -> (w1720:refnum<event-registration>)
                n1377 = local read "Detektionskamera"() -> (w1724:T5)
                n1378 = local read "Buffer Interval"() -> (w1723:u32)
                n1379 = call "camera_change_ROI.vi"("BufferInterval"=w1723, "Region of Interest"=w1718, "Ereignisregistrierung (Referenz) 2"=w1720, "Session In"=w1724) -> ("Fehler (Ausgang)"=w1719:errorcluster, "Ereignisregistrierung (Referenz)"=w1722:refnum<event-registration>, "Session Out"=w1721:T5)  [unwired: 5 in]
                n1380 = local write "ROI"(w1718) -> ()
                n1381 = local write "Detektionskamera"(w1721) -> ()
                n1382 = local write "Ereignis: FrameDone?"(w1722) -> ()
                n1383 = local write "Fehler (Ausgang)"(w1719) -> ()
              }
            }
          }
        }
        "Kameraschleifenzähler" <- w1645
      }
      n1384 = while "Steuerungs-Schleife" {
        i -> [w592]
        stop <- w591 stop-if-true
        n1385 = event shown="[0] \"HV ON/OFF\": Wertänderung" {
          selector: _ -> [_ _ _ _ _]
          dyn-events: _ -> [_ _ _ _ _]
          timeout: 1000 -> [_ _ _ _ _]
          event #0 {
            w597 = 0.0 ("Suppressor-Spannung [V]")
            n1386 = event-data() -> ("NewVal"=w598:bool)  [unwired: 1 in]
            n1387 = local write "HV-Steuerung"(w598) -> ()
            n1388 = local write "Suppressor-Spannung [V]"(w597) -> ()
            n1389 = local write "Tip-Spannung [V]"(w597) -> ()
            n1390 = call "HV_power_supply_set_voltage.vi"("Desired output voltage in V (HV power supply)"=0.0, "Channel of HV power supply"=refnum<k21> "Dev0/Ao0") -> ("error out"=w600:errorcluster)  [unwired: 8 in]
            n1391 = call "HV_power_supply_set_voltage.vi"("error in"=w600, "Desired output voltage in V (HV power supply)"=0.0, "Channel of HV power supply"=refnum<k21> "Dev0/Ao1") -> ("error out"=w599:errorcluster)  [unwired: 7 in]
            n1392 = local write "Fehler (Ausgang)"(w599) -> ()
          }
          event #1 {
            n1393 = event-data() -> ("NewVal"=w605:bool)  [unwired: 1 in]
            n1394 = case shown="True" w605 {
              frame #0 {
                n1395 = local read "Wellenplatte [°]"() -> (w608:refnum<k7>)
                n1396 = invoke class="MG17Motor" method="StopCtrl"(reference=w608) -> (error out=w607:errorcluster)  [unwired: 2 in, 2 out]
                n1397 = Unbundle By Name(w607) -> ("status"=w606:bool)
                n1398 = local write "Wellenplatte"(w606) -> ()
              }
              frame #1 {
                n1399 = property class="MG17Motor"(reference="Wellenplatte [°]", "HWSerialNum"="SN von Rotationsbühne") -> (reference out=w615:refnum<k7>, error out=w614:errorcluster)  [unwired: 1 in]
                n1400 = invoke class="MG17Motor" method="StartCtrl"(reference=w615, error in=w614) -> (error out=w613:errorcluster)  [unwired: 1 in, 2 out]
                n1401 = local write "Fehler (Ausgang)"(w613) -> ()
                n1402 = Unbundle By Name(w613) -> ("status"=w612:bool)
                n1403 = Not(x=w612) -> (.not. x?=w611:bool)
                n1404 = local write "Wellenplatte"(w611) -> ()
              }
            }
          }
          event #2 {
            n1405 = event-data() -> ("OldVal"=w616:dbl, "NewVal"=w622:dbl)  [unwired: 1 in]
            n1406 = local read "Suppressor-Spannung [V]"() -> (w621:dbl)
            n1407 = local read "Max. Spannungsdifferenz"() -> (w619:dbl)
            n1408 = local read "HV-Steuerung"() -> (w617:bool)
            n1409 = Subtract(x=w622, y=w621) -> (x-y=w620:dbl)
            n1410 = Less Or Equal?(x=w620, y=w619) -> (x <= y?=w618:bool)
            n1411 = case shown="True" w617 {
              tunnel: w618 -> [_ w624]
              tunnel: w616 -> [_ w623]
              frame #0 {
              }
              frame #1 {
                n1412 = case shown="True" w624 {
                  tunnel: w623 -> [w625 _]
                  frame #0 {
                    n1413 = local write "Tip-Spannung [V]"(w625) -> ()
                  }
                  frame #1 {
                    n1414 = local read "Tip-Spannung [V]"() -> (w626:dbl)
                    n1415 = call "HV_power_supply_set_voltage.vi"("Desired output voltage in V (HV power supply)"=w626, "Channel of HV power supply"=refnum<k21> "Dev0/Ao1") -> ("error out"=w627:errorcluster)  [unwired: 8 in]
                    n1416 = local write "Fehler (Ausgang)"(w627) -> ()
                  }
                }
              }
            }
          }
          event #3 {
            n1417 = event-data() -> ("OldVal"=w629:dbl, "NewVal"=w631:dbl)  [unwired: 1 in]
            n1418 = local read "Tip-Spannung [V]"() -> (w630:dbl)
            n1419 = local read "Max. Spannungsdifferenz"() -> (w632:dbl)
            n1420 = Subtract(x=w630, y=w631) -> (x-y=w634:dbl)
            n1421 = local read "HV-Steuerung"() -> (w635:bool)
            n1422 = Less Or Equal?(x=w634, y=w632) -> (x <= y?=w633:bool)
            n1423 = case shown="True" w635 {
              tunnel: w633 -> [_ w637]
              tunnel: w629 -> [_ w636]
              frame #0 {
              }
              frame #1 {
                n1424 = case shown="True" w637 {
                  tunnel: w636 -> [w638 _]
                  frame #0 {
                    n1425 = local write "Suppressor-Spannung [V]"(w638) -> ()
                  }
                  frame #1 {
                    n1426 = local read "Suppressor-Spannung [V]"() -> (w639:dbl)
                    n1427 = call "HV_power_supply_set_voltage.vi"("Desired output voltage in V (HV power supply)"=w639, "Channel of HV power supply"=refnum<k21> "Dev0/Ao0") -> ("error out"=w640:errorcluster)  [unwired: 8 in]
                    n1428 = local write "Fehler (Ausgang)"(w640) -> ()
                  }
                }
              }
            }
          }
          event #4 {
            n1429 = event-data() -> ()  [unwired: 1 in, 2 out]
          }
        }
        n1430 = local read "Fehler (Ausgang)"() -> (w596:errorcluster)
        n1431 = local read "Programm beenden"() -> (w595:bool)
        n1432 = Unbundle By Name(w596) -> ("status"=w594:bool)
        n1433 = Or(x=w594, y=w595) -> (x .or. y?=w591:bool)
        "Steuerschleifenzähler" <- w592
      }
      n1434 = while {
        stop <- w31 stop-if-true
        n1435 = event shown="[1] \"Log-Plot\": Wertänderung" {
          selector: _ -> [_ _]
          dyn-events: _ -> [_ _]
          timeout: 100 -> [_ _]
          event #0 {
            n1436 = event-data() -> ()  [unwired: 1 in, 2 out]
          }
          event #1 {
            n1437 = event-data() -> ("NewVal"=w41:bool)  [unwired: 1 in, 4 out]
            n1438 = Boolean To (0,1)(Boolean=w41) -> (0, 1=w40:i16)
            n1439 = property on="2D-Intensitätsverteilung (MCP)" class="IntGraph (strikt)"("ZScale.Mapping Mode"=w40) -> ()  [unwired: 2 in, 2 out]
          }
        }
        n1440 = local read "Fehler (Ausgang)"() -> (w33:errorcluster)
        n1441 = local read "Programm beenden"() -> (w32:bool)
        n1442 = Unbundle By Name(w33) -> ("status"=w34:bool)
        n1443 = Or(x=w34, y=w32) -> (x .or. y?=w31:bool)
        n1444 = for {
          N: 1 -> [_]
          shift-right: [w36] -> w28
          shift-left: 0 -> [w37]
          n1445 = call "sub_read_LAPD.vi"() -> ("data"=w38:dbl)  [unwired: 1 in]
          n1446 = Wait (ms)(milliseconds to wait=u32 100 ("Zu wartende ms")) -> ()  [unwired: 1 out]
          n1447 = Add(x=w38, y=w37) -> (x+y=w36:dbl)
        }
        n1448 = local write "LAPD (a.u.)"(w28) -> ()
      }
    }
    frame #2 {
      n1449 = flat-sequence {
        frame #0 {
          n1450 = local read "Kamera"() -> (w1725:bool)
          n1451 = case shown="True" w1725 {
            frame #0 {
            }
            frame #1 {
              n1452 = local read "Detektionskamera"() -> (w1727:T5)
              n1453 = local read "Image Memory"() -> (w1729:T4)
              n1454 = call "camera_release configuration_stop.vi"("Image Memory"=w1729, "Detektionskamera"=w1727) -> ("error out"=w1726:errorcluster, "status"=w1728:bool)
              n1455 = local write "Kamera"(w1728) -> ()
              n1456 = local write "Fehler (Ausgang)"(w1726) -> ()
            }
          }
        }
        frame #1 {
          # "Wegen Abstürzen des Programms wird dieser Teil verhindert\nAchtung: IMMER manuell Netzteile auf 0V setzen oder HV-\nSteuerung von Hand ausmachen"
          n1457 = local read "HV-Steuerung"() -> (w1732:bool)
          n1458 = And(x=w1732, y=FALSE) -> (x .and. y?=w1730:bool)
          n1459 = case shown="True" w1730 {
            frame #0 {
            }
            frame #1 {
              n1460 = call "HV_power_supply_set_voltage.vi"("Desired output voltage in V (HV power supply)"=0.0, "Channel of HV power supply"=refnum<k21> "Dev0/Ao1") -> ("error out"=w1733:errorcluster)  [unwired: 8 in]
              n1461 = call "HV_power_supply_set_voltage.vi"("Desired output voltage in V (HV power supply)"=0.0, "Channel of HV power supply"=refnum<k21> "Dev0/Ao0") -> ("error out"=w1734:errorcluster)  [unwired: 8 in]
              n1462 = local write "Fehler (Ausgang)"(w1733) -> ()
              n1463 = local write "Fehler (Ausgang)"(w1734) -> ()
            }
          }
        }
        frame #2 {
          n1464 = local read "Wellenplatte"() -> (w1739:bool)
          n1465 = case shown="True" w1739 {
            frame #0 {
            }
            frame #1 {
              n1466 = local read "Wellenplatte [°]"() -> (w1740:refnum<k7>)
              n1467 = invoke class="MG17Motor" method="StopCtrl"(reference=w1740) -> ()  [unwired: 2 in, 3 out]
            }
          }
        }
        frame #3 {
          w1741 = FALSE ("Bühne bereit")
          w1742 = 0.0 ("Suppressor-Spannung [V]")
          n1468 = local write "Bühne"(w1741) -> ()
          n1469 = local write "Wellenplatte"(w1741) -> ()
          n1470 = local write "Spannungsscan läuft"(w1741) -> ()
          n1471 = local write "HV-Steuerung"(w1741) -> ()
          n1472 = local write "x-U-Scan läuft"(w1741) -> ()
          n1473 = local write "Waveplate ON/OFF"(w1741) -> ()
          n1474 = local write "x-U-Scan ON/OFF"(w1741) -> ()
          n1475 = local write "Programm beenden"(w1741) -> ()
          n1476 = local write "Kamera ON/OFF"(w1741) -> ()
          n1477 = local write "Leistungs-/Polarisationsscan ON/OFF"(w1741) -> ()
          n1478 = local write "Leistungs-/Polarisationscan läuft"(w1741) -> ()
          n1479 = local write "Tip-Spannung [V]"(w1742) -> ()
          n1480 = local write "Suppressor-Spannung [V]"(w1742) -> ()
        }
      }
    }
  }
  n1481 = flat-sequence {
    frame #0 {
      (unwired) 0.0 ("Helligkeitsverlauf")
      w1746 = 0.0 ("Aktuelle x-Position [mm]")
      w1752 = 1 ("# x-U-Scan Spannungsschritte")
      w1753 = 0.0 ("Aktuelle x-Position [mm]")
      w1751 = 0.0 ("Suppressor-Spannung [V]")
      w1743 = i64 0 ("Numerisches Element")
      w1765 = u16 3 items=["1000", "500", "200", "100", "50", "20", "10"] ("Shutter time (ms)")
      w1744 = FALSE ("Scanstart")
      n1482 = Initialize Array(1 ("Element"), 2 ("Dimension")) -> (w1754:i32[])
      n1483 = Initialize Array(1 ("Dimension"), 3 ("Dimension")) -> (w1777:i32[])
      n1484 = Initialize Array(0.0 ("Element"), 2 ("Dimension")) -> (w1750:dbl[])
      "Aktuelle Spannung [V]" <- w1750
      "Spannungsstart [V]" <- w1750
      "x-U-Scan (Ausgleichslage) xy-Start [mm]" <- w1750
      "x-U-Scan (Ausgleichslage) xy-End [mm]" <- w1750
      n1485 = Initialize Array(0.0 ("Element"), 3 ("Dimension")) -> (w1760:dbl[])
      "Aktuelle xyz-Position [mm]" <- w1760
      "Start xyz-Position [mm]" <- w1760
      "Rasterschritt [µm]" <- w1760
      n1486 = local write "Tip-Spannung [V]"(0.0 ("Tip-Spannung [V]")) -> ()
      n1487 = local write "# Photosignale"(10.0 ("Anzahl Mittelungen")) -> ()
      n1488 = local write "x-U-Scan x-Rasterweite [µm]"(w1751) -> ()
      n1489 = local write "# x-U-Scan x-Rasterschritte"(w1752) -> ()
      n1490 = local write "x-U-Scan Spannungsweite [V]"(w1751) -> ()
      n1491 = local write "# x-U-Scan Spannungsschritte"(w1752) -> ()
      n1492 = local write "Suppressor-Spannung [V]"(w1751) -> ()
      n1493 = local read "Aktueller Messschritt"() -> (w1770:i32)
      n1494 = local write "Shutter time (ms)"(w1765) -> ()
      n1495 = local write "# Spannungsschritte"(w1754) -> ()
      n1496 = local write "Spannungsweite [V]"(w1750) -> ()
      n1497 = local write "Rasterweite [µm]"(w1760) -> ()
      n1498 = local write "# Rasterschritte"(w1777) -> ()
      n1499 = local write "ROI"(i32[] [640, 480, 0, 0] ("Region of Interest (px)")) -> ()
      n1500 = local write "x-U-Scan (Ausgleichslage) Steigung"(0.0 ("x-U-Scan (Ausgleichslage) Steigung")) -> ()
      n1501 = local write "Spannungsscan ON/OFF"(w1744) -> ()
      n1502 = local write "Programm beenden"(w1744) -> ()
      n1503 = local write "Spannungsscan ON/OFF"(w1744) -> ()
      n1504 = local write "Sequenzaufnahme ON"(w1744) -> ()
      n1505 = local write "HV ON/OFF"(w1744) -> ()
      n1506 = local write "x-U-Scan ON/OFF"(w1744) -> ()
      n1507 = local write "Kamera ON/OFF"(w1744) -> ()
      n1508 = local write "Rasterung ON/OFF"(w1744) -> ()
      n1509 = local write "Waveplate ON/OFF"(w1744) -> ()
      n1510 = local write "Buffer Overrun"(w1744) -> ()
      n1511 = local write "x-U-Scan läuft"(w1744) -> ()
      n1512 = local write "Rasterung läuft"(w1744) -> ()
      n1513 = Create User Event(user event datatype=w1770) -> (user event=→"Event: Rasterung gestartet?":refnum<user-event>)  [unwired: 1 in, 1 out]
      n1514 = local write "Leistungs-/Polarisationsscan ON/OFF"(w1744) -> ()
      n1515 = local write "Hintergrund-Helligkeit"(w1743) -> ()
      "Rasterung läuft" <- FALSE ("Scan aktiv")
      "# Messschritte" <- 0 ("# Messschritte")
      "Aktueller Messschritt" <- 0 ("Aktueller Messschritt")
      "x-Achse" <- 1 ("x-Achse")
      "y-Achse" <- 2 ("y-Achse")
      "z-Achse" <- 3 ("z-Achse")
      "Summierte Helligkeit (a.u.)" <- w1743
      "LAPD Spannung (V)" <- 0.0 ("Transmittierte Intensität (a.u.)")
      "Bühne" <- w1744
      "Wellenplatte" <- w1744
      "Kamera" <- FALSE ("Camera eingeschaltet")
      "HV-Steuerung" <- w1744
      "Spannungsscan läuft" <- w1744
      "x-U-Scan aktuelle x-Position [mm]" <- w1753
      "x-U-Scan x-Rasterschritt [µm]" <- w1753
      "x-U-Scan aktuelle Spannung [V]" <- w1753
      "x-U-Scan Spannungsschritt [V]" <- w1753
      "x-U-Scan x-Startposition [mm]" <- w1753
      "x-U-Scan Spannungsstart [V]" <- w1751
      "x-U-Scan aktuelle y-Position [mm]" <- 0.0 ("x-U-Scan aktuelle y-Position [mm]")
      "x-U-Scan y-Startposition [mm]" <- 0.0 ("x-U-Scan y-Startposition [mm]")
      "L/2-Schritt [°]" <- w1746
      "Aktuelle L/2-Position [°]" <- w1746
      "Aktuelle Leistung (iK) [mW]" <- w1746
      "Leistungs-/Polarisationscan läuft" <- w1744
      "Leist/Pol # Schleifen" <- i64 1 ("Leist/Pol # Schleifen")
      "Daten speichern" <- w1744
    }
  }
